vi "TC.vi"() -> ()   [LabVIEW 2019]
uses:
  Lib/Lib.llb/CS mode.ctl
  Lib/Lib.llb/R.ctl
  Lib/Lib.llb/T.ctl
  Lib/Lib.llb/Calibrations.ctl
  Lib/Lib.llb/CS.lvclass
  Lib/Lib.llb/PID Settings.ctl
  Lib/Lib.llb/AVS_exc_n_ranges.ctl
  Lib/Lib.llb/AVS_excitation.ctl
  Lib/Lib.llb/AVS47_range.ctl
  Lib/Lib.llb/Ch descriptions.ctl
  Lib/Lib.llb/Cursor Controls.ctl
  Lib/Lib.llb/DataArray.ctl
  Lib/Lib.llb/Unit.ctl
  Lib/Lib.llb/Control 6.ctl
  Lib/Lib.llb/Control 4.ctl
  Lib/Lib.llb/Control 8.ctl
  Lib/Lib.llb/VI FPO Ref.ctl
  Lib/support/Class ID ENUM.ctl
  <userlib>/_OpenG.lib/lvdata/lvdata.llb/Type Descriptor Enumeration__ogtk.ctl
  <userlib>/_OpenG.lib/lvdata/lvdata.llb/Refnum Subtype Enum__ogtk.ctl
  <userlib>/_OpenG.lib/lvdata/lvdata.llb/Waveform Subtype Enum__ogtk.ctl
  Lib/Lib.llb/LV Data cluster.ctl
  <userlib>/LevyLab/Instrument Framework/Instrument/Typedefs/PublicEvents--Instrument.MessageFromProcess.ctl
  <userlib>/LevyLab/RemoteControl/RemoteControl/Typedefs/Message--Cluster.ctl
  shared/Inst.TC/Inst.TC.lvclass
  C:/Program Files (x86)/National Instruments/LabVIEW 2019/vi.lib/JKI/JKI SMO/SMO/SMO.lvclass
  C:/Program Files (x86)/National Instruments/LabVIEW 2019/user.lib/LevyLab/Instrument Framework/Instrument/Instrument.lvclass
  Lib/Lib.llb/Action.ctl
  <userlib>/LevyLab/Instrument Framework/Instrument Types/Cryostat/Typedefs/setHeater--cluster.ctl
  shared/Inst.TC/Typedefs/Inst.TC.Commands--Enum.ctl
  Lib/Lib.llb/TCS.lvclass
  C:/Users/ansom/Documents/Girthub/Leiden-FP-and-TC/src/TC/1. Sources/Lib/Lib.llb/CS.lvclass
  Lib/Lib.llb/QCS.lvclass
  Lib/Lib.llb/CS Emulation.lvclass
  Lib/Lib.llb/PCS.lvclass
  Lib/Lib.llb/Byte Params.ctl
  8b3f8898-ff02-46d6-8412-899a53daf4d1.vi
  <vilib>/JDP Science/JSONtext/JSON text to Variant.vi
  <userlib>/LevyLab/Instrument Framework/Instrument/API/Instrument.sendMessageToProcess (string).vi
  <vilib>/JDP Science/JSONtext/LVClass Serializer/JSONtext LVClass Serializer.lvclass
  Lib/Lib.llb/MView.lvlib
  <userlib>/LevyLab/Instrument Framework/Instrument Types/Cryostat/Instrument.Cryostat.lvclass
  <vilib>/JKI/JKI SMO/SMO/SMO.lvclass
  <userlib>/LevyLab/Instrument Framework/Instrument/Instrument.lvclass
  C:/Program Files (x86)/National Instruments/LabVIEW 2019/user.lib/LevyLab/Instrument Framework/Instrument Types/Cryostat/Instrument.Cryostat.lvclass
  <userlib>/LevyLab/RemoteControl/RemoteControl/RemoteControl.lvclass
panel:
  out "R Array":dbl[](array[numeric])
  out "_SetControl":T1
  out "ControlNames":string[](array[string])
  out "VIRef":T2 {"Array DataType" format="%.0x"; "WaveForm Type" format="%.0x"; "RefNum Type" format="%.0x"; "DataType" format="%.0x"}
  out "VI called?":bool=TRUE
  out "Error code":u8
  out "_zBridgeSetNr":u8 caption="zBridge set nr."
  out "_zBridgeDll":path=path "C:/Users/Sasha/Dropbox/Labview/LC Software/ImpSoft-V5.2.2-multithreaded/ImpBridgeLabview/ImpBridgeDll.dll"
  in  "_String":string="^ Click the Run button to start the program "
  in  "Top Toolbar":enum32{"Page 1", "Page 2"}(tab)
  in  "Load config":bool
  in  "Start":bool
  in  "Load Data":bool
  in  "Pause":bool
  in  "Stop":bool
  in  "Copy to Clipboard":bool
  in  "Save config":bool
  in  "Clear all plots":bool
  in  "ColorBox":enum32{"Page 1", "Page 2"}(tab)
  in  "Colors":picture
  out "Color":u32(colorbox)
  in  "Graph-open popup":bool
  out "_CalibFilesPath":path=path "C:/avs-47/aaaa"
  out "_LogFilesPath":path
  out "_AVS_VISA":refnum<visa-resource-name>="COM3"
  in  "Minimize UI 2":bool
  out "VI Version":string="TC" caption="V"
  in  "Minimize UI 1":bool
  in  "Main Panel":enum32{"AVS"}(tab)
  in  "Graph Controls Bar":enum32{"Page 1"}(tab)
  in  "Mode Buttons":T7
  in  "Erase all":bool
  in  "Plot-Save All":bool
  in  "Plot-save-screen":bool
  in  "Channels Panel":T8(tab)=enum."All"
  out "T0":dbl=nan caption="T" format="%#.2p"
  out "R0":dbl caption="R" format="%.3p"
  out "R-Plot 0":cluster{dbl[], dbl[]}(graph) caption="R-Plot"
  out "T1":dbl=nan caption="T" format="%#.2p"
  out "R1":dbl caption="R" format="%.3p"
  out "R-Plot 1":cluster{dbl[], dbl[]}(graph) caption="R-Plot"
  out "T2":dbl=nan caption="T" format="%#.2p"
  out "R2":dbl caption="R" format="%.3p"
  out "R-Plot 2":cluster{dbl[], dbl[]}(graph) caption="R-Plot"
  out "T3":dbl=nan caption="T" format="%#.2p"
  out "R3":dbl caption="R" format="%.3p"
  out "R-Plot 3":cluster{dbl[], dbl[]}(graph) caption="R-Plot"
  out "T4":dbl=nan caption="T" format="%#.2p"
  out "R4":dbl caption="R" format="%.3p"
  out "R-Plot 4":cluster{dbl[], dbl[]}(graph) caption="R-Plot"
  out "T5":dbl=nan caption="T" format="%#.2p"
  out "R5":dbl caption="R" format="%.3p"
  out "R-Plot 5":cluster{dbl[], dbl[]}(graph) caption="R-Plot"
  out "T6":dbl=nan caption="T" format="%#.2p"
  out "R6":dbl caption="R" format="%.3p"
  out "R-Plot 6":cluster{dbl[], dbl[]}(graph) caption="R-Plot"
  out "T7":dbl=nan caption="T" format="%#.2p"
  out "R7":dbl caption="R" format="%.3p"
  out "R-Plot 7":cluster{dbl[], dbl[]}(graph) caption="R-Plot"
  out "T8":dbl=nan caption="T" format="%#.2p"
  out "R8":dbl caption="R" format="%.3p"
  out "R-Plot 8":cluster{dbl[], dbl[]}(graph) caption="R-Plot"
  out "T9":dbl=nan caption="T" format="%#.2p"
  out "R9":dbl caption="R" format="%.3p"
  out "R-Plot 9":cluster{dbl[], dbl[]}(graph) caption="R-Plot"
  out "T Cluster":T9 {"T9" format="%.2p"; "T8" format="%.2p"; "T7" format="%.2p"; "T6" format="%.2p"; "T5" format="%.2p"; "T4" format="%.2p"; "T3" format="%.2p"; "T2" format="%.2p"; "T1" format="%.2p"; "T0" format="%.2p"}
  in  "Sensor Names":T10={"AVS Name 0"="C_still", "AVS Name 1"="3K", "AVS Name 2"="Still", "AVS Name 3"="50mK", "AVS Name 4"="MC", "AVS Name 5"="MC", "AVS Name 6"="MC", "AVS Name 7"="", "AVS Name 8"="", "AVS Name 9"=""}
  in  "Edit Calibrations":T11
  in  "Sensor Calibrations":T12 {"Sensor 10" items=["PT100", "PT1000", "RuO2 2k", "Emulation R", "PT 1000", "RuO2-10K-NEW", "RuO2-10K", "RuO2-1k5", "TT-1338", "TT-1340", "TT-1342", "TT-1346", "TT-1349", "TT-1392", "CMN-187", "testCMN", "No Calibration"]; "Sensor 9" items=["PT100", "PT1000", "RuO2 2k", "Emulation R", "PT 1000", "RuO2-10K-NEW", "RuO2-10K", "RuO2-1k5", "TT-1338", "TT-1340", "TT-1342", "TT-1346", "TT-1349", "TT-1392", "CMN-187", "testCMN", "No Calibration"]; "Sensor 8" items=["PT100", "PT1000", "RuO2 2k", "Emulation R", "PT 1000", "RuO2-10K-NEW", "RuO2-10K", "RuO2-1k5", "TT-1338", "TT-1340", "TT-1342", "TT-1346", "TT-1349", "TT-1392", "CMN-187", "testCMN", "No Calibration"]; "Sensor 7" items=["PT100", "PT1000", "RuO2 2k", "Emulation R", "PT 1000", "RuO2-10K-NEW", "RuO2-10K", "RuO2-1k5", "TT-1338", "TT-1340", "TT-1342", "TT-1346", "TT-1349", "TT-1392", "CMN-187", "testCMN", "No Calibration"]; "Sensor 6" items=["PT100", "PT1000", "RuO2 2k", "Emulation R", "PT 1000", "RuO2-10K-NEW", "RuO2-10K", "RuO2-1k5", "TT-1338", "TT-1340", "TT-1342", "TT-1346", "TT-1349", "TT-1392", "CMN-187", "testCMN", "No Calibration"]; "Sensor 5" items=["PT100", "PT1000", "RuO2 2k", "Emulation R", "PT 1000", "RuO2-10K-NEW", "RuO2-10K", "RuO2-1k5", "TT-1338", "TT-1340", "TT-1342", "TT-1346", "TT-1349", "TT-1392", "CMN-187", "testCMN", "No Calibration"]; "Sensor 4" items=["PT100", "PT1000", "RuO2 2k", "Emulation R", "PT 1000", "RuO2-10K-NEW", "RuO2-10K", "RuO2-1k5", "TT-1338", "TT-1340", "TT-1342", "TT-1346", "TT-1349", "TT-1392", "CMN-187", "testCMN", "No Calibration"]; "Sensor 3" items=["PT100", "PT1000", "RuO2 2k", "Emulation R", "PT 1000", "RuO2-10K-NEW", "RuO2-10K", "RuO2-1k5", "TT-1338", "TT-1340", "TT-1342", "TT-1346", "TT-1349", "TT-1392", "CMN-187", "testCMN", "No Calibration"]; "Sensor 2" items=["PT100", "PT1000", "RuO2 2k", "Emulation R", "PT 1000", "RuO2-10K-NEW", "RuO2-10K", "RuO2-1k5", "TT-1338", "TT-1340", "TT-1342", "TT-1346", "TT-1349", "TT-1392", "CMN-187", "testCMN", "No Calibration"]; "Sensor 1" items=["PT100", "PT1000", "RuO2 2k", "Emulation R", "PT 1000", "RuO2-10K-NEW", "RuO2-10K", "RuO2-1k5", "TT-1338", "TT-1340", "TT-1342", "TT-1346", "TT-1349", "TT-1392", "CMN-187", "testCMN", "No Calibration"]}
  out "Units":T13
  out "R Cluster":T14={"R0"=0.0, "R1"=0.0, "R2"=-0.0, "R3"=0.0, "R4"=0.0, "R5"=0.0, "R6"=0.0, "R7"=0.0, "R8"=0.0, "R9"=0.0} {"R9" format="%.3p"; "R8" format="%.3p"; "R7" format="%.3p"; "R6" format="%.3p"; "R5" format="%.3p"; "R4" format="%.3p"; "R3" format="%.3p"; "R2" format="%.3p"; "R1" format="%.3p"; "R0" format="%.3p"}
  in  "AVS Scan Parameters":enum32{"Page 1", "Page 2"}(tab)
  in  "AVS Exc&Ranges":T15={"Excitation 0"=4, "Excitation 1"=4, "Excitation 2"=3, "Excitation 3"=3, "Excitation 4"=3, "Excitation 5"=3, "Excitation 6"=3, "Excitation 7"=3, "Range 0"=5, "Range 1"=5, "Range 2"=5, "Range 3"=5, "Range 4"=5, "Range 5"=5, "Range 6"=5, "Range 7"=5} {"Range 7" items=["n.a."=-1, "open"=0, "2 Ohm"=1, "20 Ohm"=2, "200 Ohm"=3, "2k Ohm"=4, "20k Ohm"=5, "200k Ohm"=6, "2M Ohm"=7]; "Range 6" items=["n.a."=-1, "open"=0, "2 Ohm"=1, "20 Ohm"=2, "200 Ohm"=3, "2k Ohm"=4, "20k Ohm"=5, "200k Ohm"=6, "2M Ohm"=7]; "Range 5" items=["n.a."=-1, "open"=0, "2 Ohm"=1, "20 Ohm"=2, "200 Ohm"=3, "2k Ohm"=4, "20k Ohm"=5, "200k Ohm"=6, "2M Ohm"=7]; "Range 4" items=["n.a."=-1, "open"=0, "2 Ohm"=1, "20 Ohm"=2, "200 Ohm"=3, "2k Ohm"=4, "20k Ohm"=5, "200k Ohm"=6, "2M Ohm"=7]; "Range 3" items=["n.a."=-1, "open"=0, "2 Ohm"=1, "20 Ohm"=2, "200 Ohm"=3, "2k Ohm"=4, "20k Ohm"=5, "200k Ohm"=6, "2M Ohm"=7]; "Range 2" items=["n.a."=-1, "open"=0, "2 Ohm"=1, "20 Ohm"=2, "200 Ohm"=3, "2k Ohm"=4, "20k Ohm"=5, "200k Ohm"=6, "2M Ohm"=7]; "Range 1" items=["n.a."=-1, "open"=0, "2 Ohm"=1, "20 Ohm"=2, "200 Ohm"=3, "2k Ohm"=4, "20k Ohm"=5, "200k Ohm"=6, "2M Ohm"=7]; "Range 0" items=["n.a."=-1, "open"=0, "2 Ohm"=1, "20 Ohm"=2, "200 Ohm"=3, "2k Ohm"=4, "20k Ohm"=5, "200k Ohm"=6, "2M Ohm"=7]; "Excitation 7" items=["none", "3 µV", "10 µV", "30 µV", "100 µV", "300 µV", "1 mV", "3 mV"]; "Excitation 6" items=["none", "3 µV", "10 µV", "30 µV", "100 µV", "300 µV", "1 mV", "3 mV"]; "Excitation 5" items=["none", "3 µV", "10 µV", "30 µV", "100 µV", "300 µV", "1 mV", "3 mV"]; "Excitation 4" items=["none", "3 µV", "10 µV", "30 µV", "100 µV", "300 µV", "1 mV", "3 mV"]; "Excitation 3" items=["none", "3 µV", "10 µV", "30 µV", "100 µV", "300 µV", "1 mV", "3 mV"]; "Excitation 2" items=["none", "3 µV", "10 µV", "30 µV", "100 µV", "300 µV", "1 mV", "3 mV"]; "Excitation 1" items=["none", "3 µV", "10 µV", "30 µV", "100 µV", "300 µV", "1 mV", "3 mV"]; "Excitation 0" items=["none", "3 µV", "10 µV", "30 µV", "100 µV", "300 µV", "1 mV", "3 mV"]}
  out "zBridge.Scan Phase":T18
  out "zBridge params":T19
  out "uPlots":T20
  out "zBridge.Active Channels":T21={"active Channel 0"=TRUE, "active Channel 1"=TRUE, "active Channel 2"=TRUE, "active Channel 3"=FALSE, "active Channel 4"=FALSE, "active Channel 5"=FALSE, "active Channel 6"=FALSE, "active Channel 7"=FALSE, "active Channel 8"=FALSE, "active Channel 9"=FALSE}
  out "Waveform Chart":T22(graph)
  in  "_CS_Address":u32
  in  "Edit calibration":bool
  in  "Convert R-T":bool
  out "T7":dbl caption="T=" format="%#.2p"
  in  "QuickR":dbl caption="R=" format="%_6g"
  in  "_QuickConvertCal":u16(ring) items=["PT100", "PT1000", "RuO2 2k", "Emulation R", "PT 1000", "RuO2-10K-NEW", "RuO2-10K", "RuO2-1k5", "TT-1338", "TT-1340", "TT-1342", "TT-1346", "TT-1349", "TT-1392", "CMN-187", "testCMN", "No Calibration"]
  out "_CSMode1List[i]":T23[](array[typedef]) caption="I_list[i]" min=-1.0
  out "CS.Automode Current":T23[](array[typedef]) min=-1.0
  in  "Lower Panel":enum32{"Page 1", "Page 2"}(tab)
  in  "Data History/RT Settings":enum32{"History", "Settings"}(tab)=enum."Settings"
  out "AVS names small":T10={"AVS Name 0"="3K", "AVS Name 1"="Still", "AVS Name 2"="50 mK", "AVS Name 3"="MC", "AVS Name 4"="MC", "AVS Name 5"="", "AVS Name 6"="", "AVS Name 7"="", "AVS Name 8"="", "AVS Name 9"=""}
  out "zBridge.Active channel":T24
  out "Small T Cluster":T25 caption="T" {"T0" format="%#.2p"; "T1" format="%#.2p"; "T2" format="%#.2p"; "T3" format="%#.2p"; "T4" format="%#.2p"; "T5" format="%#.2p"; "T6" format="%#.2p"; "T7" format="%#.2p"; "T8" format="%#.2p"; "T9" format="%#.2p"}
  out "Small R Cluster":T26 caption="R" {"R0" format="%#_5p"; "R1" format="%#_5p"; "R2" format="%#_5p"; "R3" format="%#_5p"; "R4" format="%#_5p"; "R5" format="%#_5p"; "R6" format="%#_5p"; "R7" format="%#_5p"; "R8" format="%#_5p"; "R9" format="%#_5p"}
  out "Time":dbl format="%<%X\n%x>T"
  in  "Runtime Settings":T27={"Read AVS channels from"=0, "Last Channel"=7, "Delay Between Scans"=0, "Stabilisation Delay"=5.0, "Averages"=2, "Data Memory"=25000, "Filter Graphs"=FALSE, "Y_min"=0.0, "Y_max"=2000000.0, "Plot type"=enum."T vs Time", "Allow neg R"=TRUE, "Miniplot Time"=30.0} {"Miniplot Time" min=0.0; "Delay Between Scans" format="%.0f s"; "Averages" min=1 max=1000; "Stabilisation Delay" min=0.5; "Last Channel" min=0 max=7 step=1; "Read AVS channels from" min=0 max=7 step=1; "Y_max" format="%#_6f"; "Y_min" min=0.0 format="%#_6f"; "Data Memory" min=3 max=50000}
  out "CS.Current Value":dbl[](array[numeric])
  in  "Data Array":T28=[{"R"=[], "T"=[], "Time"=[]}, {"R"=[0.0, 2.0], "T"=[], "Time"=[]}]
  out "T Array":dbl[](array[numeric])
  in  "_ScanData":dbl[](array[numeric])
  out "_I3SetPnt":dbl
  out "_CurrentsChanged":bool
  in  "_AVSRanges":T29={"Excitationl 0"=5, "Excitation 1"=5, "Excitation 2"=5, "Excitation 3"=5, "Excitation 4"=5, "Excitation 5"=5, "Excitation 6"=5, "Excitation 7"=5} caption="Ranges" {"Excitation 7" items=["n.a."=-1, "open"=0, "2 Ohm"=1, "20 Ohm"=2, "200 Ohm"=3, "2k Ohm"=4, "20k Ohm"=5, "200k Ohm"=6, "2M Ohm"=7]; "Excitation 6" items=["n.a."=-1, "open"=0, "2 Ohm"=1, "20 Ohm"=2, "200 Ohm"=3, "2k Ohm"=4, "20k Ohm"=5, "200k Ohm"=6, "2M Ohm"=7]; "Excitation 5" items=["n.a."=-1, "open"=0, "2 Ohm"=1, "20 Ohm"=2, "200 Ohm"=3, "2k Ohm"=4, "20k Ohm"=5, "200k Ohm"=6, "2M Ohm"=7]; "Excitation 4" items=["n.a."=-1, "open"=0, "2 Ohm"=1, "20 Ohm"=2, "200 Ohm"=3, "2k Ohm"=4, "20k Ohm"=5, "200k Ohm"=6, "2M Ohm"=7]; "Excitation 3" items=["n.a."=-1, "open"=0, "2 Ohm"=1, "20 Ohm"=2, "200 Ohm"=3, "2k Ohm"=4, "20k Ohm"=5, "200k Ohm"=6, "2M Ohm"=7]; "Excitation 2" items=["n.a."=-1, "open"=0, "2 Ohm"=1, "20 Ohm"=2, "200 Ohm"=3, "2k Ohm"=4, "20k Ohm"=5, "200k Ohm"=6, "2M Ohm"=7]; "Excitation 1" items=["n.a."=-1, "open"=0, "2 Ohm"=1, "20 Ohm"=2, "200 Ohm"=3, "2k Ohm"=4, "20k Ohm"=5, "200k Ohm"=6, "2M Ohm"=7]; "Excitationl 0" items=["n.a."=-1, "open"=0, "2 Ohm"=1, "20 Ohm"=2, "200 Ohm"=3, "2k Ohm"=4, "20k Ohm"=5, "200k Ohm"=6, "2M Ohm"=7]}
  out "_CSClassRef":refnum<class "CS.lvclass">
  in  "CS Indicators Panel":enum32{"Page 1", "Page 2"}(tab)
  out "CS.Automode 0":bool
  out "CS.Automode 1":bool
  out "QCS. I0 Mapping":T30(ring) caption="Output to"
  in  "uA 0":u32
  in  "CS Cannel Names":T31={"CS Name 0"="N.C.", "CS Name 1"="3K", "CS Name 2"="Still", "CS Name 3"="MC"}
  out "I0":T32={"uA"="000", "ON"=FALSE, "Gated"=FALSE, "current flows"=FALSE, "Error"=FALSE} caption="Ch0 -"
  in  "uA 3":u32
  in  "uA 2":u32
  in  "uA 1":u32
  out "CS.Automode 3":bool
  out "CS.Automode 2":bool
  out "I3":T32={"uA"="000", "ON"=FALSE, "Gated"=FALSE, "current flows"=FALSE, "Error"=FALSE} caption="Chn 3"
  out "I2":T32={"uA"="000", "ON"=FALSE, "Gated"=FALSE, "current flows"=FALSE, "Error"=FALSE} caption="Chn 2"
  out "I1":T32={"uA"="000", "ON"=FALSE, "Gated"=FALSE, "current flows"=FALSE, "Error"=FALSE} caption="Chn 1"
  out "_ExtVIReference":refnum<vi>
  out "Small I":cluster{"I1":dbl, "I2":dbl, "I3":dbl, "I4":dbl} caption="I" {"I1" format="%#.2f"; "I2" format="%#.2p"; "I3" format="%#.2p"; "I4" format="%#.2p"}
  out "CS.Actual Current":dbl[](array[numeric])
  in  "Save Data 2":bool
  in  "Show PID graph?":bool
  in  "Set Color":bool
  out "_ZBridgeUnit":string caption="Unit"
  out "_zBridgeParText":string caption="zBridge params/Error"
  out "_CurCalibrations":T33
  out "_LMBDown":bool
  in  "Side Panel":T34(tab)
  in  "Reload Calibrations":bool
  in  "zBridge settings":bool
  out "CS.ID":string caption="ID"
  out "CS status":errorcluster
  out "General Error":errorcluster caption="General status"
  in  "Bridge settings":T35={"Bridge Type"=enum."AVS47A (GPIB interface)", "AVS RS232 Port"="COM5", "AVS GPIB Address"="GPIB0::20::INSTR", "Calibrations Folder"=path "C:/LC Data/Calibrations", "Picobus Delay"=1, "Sync to ADC"=enum."TRUE"} {"Picobus Delay" max=1000000 step=1}
  in  "CS Settings":T36={"TCS RS232 Port"="COM1", "TCS_Imax"=5, "CS type"=enum."TCS", "CS.QCS Device Nr"=0}
  in  "Data Logging Settings":T37={"Log Files Folder"=path "C:/LC Data/Data", "Log Files Name"="LogAVS", "Automode Files Name"="calibration", "Filenames Suffix"="_%Y-%m-%d-%H-%M-%S", "Delimeter"="\t", "New File Interval"=7, "New File Interval Units"=enum."Days", "Date Format"="%Y-%m-%d %H:%M:%S", "External VI Path"=path "", "Query Description"=FALSE, "Run Description"="\n"}
  out "Bridge status":errorcluster
  in  "CS.QCS I0 Output":T38(ring) caption="Set Channel 0 output to"
  in  "CS.Mode":T39 caption="CS mode"
  out "_TimeOld":dbl format="%#_16g"
  in  "CS Modes Panel":T40(tab)=enum."Automatic 1"
  in  "CS.I3":T41={"Toggle ON/OFF"=FALSE, "Toggle Gated"=FALSE, "I"=0, "Range"=enum."x1 uA"} caption="Chn 3" {"I" max=100000 step=1}
  in  "CS.I2":T41={"Toggle ON/OFF"=FALSE, "Toggle Gated"=FALSE, "I"=0, "Range"=enum."x1 uA"} caption="Chn 2" {"I" max=100000 step=1}
  in  "CS.I1":T41={"Toggle ON/OFF"=FALSE, "Toggle Gated"=FALSE, "I"=0, "Range"=enum."x1 uA"} caption="Chn 1" {"I" max=100000 step=1}
  in  "CS.I0":T41={"Toggle ON/OFF"=FALSE, "Toggle Gated"=FALSE, "I"=0, "Range"=enum."x1 uA"} caption="Chn 0" {"I" max=100000 step=1}
  in  "CS.Mode1.PID Settings":T42={"FB on 2"=enum."3", "Proportional Gain"=3.0, "Integral Gain"=3.0, "Derivative Gain"=1.0, "Deadband"=0.1, "Feed Fwd Gain [uA/mK]"=0.0, "Integral Gain Bandwidth"=10.0, "Integral Gain Background"=1.0, "Current limit, [uA]"=1.0} {"Integral Gain Background" format="%#.6g"; "Integral Gain Bandwidth" format="%#.6g"; "Feed Fwd Gain [uA/mK]" format="%#.5g"; "Deadband" format="%#.5g"; "Derivative Gain" format="%#.6g"; "Integral Gain" format="%#.6g"; "Proportional Gain" format="%#.6g"; "Current limit, [uA]" format="%#.5g"}
  in  "CS.Mode1.Start":bool
  in  "CS.Mode1.List":T23[][](array[typedef]) min=-1.0
  out "CS.Mode1.PID Column":T43[](array[typedef])
  out "CS.Mode1.Row":T44[](array[typedef])=[TRUE, FALSE, FALSE, FALSE, FALSE, FALSE, FALSE, FALSE, FALSE, FALSE]
  out "CS.Mode1.PID Stabilized?":bool caption="SP reached?"
  out "CS.Mode1.PID Error":dbl=10.0 caption="Error" format="%#_6f"
  out "CS.Mode1.Slope":dbl caption="Slope" format="%#_3g %"
  out "CS.Mode1.Timer":dbl caption="Timer" format="%<%H:%M:%S>t"
  out "CS.Mode1.List:Count":i32=10 caption="/"
  out "CS.Mode1.List:Index":i32=10 caption="Point #"
  in  "CS.Mode1.Next":bool
  in  "CS.Mode1.Reset PID":bool
  in  "CS.Mode1.Auto Advance":bool=TRUE caption="Enable automatic sweeping/list iteration"
  in  "CS.Mode1.Settings":T45={"Bridge Channel"=0, "N averages"=10, "Delay Time"=10.0, "T stability"=0.3, "FB on"=enum."Temperature"} {"Delay Time" min=0.0 format="%#_g min"; "Bridge Channel" min=-1 max=9 step=1}
  in  "CS.Mode1.Call VI?":bool caption="Call Ext. VI"
  out "CS.Mode1.VI State":T46(ring) caption="- state"
  in  "CS.Mode1.Trigger all TC":bool caption="Trigger other running TC instances"
  in  "CS.Mode1.List:Prev":bool
  in  "CS.Mode1.List:Next":bool
  in  "CS.Mode1.List:To First":bool
  in  "CS.Mode1.List:Save":bool
  in  "CS.Mode1.List:Load":bool
  in  "CS.Mode1.Write To Log":bool
  in  "CS.Mode1.PID":cluster{"Enabled":bool}
  in  "CS.Mode1.List:Clear":bool
  in  "CS.Mode2.Settings":T47={"FB on"=enum."Temperature", "Bridge Channel"=0, "Hysteresis"=10} {"Hysteresis" max=100 format="%.0f %%"; "Bridge Channel" min=-1 max=9 step=1}
  in  "CS.Mode2.Start":bool
  in  "CS.Mode2.Add Row":bool
  in  "CS.Mode2.New Row":dbl[](array[numeric])=[0.0, 0.0, 0.0, 0.0, 0.0, 0.0] caption="New range" min=-1.0
  in  "CS.Mode2.List":dbl[][](array[numeric])=[[0.0, 0.0, 0.0, 0.0, 0.0, inf]] min=-1.0
  out "CS.Mode2.Row":T44[](array[typedef])=[TRUE, FALSE, FALSE, FALSE, FALSE, FALSE, FALSE, FALSE, FALSE, FALSE]
  in  "T Sweep":T48={"Start value"=200.0, "End value"=250.0, "Step"=10.0, "Current"=0.0, "I_next"=FALSE, "I_prev"=FALSE, "Interrrupt Sweep"=FALSE, "Start"=FALSE, "Boolean"=TRUE} {"Step" min=0.0; "End value" min=0.0; "Start value" min=0.0}
  # "Quick convert R->T:"
  # "Ohm"
  # "mK"
  # "Ch#"
  # "Miniplot"
  # "Channel parameters"
  # "Impedance"
  # "Unit"
  # "Type of sensor"
  # "T [mK]"
  # "Description"
  # "0"
  # "1"
  # "2"
  # "3"
  # "4"
  # "5"
  # "6"
  # "7"
  # "8"
  # "9"
  # "0"
  # "1"
  # "2"
  # "3"
  # "4"
  # "5"
  # "7"
  # "8"
  # "9"
  # "6"
  # "auto"
  # "auto"
  # "auto"
  # "auto"
  # "gated"
  # "gated"
  # "gated"
  # "gated"
  # "Status"
  # "Current source mode"
  # "Current source manual control"
  # "Current source automatic mode #1"
  # "Currents List"
  # "Settings"
  # "I0"
  # "I1"
  # "I2"
  # "I3"
  # "Status"
  # "On temperature stabilized"
  # "Current source automatic mode #2"
  # "Currents List"
  # "Settings"
  # "T0"
  # "T1"
  # "I0"
  # "I1"
  # "I2"
  # "I3"
  # "T0"
  # "T1"
  # "I0"
  # "I1"
  # "I2"
  # "I3"
  # "Ch3"
types:
  T1 = typedef "MView.lvlib/LV Data cluster.ctl" = cluster{"Name":string, "Scalar":string, "Array":string[][]}
  T2 = typedef "MView.lvlib/VI FPO Ref.ctl" = cluster{"Control Ref ID":refnum<vi>[], "Full Name":string[], "ClassID":T3[], "Short Name":string[], "DataType":T4[], "RefNum Type":T5[], "WaveForm Type":T6[], "Parent":i32[], "Array DataType":T4[], "Owning VI":refnum<vi>[], "Active?":bool[]}
  T3 = typedef "Class ID ENUM.ctl" = enum16{"<Null>", "1", "2", "Generic", "Decoration", "Text", "Control", "ColorBox", "Boolean", "RefNum", "Variant", "Path", "ListBox", "Table", "Array", "Picture", "ActiveXContainer", "Numeric", "Digital", "NamedNumeric", "ColorRamp", "Slide", "GraphOrChart", "WaveformChart", "WaveformGraph", "IntensityChart", "IntensityGraph", "String", "IOName", "ComboBox", "Cluster", "Panel", "Knob", "NumWithScale", "Ring", "Enum", "GObject", "Plot", "Cursor", "NumericText", "Scale", "ColorScale", "GraphScale", "ColorGraphScale", "TypedRefNum", "OldKnobScale", "MCListbox", "MeasureData", "BVTag", "DAQName", "VISAName", "IVIName", "SlideScale", "TabControl", "Page", "TabArrayTabControl", "ConPane", "57", "58", "59", "60", "61", "62", "63", "64", "SubPanel", "TreeControl", "67", "68", "69", "70", "71", "72", "73", "74", "75", "SplitterBar"}
  T4 = typedef "Type Descriptor Enumeration__ogtk.ctl" = enum8{"<Null>", "I8", "I16", "I32", "I64", "U8", "U16", "U32", "U64", "SGL", "DBL", "EXT", "CSG", "CDB", "CXT", "0x0F", "0x10", "0x11", "0x12", "0x13", "0x14", "Enum U8", "Enum U16", "Enum U32", "Enum U64", "SGL PQ", "DBL PQ", "EXT PQ", "CSG PQ", "CDB PQ", "CXT PQ", "0x1F", "0x20", "Boolean", "0x22", "0x23", "0x24", "0x25", "0x26", "0x27", "0x28", "0x29", "0x2A", "0x2B", "0x2C", "0x2D", "0x2E", "0x2F", "String", "0x31", "Path", "Pict", "0x34", "0x35", "0x36", "DAQ", "0x38", "0x39", "0x3A", "0x3B", "0x3C", "0x3D", "0x3E", "0x3F", "Array", "0x41", "0x42", "0x43", "0x44", "0x45", "0x46", "0x47", "0x48", "0x49", "0x4A", "0x4B", "0x4C", "0x4D", "0x4E", "0x4F", "Cluster", "0x51", "0x52", "Variant", "Waveform", "0x55", "0x56", "0x57", "0x58", "0x59", "0x5A", "0x5B", "0x5C", "0x5D", "0x5E", "Fixed Point", "0x60", "0x61", "0x62", "0x63", "0x64", "0x65", "0x66", "0x67", "0x68", "0x69", "0x6A", "0x6B", "0x6C", "0x6D", "0x6E", "0x6F", "Refnum", "0x71", "0x72", "Set Collection", "Map Collection"}
  T5 = typedef "Refnum Subtype Enum__ogtk.ctl" = enum8{"Generic", "Datalog File Refnum", "Byte Stream File Refnum", "Device Refnum", "Occurence Refnum", "TCP Connection Refnum", "VISA Refnum (Obsolete)", "Automation Renum", "VI Server Refnum", "Menu Refnum", "IVI Refnum (Obsolete)", "IMAQ Session", "0x0C", "Datasocket Refnum", "VISA Resource", "IVI Logical Name", "UDP Connection Refnum", "Notifier Refnum", "Queue Refnum", "IrDA Refnum", "Hardware Plugin Refnum", "Hardware Plugin Tag Refnum", "DAQmx Refnum", "Event Registration Refnum", ".NET Refnum", "User Event Refnum", "0x1A", "Event Callback", "0x1C", "0x1D", "LabVIEW Class Instance", "Bluetooth", "Data Value References", "RT FIFO", "TDM Streaming"}
  T6 = typedef "Waveform Subtype Enum__ogtk.ctl" = enum8{"<Not a Waveform Type>", "0x01", "Analog 16-bit signed", "Analog Double-Precision", "0x04", "Analog Single Precision", "Timestamp", "Digital Data", "Digital Waveform", "Dynamic Data", "Analog Extended-Precision", "Analog 8-bit unsigned", "Analog 16-bit unsigned", "Analog 32-bit unsigned", "Analog 8-bit signed", "Analog 32-bit signed", "Analog Complex Single-Precision", "Analog Complex Double-Precision", "Analog Complex Extended Precision", "Analog 64-bit signed", "Analog 64-bit unsigned"}
  T7 = typedef "Cursor Controls.ctl" = enum32{"No Selection", "Cursor mode", "Erase point", "Erase range"}
  T8 = enum32{"0", "1", "2", "3", "4", "5", "6", "7", "8", "9", "All", "PID loop"}
  T9 = typedef "T.ctl" = cluster{"T0":dbl, "T1":dbl, "T2":dbl, "T3":dbl, "T4":dbl, "T5":dbl, "T6":dbl, "T7":dbl, "T8":dbl, "T9":dbl}
  T10 = typedef "Ch descriptions.ctl" = cluster{"AVS Name 0":string, "AVS Name 1":string, "AVS Name 2":string, "AVS Name 3":string, "AVS Name 4":string, "AVS Name 5":string, "AVS Name 6":string, "AVS Name 7":string, "AVS Name 8":string, "AVS Name 9":string}
  T11 = cluster{"Boolean":bool, "Boolean 2":bool, "Boolean 3":bool, "Boolean 4":bool, "Boolean 5":bool, "Boolean 6":bool, "Boolean 7":bool, "Boolean 8":bool, "Boolean 9":bool, "Boolean 10":bool}
  T12 = typedef "Calibrations.ctl" = cluster{"Sensor 1":u16, "Sensor 2":u16, "Sensor 3":u16, "Sensor 4":u16, "Sensor 5":u16, "Sensor 6":u16, "Sensor 7":u16, "Sensor 8":u16, "Sensor 9":u16, "Sensor 10":u16}
  T13 = typedef "Unit.ctl" = cluster{"Value 0":string, "Value 1":string, "Value 2":string, "Value 3":string, "Value 4":string, "Value 5":string, "Value 6":string, "Value 7":string, "Value 8":string, "Value 9":string}
  T14 = typedef "R.ctl" = cluster{"R0":dbl, "R1":dbl, "R2":dbl, "R3":dbl, "R4":dbl, "R5":dbl, "R6":dbl, "R7":dbl, "R8":dbl, "R9":dbl}
  T15 = typedef "AVS_exc_n_ranges.ctl" = cluster{"Excitation 0":T16, "Excitation 1":T16, "Excitation 2":T16, "Excitation 3":T16, "Excitation 4":T16, "Excitation 5":T16, "Excitation 6":T16, "Excitation 7":T16, "Range 0":T17, "Range 1":T17, "Range 2":T17, "Range 3":T17, "Range 4":T17, "Range 5":T17, "Range 6":T17, "Range 7":T17}
  T16 = typedef "AVS_excitation.ctl" = i16
  T17 = typedef "AVS47_range.ctl" = i16
  T18 = cluster{"Value 0":dbl, "Value 1":dbl, "Value 2":dbl, "Value 3":dbl, "Value 4":dbl, "Value 5":dbl, "Value 6":dbl, "Value 7":dbl, "Value 8":dbl, "Value 9":dbl}
  T19 = cluster{"AVS Name 0":string, "AVS Name 1":string, "AVS Name 2":string, "AVS Name 3":string, "AVS Name 4":string, "AVS Name 5":string, "AVS Name 6":string, "AVS Name 7":string, "AVS Name 8":string, "AVS Name 9":string}
  T20 = cluster{"uPlot 0":cluster{dbl[], dbl[]}, "uPlot 1":cluster{dbl[], dbl[]}, "uPlot 2":cluster{dbl[], dbl[]}, "uPlot 3":cluster{dbl[], dbl[]}, "uPlot 4":cluster{dbl[], dbl[]}, "uPlot 5":cluster{dbl[], dbl[]}, "uPlot 6":cluster{dbl[], dbl[]}, "uPlot 7":cluster{dbl[], dbl[]}, "uPlot 8":cluster{dbl[], dbl[]}, "uPlot 9":cluster{dbl[], dbl[]}}
  T21 = cluster{"active Channel 0":bool, "active Channel 1":bool, "active Channel 2":bool, "active Channel 3":bool, "active Channel 4":bool, "active Channel 5":bool, "active Channel 6":bool, "active Channel 7":bool, "active Channel 8":bool, "active Channel 9":bool}
  T22 = cluster{"Ip":dbl, "Ii":dbl, "Id":dbl, "Iff":dbl, "I_tot":dbl}
  T23 = typedef "Control 4.ctl" = dbl
  T24 = cluster{"Boolean 5":bool, "Boolean 5":bool, "Boolean 5":bool, "Boolean 5":bool, "Boolean 5":bool, "Boolean 5":bool, "Boolean 5":bool, "Boolean 5":bool, "Boolean 5":bool, "Boolean 5":bool}
  T25 = cluster{"T0":dbl, "T1":dbl, "T2":dbl, "T3":dbl, "T4":dbl, "T5":dbl, "T6":dbl, "T7":dbl, "T8":dbl, "T9":dbl}
  T26 = cluster{"R0":dbl, "R1":dbl, "R2":dbl, "R3":dbl, "R4":dbl, "R5":dbl, "R6":dbl, "R7":dbl, "R8":dbl, "R9":dbl}
  T27 = cluster{"Read AVS channels from":i8, "Last Channel":i8, "Delay Between Scans":u32, "Stabilisation Delay":dbl, "Averages":u16, "Data Memory":u16, "Filter Graphs":bool, "Y_min":dbl, "Y_max":dbl, "Plot type":enum16{"R vs Time", "T vs Time"}, "Allow neg R":bool, "Miniplot Time":dbl}
  T28 = typedef "DataArray.ctl" = cluster{"R":dbl[], "T":dbl[], "Time":dbl[]}[]
  T29 = cluster{"Excitationl 0":i16, "Excitation 1":i16, "Excitation 2":i16, "Excitation 3":i16, "Excitation 4":i16, "Excitation 5":i16, "Excitation 6":i16, "Excitation 7":i16}
  T30 = enum16{"Chn 0", "Aux 0", "Aux 1", "Aux 2", "Aux 3"}
  T31 = cluster{"CS Name 0":string, "CS Name 1":string, "CS Name 2":string, "CS Name 3":string}
  T32 = cluster{"uA":string, "ON":bool, "Gated":bool, "current flows":bool, "Error":bool}
  T33 = cluster{"[0]":string, "[1]":string, "[2]":string, "[3]":string, "[4]":string, "[5]":string, "[6]":string, "[7]":string, "[8]":string, "[9]":string}
  T34 = enum32{"Devices Settings", "Current source control"}
  T35 = cluster{"Bridge Type":enum16{"AVS47A (GPIB interface)", "AVS47B (RS232 interface)", "AVS48SI (RS232 interface)", "AVS Emulation", "Impedance Bridge", "Disabled"}, "AVS RS232 Port":refnum<visa-resource-name>, "AVS GPIB Address":refnum<visa-resource-name>, "Calibrations Folder":path, "Picobus Delay":u32, "Sync to ADC":enum16{"FALSE", "TRUE"}}
  T36 = cluster{"TCS RS232 Port":refnum<visa-resource-name>, "TCS_Imax":i32, "CS type":enum16{"TCS", "QCS v1", "PCS (n.a.)", "CS Emulation", "Disabled"}, "CS.QCS Device Nr":u16}
  T37 = cluster{"Log Files Folder":path, "Log Files Name":string, "Automode Files Name":string, "Filenames Suffix":string, "Delimeter":string, "New File Interval":u32, "New File Interval Units":enum16{"Minutes", "Hours", "Days"}, "Date Format":string, "External VI Path":path, "Query Description":bool, "Run Description":string}
  T38 = enum16{"Channel 0", "Aux 0", "Aux 1", "Aux 2", "Aux 3"}
  T39 = typedef "CS mode.ctl" = enum16{"Manual", "Mode 1", "Mode2"}
  T40 = enum32{"Manual", "Automatic 1", "Automatic 2", "Automatic 3"}
  T41 = cluster{"Toggle ON/OFF":bool, "Toggle Gated":bool, "I":u32, "Range":enum8{"Auto", "x1 uA", "x10 uA", "x100 uA", "x1 mA"}}
  T42 = typedef "PID Settings.ctl" = cluster{"FB on 2":enum16{"0", "1", "2", "3"}, "Proportional Gain":dbl, "Integral Gain":dbl, "Derivative Gain":dbl, "Deadband":dbl, "Feed Fwd Gain [uA/mK]":dbl, "Integral Gain Bandwidth":dbl, "Integral Gain Background":dbl, "Current limit, [uA]":dbl}
  T43 = typedef "Control 8.ctl" = bool
  T44 = typedef "Control 6.ctl" = bool
  T45 = cluster{"Bridge Channel":i32, "N averages":i32, "Delay Time":dbl, "T stability":dbl, "FB on":enum16{"Resistance", "Temperature"}}
  T46 = enum32{"Bad", "Idle", "Run top level", "Running"}
  T47 = cluster{"FB on":enum16{"Resistance", "Temperature"}, "Bridge Channel":i32, "Hysteresis":u8}
  T48 = cluster{"Start value":dbl, "End value":dbl, "Step":dbl, "Current":dbl, "I_next":bool, "I_prev":bool, "Interrrupt Sweep":bool, "Start":bool, "Boolean":bool}
  T49 = cluster{"UpdateChannelInfo":refnum<user-event>, "UpdateValuesAVS":refnum<user-event>, "UpdateCalibrations":refnum<user-event>, "UpdateLogFilePath":refnum<user-event>, "TempStabilized":refnum<user-event>, "Reset PID loop":refnum<user-event>, "UpdateValuesZBridge":refnum<user-event>, "CS Automode":refnum<user-event>, "CallExtVI":refnum<user-event>, "Data Array":refnum<user-event>}
  T50 = cluster{"Config folder":path, "Config File":path, "Calibrations Folder":path, "zBridge dll":path, "Variables Library":path, "Inst.TC":refnum<class "Inst.TC.lvclass">}
  T51 = enum32{"Page Enabled", "Page Disabled", "Page Disabled & Grayed"}
  T52 = cluster{"error":bool, "code":i32, "source":string}
  T53 = typedef "Action.ctl" = enum16{"Init", "Write", "Read"}
  T54 = typedef "Instrument.Cryostat.lvclass/setHeater--cluster.ctl" = cluster{"current":dbl, "channel":i32}
  T55 = enum8{"Auto", "x1 uA", "x10 uA", "x100 uA", "x1 mA"}
  T56 = enum32{"No Selection", "Cursor mode", "Erase point", "Erase range"}
  T57 = enum16{"AVS47A (GPIB interface)", "AVS47B (RS232 interface)", "AVS48", "AVS Emulation", "Impedance Bridge", "Disabled"}
  T58 = enum16{"TCS", "QCS v1", "PCS (n.a.)", "CS Emulation", "Disabled"}
  T59 = cluster{"Cluster":cluster{"Time":dbl[], "T":dbl[]}, "Cluster":cluster{"Time":dbl[], "T":dbl[]}, "Cluster":cluster{"Time":dbl[], "T":dbl[]}, "Cluster":cluster{"Time":dbl[], "T":dbl[]}, "Cluster":cluster{"Time":dbl[], "T":dbl[]}, "Cluster":cluster{"Time":dbl[], "T":dbl[]}, "Cluster":cluster{"Time":dbl[], "T":dbl[]}, "Cluster":cluster{"Time":dbl[], "T":dbl[]}, "Cluster":cluster{"Time":dbl[], "T":dbl[]}, "Cluster":cluster{"Time":dbl[], "T":dbl[]}}
  T60 = enum32{"invalid app kind", "Development System", "Run Time System", "Student Edition", "Embedded LabVIEW", "Evaluation", "Custom"}
  T61 = enum16{"AVS47A (GPIB interface)", "AVS47B (RS232 interface)", "AVS48SI (RS232 interface)", "AVS Emulation", "Impedance Bridge", "Disabled"}
  T62 = typedef "Inst.TC.lvclass/PublicEvents--Cluster.ctl" = cluster{"MessageFromProcess":refnum<user-event>}
  T63 = typedef "Inst.TC.lvclass/Inst.TC.Commands--Enum.ctl" = enum16{"getTemperature", "getHeater", "setHeater"}
  T64 = cluster{"[0]":dbl, "[1]":dbl, "[2]":dbl, "[3]":dbl, "[4]":dbl, "[5]":dbl, "[6]":dbl, "[7]":dbl, "[8]":dbl, "[9]":dbl}
  T65 = cluster{"Temperature[0]":dbl, "Temperature[1]":dbl, "Temperature[2]":dbl, "Temperature[3]":dbl, "Temperature[4]":dbl, "Temperature[5]":dbl, "Temperature[6]":dbl, "Temperature[7]":dbl, "Temperature[8]":dbl, "Temperature[9]":dbl}
  T66 = cluster{"Current Time (double)":dbl, "R":dbl[], "T":dbl[]}
  T67 = typedef "File Info Record__ogtk.ctl" = cluster{"type":string, "creator":string, "permissions":i32, "data size":i32, "res size":i32, "creation date":u32, "modification date":u32, "bFolder":bool, "bInvisible":bool, "location":cluster{"vertical":i16, "horizontal":i16}, "owner":string, "group":string}
  T68 = cluster{"Units[0]":string, "Units[1]":string, "Units[2]":string, "Units[3]":string, "Units[4]":string, "Units[5]":string, "Units[6]":string, "Units[7]":string, "Units[8]":string, "Units[9]":string}
  T69 = cluster{"zBridge params[0]":string, "zBridge params[1]":string, "zBridge params[2]":string, "zBridge params[3]":string, "zBridge params[4]":string, "zBridge params[5]":string, "zBridge params[6]":string, "zBridge params[7]":string, "zBridge params[8]":string, "zBridge params[9]":string}
  T70 = cluster{"date/time string":string, "Value":dbl[], "Value":dbl[], "Value":dbl[]}
  T71 = typedef "imagedata.ctl" = cluster{"image type":i32, "image depth":i32, "image":u8[], "mask":u8[], "colors":u32[], "Rectangle":cluster{"left":i16, "top":i16, "right":i16, "bottom":i16}}
  T72 = typedef "LVPoint32TypeDef.ctl" = cluster{"Horizontal":i32, "Vertical":i32}
  T73 = cluster{"Shift":bool, "Ctrl":bool, "Alt":bool, "Cmd":bool, "Opt":bool}
  T74 = cluster{"Output Array":dbl[], "array w/ subset deleted":dbl[], "array w/ subset deleted":dbl[]}
  T75 = typedef "LVRectTypeDef.ctl" = cluster{"Left":i16, "Top":i16, "Right":i16, "Bottom":i16}
  T76 = typedef "Exc_n_Ranges.ctl" = cluster{"Excitationl 0":i16, "Excitation 1":i16, "Excitation 2":i16, "Excitation 3":i16, "Excitation 4":i16, "Excitation 5":i16, "Excitation 6":i16, "Excitation 7":i16, "Range 0":i16, "Range 1":i16, "Range 2":i16, "Range 3":i16, "Range 4":i16, "Range 5":i16, "Range 6":i16, "Range 7":i16}
  T77 = enum32{"HKEY_CLASSES_ROOT", "HKEY_CURRENT_USER", "HKEY_LOCAL_MACHINE", "HKEY_USERS", "HKEY_PERFORMANCE_DATA", "HKEY_CURRENT_CONFIG", "HKEY_DYN_DATA"}
  T78 = typedef "Byte Params.ctl" = enum8{"Active", "Channel Type", "Channel No", "Reference No", "RLC select", "Save Data", "L Inverted", "Menu Active"}
  T79 = typedef "LVPositionTypeDef.ctl" = cluster{"Left":i32, "Top":i32}
  T80 = cluster{"Range 0":i16, "Range 1":i16, "Range 2":i16, "Range 3":i16, "Range 4":i16, "Range 7":i16, "Range 5":i16, "Range 6":i16}
  T81 = cluster{"Range 0":i16, "Range 1":i16, "Range 2":i16, "Range 3":i16, "Range 4":i16, "Range 5":i16, "Range 6":i16, "Range 7":i16}
  T82 = cluster{"RANGE 0":u16, "RANGE 1":u16, "RANGE 2":u16, "RANGE 3":u16, "RANGE 4":u16, "RANGE 5":u16, "RANGE 6":u16, "RANGE 7":u16}
  T83 = typedef "LCR Channel parameters.ctl" = cluster{"Set_number":u8, "Set_char":u16, "Ch_number":u8, "Ch_type":u8, "Freq":dbl, "T_int":dbl, "I_exc":dbl, "V_exc":dbl, "SNR":dbl, "Vnoise":dbl, "P_diss":dbl}
  T84 = typedef "CS Data.ctl" = cluster{"Range":u8, "Current":dbl, "Current (string)":string, "On?":bool, "G?":bool, "I?":bool, "Err?":bool}
  T85 = typedef "TCS indicator.ctl" = cluster{"uA":string, " ON":bool, "Gated":bool, "current flows":bool, "Error":bool}
  T86 = cluster{"Toggle ON/OFF":bool, "Toggle Gated":bool}
  T87 = cluster{"Current":u32, "Range":enum16{"Auto", "x1 uA", "x10 uA", "x100 uA", "x1 mA"}}
  T88 = typedef "TCS manual control.ctl" = cluster{"Toggle ON/OFF":bool, "Toggle Gated":bool, "Current":u32, "Range":enum8{"Auto", "x1 uA", "x10 uA", "x100 uA", "x1 mA"}}
  T89 = cluster{"Status[0]":i32, "Status[1]":i32, "Status[2]":i32, "Status[3]":i32, "Status[4]":i32, "Status[5]":i32, "Status[6]":i32, "Status[7]":i32, "Status[8]":i32, "Status[9]":i32}
  T90 = cluster{"Active":bool, "Active":bool, "Active":bool, "Active":bool, "Active":bool, "Active":bool, "Active":bool, "Active":bool, "Active":bool, "Active":bool}
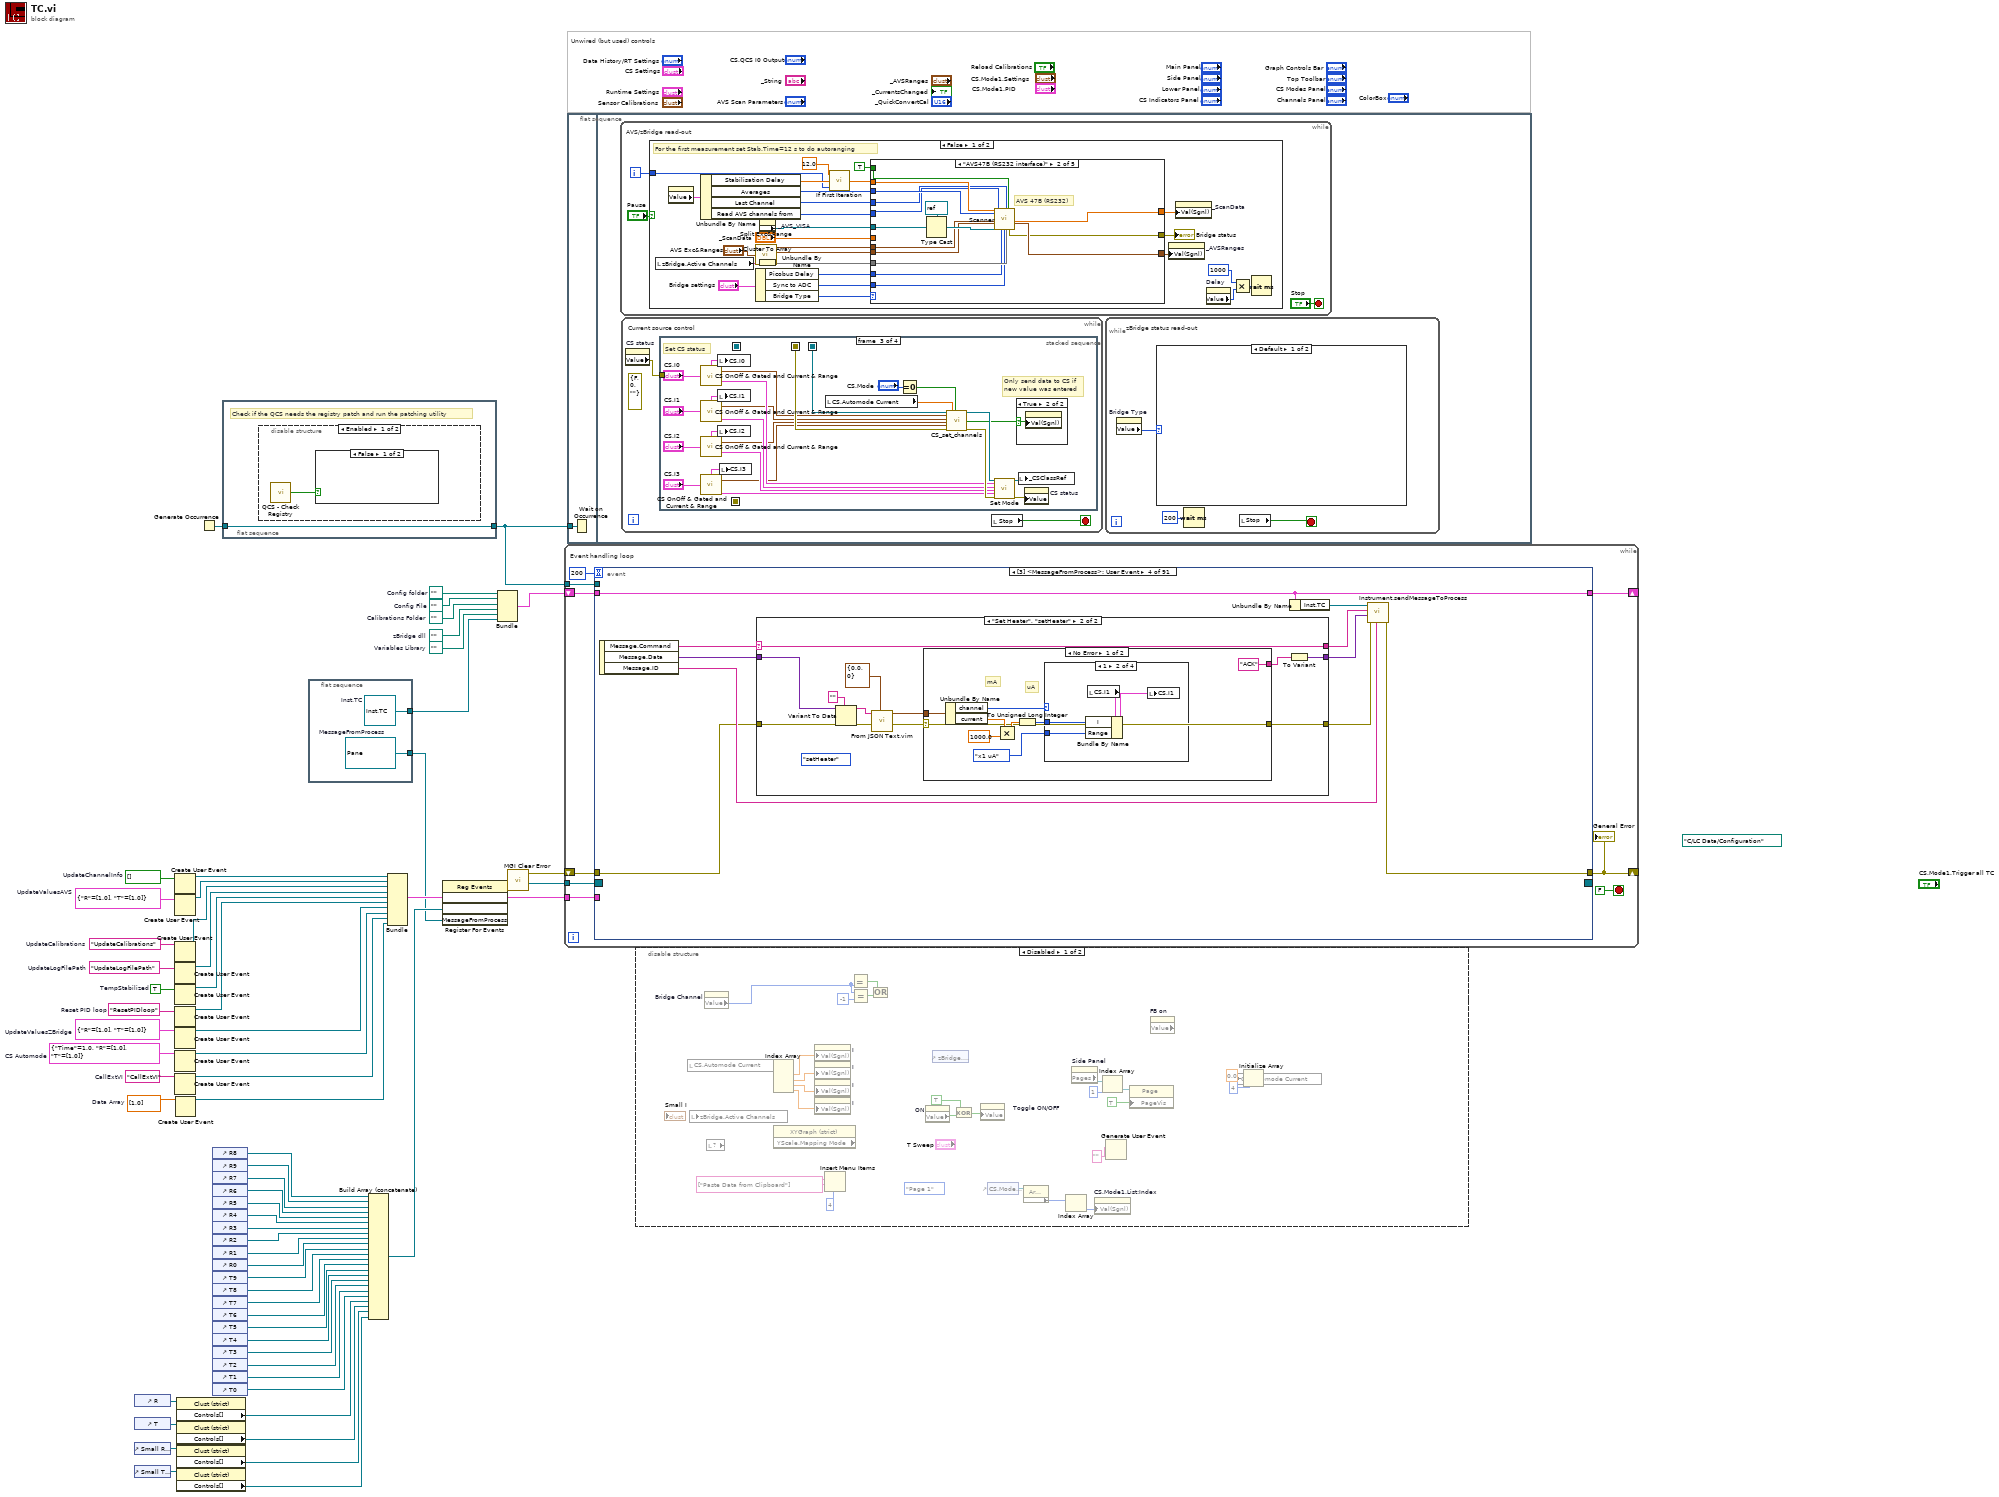
[diagram p0: block diagram]
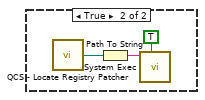
[diagram p2: hidden frame]
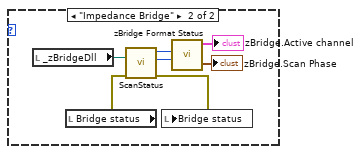
[diagram p4: hidden frame]
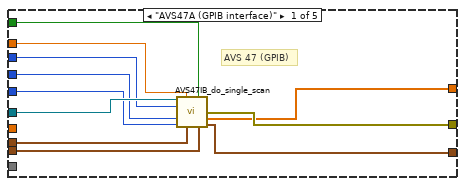
[diagram p5: hidden frame]
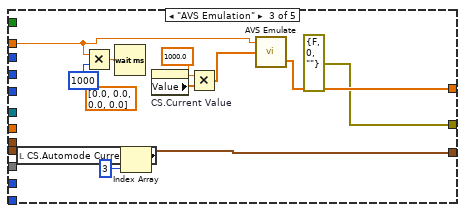
[diagram p6: hidden frame]
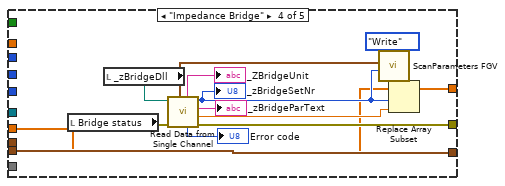
[diagram p7: hidden frame]
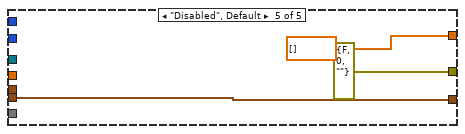
[diagram p8: hidden frame]
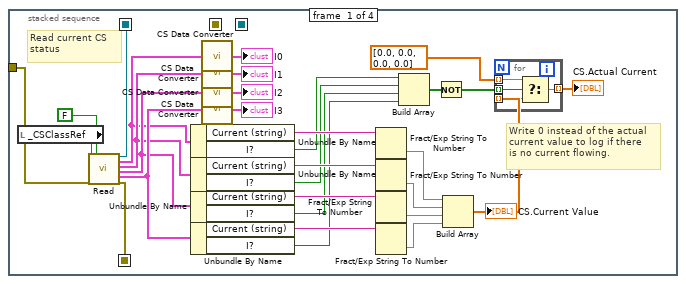
[diagram p10: hidden frame]
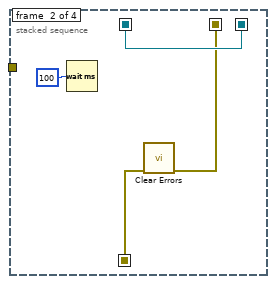
[diagram p11: hidden frame]
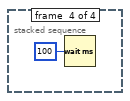
[diagram p13: hidden frame]
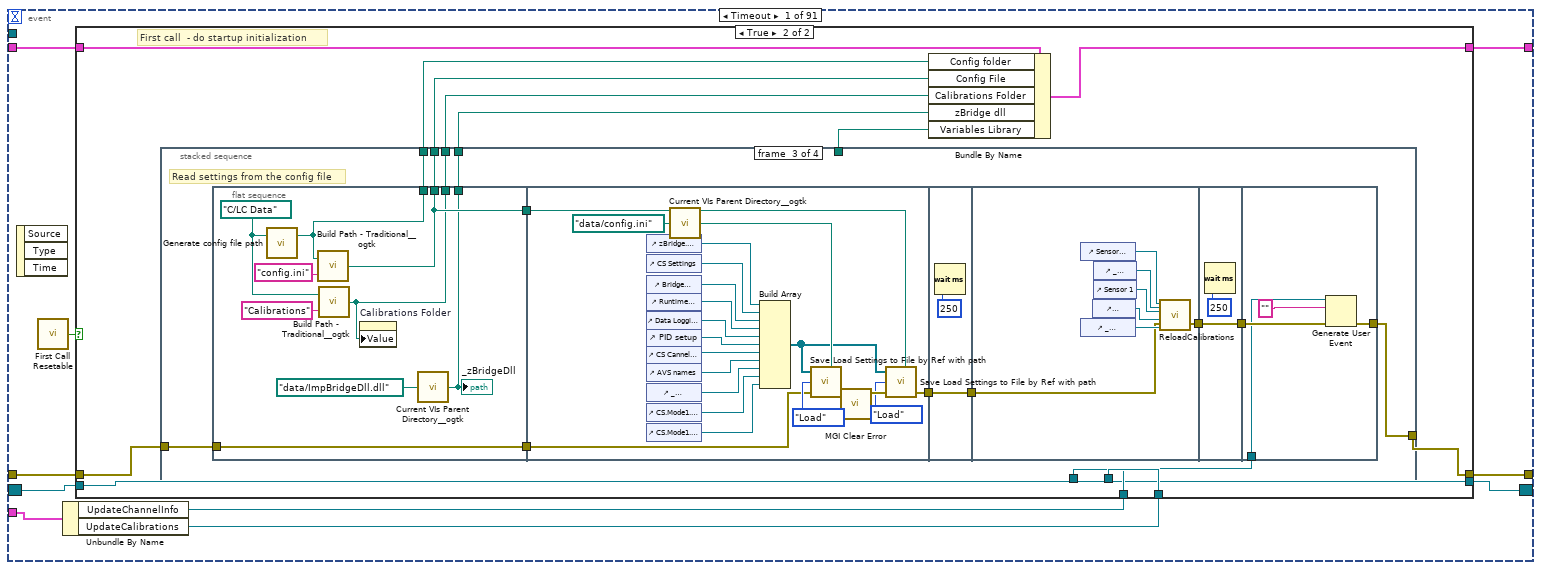
[diagram p15: hidden frame]
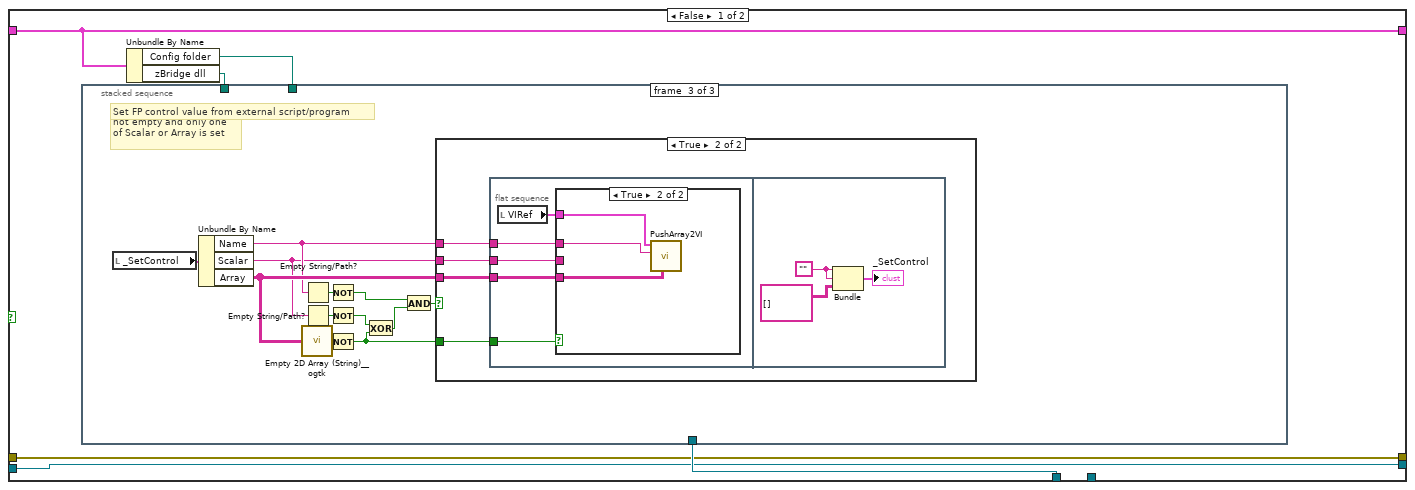
[diagram p16: hidden frame]
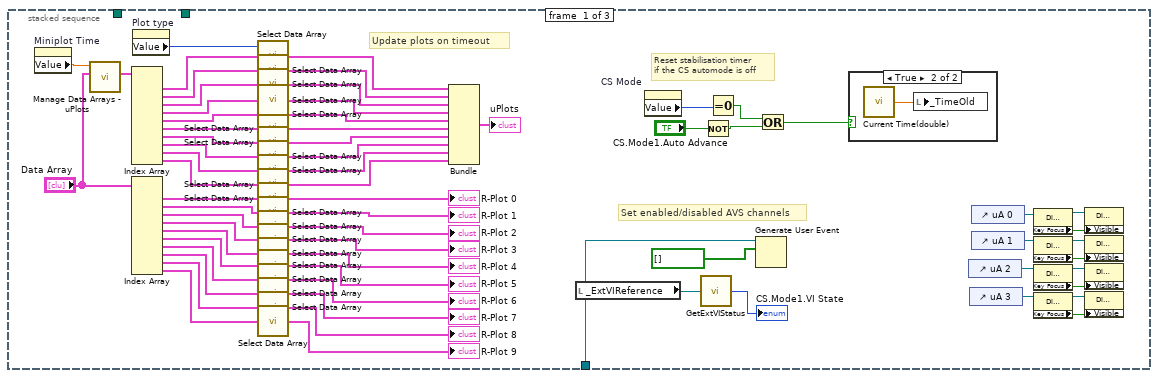
[diagram p17: hidden frame]
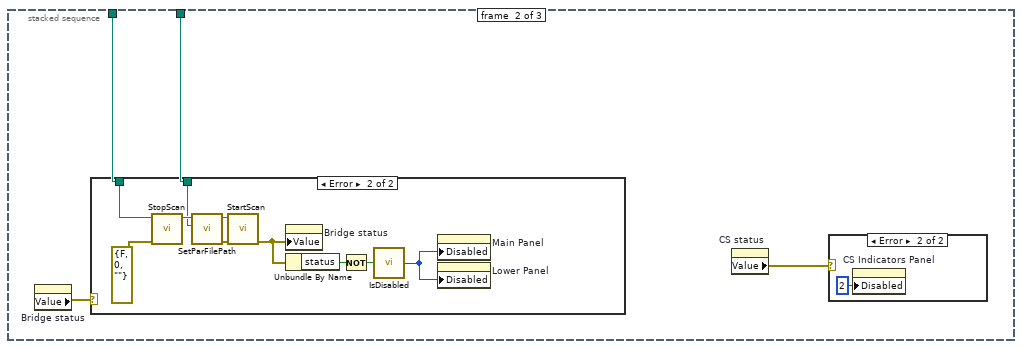
[diagram p19: hidden frame]
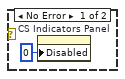
[diagram p20: hidden frame]
diagram:
  w32 = path ""  # Variables Library
  w33 = path ""  # zBridge dll
  w34 = path ""  # Calibrations Folder
  w35 = path ""  # Config File
  w37 = path ""  # Config folder
  (unwired) path "C:/LC Data/Configuration" ("Relative path (.)")
  w40 = dbl[] [1.0]  # Data Array
  w54 = "CallExtVI"  # CallExtVI
  w55 = bool[] []  # UpdateChannelInfo
  w56 = cluster{"Time":dbl, "R":dbl[], "T":dbl[]} {"Time"=1.0, "R"=[1.0], "T"=[1.0]}  # CS Automode
  w57 = cluster{"R":dbl[], "T":dbl[]} {"R"=[1.0], "T"=[1.0]}  # UpdateValuesAVS
  w58 = cluster{"R":dbl[], "T":dbl[]} {"R"=[1.0], "T"=[1.0]}  # UpdateValuesZBridge
  w59 = "ResetPIDloop"  # Reset PID loop
  w60 = TRUE  # TempStabilized
  w61 = "UpdateLogFilePath"  # UpdateLogFilePath
  w62 = "UpdateCalibrations"  # UpdateCalibrations
  # "Unwired (but used) controls"
  n1 = control-ref of="R"() -> (w31:refnum<vi>)
  n2 = control-ref of="T"() -> (w30:refnum<vi>)
  n3 = control-ref of="Small R Cluster"() -> (w6:refnum<vi>)
  n4 = control-ref of="Small T Cluster"() -> (w5:refnum<vi>)
  n5 = Create User Event(user event datatype=w55) -> (user event=w52:refnum<user-event>)  [unwired: 1 in, 1 out]
  n6 = Create User Event(user event datatype=w57) -> (user event=w51:refnum<user-event>)  [unwired: 1 in, 1 out]
  n7 = Create User Event(user event datatype=w62) -> (user event=w50:refnum<user-event>)  [unwired: 1 in, 1 out]
  n8 = Create User Event(user event datatype=w61) -> (user event=w49:refnum<user-event>)  [unwired: 1 in, 1 out]
  n9 = Create User Event ("TempStabilized")(user event datatype=w60) -> (user event=w48:refnum<user-event>)  [unwired: 1 in, 1 out]
  n10 = Create User Event(user event datatype=w59) -> (user event=w47:refnum<user-event>)  [unwired: 1 in, 1 out]
  n11 = Create User Event(user event datatype=w58) -> (user event=w46:refnum<user-event>)  [unwired: 1 in, 1 out]
  n12 = Create User Event(user event datatype=w56) -> (user event=w45:refnum<user-event>)  [unwired: 1 in, 1 out]
  n13 = Create User Event(user event datatype=w54) -> (user event=w44:refnum<user-event>)  [unwired: 1 in, 1 out]
  n14 = Create User Event(user event datatype=w40) -> (user event=w41:refnum<user-event>)  [unwired: 1 in, 1 out]
  n15 = property class="Clust (strict)"(reference=w31) -> ("Controls[]"=w9:refnum<vi>[])  [unwired: 1 in, 2 out]
  n16 = property class="Clust (strict)"(reference=w30) -> ("Controls[]"=w8:refnum<vi>[])  [unwired: 1 in, 2 out]
  n17 = property class="Clust (strict)"(reference=w6) -> ("Controls[]"=w4:refnum<vi>[])  [unwired: 1 in, 2 out]
  n18 = property class="Clust (strict)"(reference=w5) -> ("Controls[]"=w3:refnum<vi>[])  [unwired: 1 in, 2 out]
  n19 = Generate Occurrence() -> (w39:refnum<k4>)
  n20 = control-ref of="R8"() -> (w29:refnum<vi>)
  n21 = control-ref of="R9"() -> (w28:refnum<vi>)
  n22 = control-ref of="R7"() -> (w27:refnum<vi>)
  n23 = control-ref of="R6"() -> (w26:refnum<vi>)
  n24 = control-ref of="R5"() -> (w25:refnum<vi>)
  n25 = control-ref of="R4"() -> (w24:refnum<vi>)
  n26 = control-ref of="R3"() -> (w23:refnum<vi>)
  n27 = control-ref of="R2"() -> (w22:refnum<vi>)
  n28 = control-ref of="R1"() -> (w21:refnum<vi>)
  n29 = control-ref of="R0"() -> (w20:refnum<vi>)
  n30 = control-ref of="T9"() -> (w19:refnum<vi>)
  n31 = control-ref of="T8"() -> (w18:refnum<vi>)
  n32 = control-ref of="T7"() -> (w17:refnum<vi>)
  n33 = control-ref of="T6"() -> (w16:refnum<vi>)
  n34 = control-ref of="T5"() -> (w15:refnum<vi>)
  n35 = control-ref of="T4"() -> (w14:refnum<vi>)
  n36 = control-ref of="T3"() -> (w13:refnum<vi>)
  n37 = control-ref of="T2"() -> (w12:refnum<vi>)
  n38 = control-ref of="T1"() -> (w11:refnum<vi>)
  n39 = control-ref of="T0"() -> (w10:refnum<vi>)
  n40 = flat-sequence {
    tunnel: w39 -> [w63]
    tunnel: [w63] -> w38
    frame #0 {
      # "Check if the QCS needs the registry patch and run the patching utility"
      n41 = disable-structure shown="Enabled" {
        frame Enabled {
          n42 = call "QCS - Check Registry.vi"() -> ("QCS needs reset?"=w64:bool)  [unwired: 5 in]
          n43 = case shown="False" w64 {
            frame False {
            }
            frame True {
              n44 = call "QCS - Locate Registry Patcher.vi"() -> ("dup path"=w66:path)  [unwired: 5 in]
              n45 = Path To String(path=w66) -> (string=w67:string)
              n46 = call <vilib>:"System Exec.vi"("wait until completion? (T)"=TRUE, "command line"=w67) -> ()  [unwired: 6 in, 4 out]
            }
          }
        }
        frame Disabled {
        }
      }
    }
  }
  n47 = flat-sequence {
    tunnel: [w69] -> w2
    tunnel: [w68] -> w1
    frame #0 {
      w68 = refnum<class "Inst.TC.lvclass"> refnum  # Inst.TC
      w69 = refnum<user-event> refnum  # MessageFromProcess
    }
  }
  n48 = Build Array (concatenate)(w29, w28, w27, w26, w25, w24, w23, w22, w21, w20, w19, w18, w17, w16, w15, w14, w13, w12, w11, w10, w9, w8, w4, w3) -> (w7:refnum<vi>[])
  n49 = Bundle("UpdateChannelInfo"=w52, "UpdateValuesAVS"=w51, "UpdateCalibrations"=w50, "UpdateLogFilePath"=w49, "TempStabilized"=w48, "Reset PID loop"=w47, "UpdateValuesZBridge"=w46, "CS Automode"=w45, "CallExtVI"=w44, "Data Array"=w41) -> (w43:T49)  [unwired: 1 in]
  n50 = register-events(w43, w7, w2) -> (reference out=w53:refnum<event-registration>)  [unwired: 2 in, 1 out]
  n51 = Bundle("Config folder"=w37, "Config File"=w35, "Calibrations Folder"=w34, "zBridge dll"=w33, "Variables Library"=w32, "Inst.TC"=w1) -> (w36:T50)  [unwired: 1 in]
  n52 = call <userlib>:"MGI Clear Error.vi"() -> ("Error Out"=w42:errorcluster)  [unwired: 7 in]
  n53 = while {
    tunnel: w53 -> [w77]
    shift-right: [w74] -> _
    shift-left: w42 -> [w75]
    tunnel: w43 -> [w73]
    tunnel: w38 -> [w72]
    shift-right: [w70] -> _
    shift-left: w36 -> [w71]
    stop <- FALSE stop-if-true
    # "Event handling loop"
    n54 = event shown="[3] <MessageFromProcess>: User Event" {
      selector: w77 -> [w80 w346 _ _ _ _ _ _ _ _ _ _ _ _ _ _ _ _ _ _ _ _ _ _ _ _ _ _ _ _ _ _ _ _ _ _ _ _ _ _ _ _ _ _ _ _ _ _ _ _ _ _ _ _ _ _ _ _ _ _ _ _ _ _ _ _ _ _ _ _ _ _ _ _ _ _ _ _ _ _ _ _ _ _ _ _ _ _ _ _ _]
      dyn-events: [w79 w345 _ _ _ _ _ _ _ _ _ _ _ _ _ _ _ _ _ _ _ _ _ _ _ _ _ _ _ _ _ _ _ _ _ _ _ _ _ _ _ _ _ _ _ _ _ _ _ _ _ _ _ _ _ _ _ _ _ _ _ _ _ _ _ _ _ _ _ _ _ _ _ _ _ _ _ _ _ _ _ _ _ _ _ _ _ _ _ _ _] -> _
      timeout: 200 -> [_ _ _ _ _ _ _ _ _ _ _ _ _ _ _ _ _ _ _ _ _ _ _ _ _ _ _ _ _ _ _ _ _ _ _ _ _ _ _ _ _ _ _ _ _ _ _ _ _ _ _ _ _ _ _ _ _ _ _ _ _ _ _ _ _ _ _ _ _ _ _ _ _ _ _ _ _ _ _ _ _ _ _ _ _ _ _ _ _ _ _]
      tunnel: w75 -> [w88 _ _ w525 w596 w645 w733 _ _ w945 _ _ _ w1075 w1084 _ _ _ _ _ _ _ _ _ w1333 _ w1342 _ _ _ _ _ _ _ _ w1447 _ _ _ _ _ _ _ _ _ _ _ _ _ _ _ _ _ _ _ _ _ _ w1873 w1893 _ _ _ _ _ w2038 _ _ _ _ _ _ _ _ _ _ _ _ _ _ _ _ _ _ _ _ _ _ _ _ _]
      tunnel: [w87 _ _ w527 w599 w644 w728 _ _ w943 _ _ _ w1074 w1084 _ _ _ _ _ _ _ _ _ w1333 _ w1342 _ _ _ _ _ _ w1429 _ w1447 _ _ _ _ _ _ _ _ _ _ _ _ _ _ _ _ _ _ _ _ _ _ w1872 w1892 _ _ _ _ _ w2038 _ _ _ _ _ _ _ _ _ _ _ _ _ _ _ _ _ _ _ _ _ _ _ _ _] -> w74
      tunnel: w73 -> [w85 _ _ _ w581 w640 w730 w835 w924 _ _ _ _ _ _ _ _ _ _ _ _ _ _ _ _ _ _ w1373 w1395 _ _ _ _ _ w1437 w1445 _ _ _ _ _ _ _ _ _ _ _ _ _ _ _ _ _ _ _ _ _ _ _ w1887 _ w1968 w1982 _ _ _ _ _ w2044 _ _ w2066 w2083 w2087 _ _ _ _ _ _ _ _ _ _ w2167 _ _ _ _ _ _]
      tunnel: w72 -> [_ w351 _ _ _ _ _ _ _ _ _ _ _ _ _ _ _ _ _ _ _ _ _ _ _ _ _ _ _ _ _ _ _ _ _ _ _ _ _ _ _ _ _ _ _ _ _ _ _ _ _ _ _ _ _ _ _ _ _ _ _ _ _ _ _ _ _ _ _ _ _ _ _ _ _ _ _ _ _ _ _ _ _ _ _ _ _ _ _ _ _]
      tunnel: w71 -> [w81 w342 w493 w530 w577 w638 w727 w831 w922 w942 w980 w1037 w1065 w1072 w1080 w1123 w1140 w1206 w1219 w1259 w1261 w1264 w1277 w1320 w1328 w1336 w1340 w1371 w1393 w1397 w1400 w1408 w1417 w1427 w1435 w1440 w1467 w1471 w1546 w1553 w1563 w1602 w1630 w1664 w1691 w1697 w1705 w1713 w1722 w1731 w1733 w1778 w1786 w1791 w1814 w1831 w1856 w1860 w1864 w1885 w1956 w1966 w1980 w1990 w2015 w2037 w2039 w2040 w2042 w2048 w2052 w2063 w2081 w2085 w2098 w2105 w2106 w2114 w2117 w2121 w2125 w2128 w2154 w2160 w2165 w2169 w2173 w2196 w2207 w2217 w2219]
      tunnel: [w82 w343 w493 w530 w577 w638 w727 w831 w922 w942 w980 w1037 w1065 w1071 w1080 w1123 w1140 w1206 w1219 w1259 w1261 w1264 w1277 w1320 w1328 w1336 w1340 w1371 w1393 w1397 w1400 w1408 w1417 w1427 w1435 w1440 w1467 w1471 w1546 w1553 w1563 w1602 w1630 w1664 w1691 w1697 w1705 w1713 w1722 w1731 w1733 w1778 w1786 w1791 w1814 w1831 w1856 w1860 w1864 w1885 w1956 w1966 w1980 w1990 w2015 w2037 w2039 w2040 w2042 w2048 w2052 w2063 w2081 w2085 w2098 w2105 w2106 w2114 w2117 w2121 w2125 w2128 w2154 w2160 w2165 w2169 w2173 w2196 w2207 w2217 w2219] -> w70
      event Timeout {
        n55 = event-data() -> ()  [unwired: 1 in, 3 out]
        n56 = call "First Call Resetable.vi"() -> ("First Call?"=w86:bool)
        n57 = Unbundle By Name(w85) -> ("UpdateChannelInfo"=w83:refnum<user-event>, "UpdateCalibrations"=w84:refnum<user-event>)
        n58 = case shown="True" w86 {
          tunnel: w88 -> [w93 w219]
          tunnel: [w93 w217] -> w87
          tunnel: w84 -> [_ w218]
          tunnel: w83 -> [w94 w216]
          tunnel: w81 -> [w92 w209]
          tunnel: [w92 w215] -> w82
          tunnel: w80 -> [w89 w208]
          tunnel: [w89 w208] -> w79
          frame False {
            n59 = Unbundle By Name(w92) -> ("Config folder"=w91:path, "zBridge dll"=w90:path)
            n60 = stacked-sequence {
              tunnel: w94 -> [w95 _ _]
              tunnel: w91 -> [_ w163 _]
              tunnel: w90 -> [_ w162 _]
              frame #0 {
                # "Update plots on timeout"
                # "Set enabled/disabled AVS channels"
                # "Reset stabilisation timer\nif the CS automode is off"
                n61 = property on="Miniplot Time" class="DigNum (strict)"() -> ("Value"=w156:dbl)  [unwired: 2 in, 2 out]
                n62 = call "Manage Data Arrays - uPlots.vi"("Data In"="Data Array", "Data Memory"=w156) -> ("Data Out"=w111:T28)  [unwired: 7 in]
                n63 = Index Array(array=w111) -> (element #1=w126:cluster{"R":dbl[], "T":dbl[], "Time":dbl[]}, element #2=w127:cluster{"R":dbl[], "T":dbl[], "Time":dbl[]}, element #3=w128:cluster{"R":dbl[], "T":dbl[], "Time":dbl[]}, element #4=w129:cluster{"R":dbl[], "T":dbl[], "Time":dbl[]}, element #5=w130:cluster{"R":dbl[], "T":dbl[], "Time":dbl[]}, element #6=w131:cluster{"R":dbl[], "T":dbl[], "Time":dbl[]}, element #7=w132:cluster{"R":dbl[], "T":dbl[], "Time":dbl[]}, element #8=w133:cluster{"R":dbl[], "T":dbl[], "Time":dbl[]}, element #9=w134:cluster{"R":dbl[], "T":dbl[], "Time":dbl[]}, element #10=w135:cluster{"R":dbl[], "T":dbl[], "Time":dbl[]})  [unwired: 10 in]
                n64 = Index Array(array="Data Array") -> (element #1=w155:cluster{"R":dbl[], "T":dbl[], "Time":dbl[]}, element #2=w154:cluster{"R":dbl[], "T":dbl[], "Time":dbl[]}, element #3=w153:cluster{"R":dbl[], "T":dbl[], "Time":dbl[]}, element #4=w152:cluster{"R":dbl[], "T":dbl[], "Time":dbl[]}, element #5=w151:cluster{"R":dbl[], "T":dbl[], "Time":dbl[]}, element #6=w150:cluster{"R":dbl[], "T":dbl[], "Time":dbl[]}, element #7=w149:cluster{"R":dbl[], "T":dbl[], "Time":dbl[]}, element #8=w148:cluster{"R":dbl[], "T":dbl[], "Time":dbl[]}, element #9=w147:cluster{"R":dbl[], "T":dbl[], "Time":dbl[]}, element #10=w146:cluster{"R":dbl[], "T":dbl[], "Time":dbl[]})  [unwired: 10 in]
                n65 = property on="Plot type" class="Enum (strict)"() -> ("Value"=w114:enum16{"R vs Time", "T vs Time"})  [unwired: 2 in, 2 out]
                n66 = call "Select Data Array.vi"("Value"=w114, "Cluster 2"=w126) -> ("Cluster"=w136:cluster{"Time":dbl[], "T":dbl[]})  [unwired: 7 in]
                n67 = call "Select Data Array.vi"("Value"=w114, "Cluster 2"=w127) -> ("Cluster"=w137:cluster{"Time":dbl[], "T":dbl[]})  [unwired: 7 in]
                n68 = call "Select Data Array.vi"("Value"=w114, "Cluster 2"=w128) -> ("Cluster"=w138:cluster{"Time":dbl[], "T":dbl[]})  [unwired: 7 in]
                n69 = call "Select Data Array.vi"("Value"=w114, "Cluster 2"=w129) -> ("Cluster"=w139:cluster{"Time":dbl[], "T":dbl[]})  [unwired: 7 in]
                n70 = call "Select Data Array.vi"("Value"=w114, "Cluster 2"=w130) -> ("Cluster"=w145:cluster{"Time":dbl[], "T":dbl[]})  [unwired: 7 in]
                n71 = call "Select Data Array.vi"("Value"=w114, "Cluster 2"=w131) -> ("Cluster"=w140:cluster{"Time":dbl[], "T":dbl[]})  [unwired: 7 in]
                n72 = call "Select Data Array.vi"("Value"=w114, "Cluster 2"=w132) -> ("Cluster"=w141:cluster{"Time":dbl[], "T":dbl[]})  [unwired: 7 in]
                n73 = call "Select Data Array.vi"("Value"=w114, "Cluster 2"=w133) -> ("Cluster"=w142:cluster{"Time":dbl[], "T":dbl[]})  [unwired: 7 in]
                n74 = call "Select Data Array.vi"("Value"=w114, "Cluster 2"=w134) -> ("Cluster"=w143:cluster{"Time":dbl[], "T":dbl[]})  [unwired: 7 in]
                n75 = call "Select Data Array.vi"("Value"=w114, "Cluster 2"=w135) -> ("Cluster"=w144:cluster{"Time":dbl[], "T":dbl[]})  [unwired: 7 in]
                n76 = call "Select Data Array.vi"("Value"=w114, "Cluster 2"=w155) -> ("Cluster"=→"R-Plot 0":cluster{"Time":dbl[], "T":dbl[]})  [unwired: 7 in]
                n77 = call "Select Data Array.vi"("Value"=w114, "Cluster 2"=w154) -> ("Cluster"=→"R-Plot 1":cluster{"Time":dbl[], "T":dbl[]})  [unwired: 7 in]
                n78 = call "Select Data Array.vi"("Value"=w114, "Cluster 2"=w153) -> ("Cluster"=→"R-Plot 2":cluster{"Time":dbl[], "T":dbl[]})  [unwired: 7 in]
                n79 = call "Select Data Array.vi"("Value"=w114, "Cluster 2"=w152) -> ("Cluster"=→"R-Plot 3":cluster{"Time":dbl[], "T":dbl[]})  [unwired: 7 in]
                n80 = call "Select Data Array.vi"("Value"=w114, "Cluster 2"=w151) -> ("Cluster"=→"R-Plot 4":cluster{"Time":dbl[], "T":dbl[]})  [unwired: 7 in]
                n81 = call "Select Data Array.vi"("Value"=w114, "Cluster 2"=w150) -> ("Cluster"=→"R-Plot 5":cluster{"Time":dbl[], "T":dbl[]})  [unwired: 7 in]
                n82 = call "Select Data Array.vi"("Value"=w114, "Cluster 2"=w149) -> ("Cluster"=→"R-Plot 6":cluster{"Time":dbl[], "T":dbl[]})  [unwired: 7 in]
                n83 = call "Select Data Array.vi"("Value"=w114, "Cluster 2"=w148) -> ("Cluster"=→"R-Plot 7":cluster{"Time":dbl[], "T":dbl[]})  [unwired: 7 in]
                n84 = call "Select Data Array.vi"("Value"=w114, "Cluster 2"=w147) -> ("Cluster"=→"R-Plot 8":cluster{"Time":dbl[], "T":dbl[]})  [unwired: 7 in]
                n85 = call "Select Data Array.vi"("Value"=w114, "Cluster 2"=w146) -> ("Cluster"=→"R-Plot 9":cluster{"Time":dbl[], "T":dbl[]})  [unwired: 7 in]
                n86 = Bundle("Cluster"=w136, "Cluster"=w137, "Cluster"=w138, "Cluster"=w139, "Cluster"=w145, "Cluster"=w140, "Cluster"=w141, "Cluster"=w142, "Cluster"=w143, "Cluster"=w144) -> (→"uPlots":T59)  [unwired: 1 in]
                n87 = local read "_ExtVIReference"() -> (w110:refnum<vi>)
                n88 = property on="CS Mode" class="Enum (strict)"() -> ("Value"=w159:T39)  [unwired: 2 in, 2 out]
                n89 = call "GetExtVIStatus.vi"("vi reference in"=w110) -> ("Exec.State"=→"CS.Mode1.VI State":T46)  [unwired: 2 out]
                n90 = Not(x="CS.Mode1.Auto Advance") -> (.not. x?=w158:bool)
                n91 = Equal To 0?(x=w159) -> (x = 0?=w108:bool)
                n92 = Generate User Event(user event=w95, event data cluster=bool[] [] ("event data")) -> ()  [unwired: 2 in, 2 out]
                n93 = Or(x=w108, y=w158) -> (x .or. y?=w157:bool)
                n94 = case shown="True" w157 {
                  frame False {
                  }
                  frame True {
                    n95 = call "Current Time(double).vi"() -> ("Current Time (double)"=w161:dbl)  [unwired: 6 in, 1 out]
                    n96 = local write "_TimeOld"(w161) -> ()
                  }
                }
                n97 = control-ref of="uA 2"() -> (w96:refnum<vi>)
                n98 = control-ref of="uA 3"() -> (w97:refnum<vi>)
                n99 = control-ref of="uA 0"() -> (w107:refnum<vi>)
                n100 = control-ref of="uA 1"() -> (w103:refnum<vi>)
                n101 = property class="DigNum (strict)"(reference=w107) -> (reference out=w106:refnum<vi>, "Key Focus"=w105:bool)  [unwired: 1 in, 1 out]
                n102 = property class="DigNum (strict)"(reference=w103) -> (reference out=w104:refnum<vi>, "Key Focus"=w102:bool)  [unwired: 1 in, 1 out]
                n103 = property class="DigNum (strict)"(reference=w96) -> (reference out=w98:refnum<vi>, "Key Focus"=w99:bool)  [unwired: 1 in, 1 out]
                n104 = property class="DigNum (strict)"(reference=w97) -> (reference out=w100:refnum<vi>, "Key Focus"=w101:bool)  [unwired: 1 in, 1 out]
                n105 = property class="DigNum (strict)"(reference=w106, "Visible"=w105) -> ()  [unwired: 1 in, 2 out]
                n106 = property class="DigNum (strict)"(reference=w104, "Visible"=w102) -> ()  [unwired: 1 in, 2 out]
                n107 = property class="DigNum (strict)"(reference=w98, "Visible"=w99) -> ()  [unwired: 1 in, 2 out]
                n108 = property class="DigNum (strict)"(reference=w100, "Visible"=w101) -> ()  [unwired: 1 in, 2 out]
              }
              frame #1 {
                n109 = property on="Bridge status" class="Clust (strict)"() -> ("Value"=w165:errorcluster)  [unwired: 2 in, 2 out]
                n110 = case shown="Error" w165 {
                  tunnel: w163 -> [_ w169]
                  tunnel: w162 -> [_ w168]
                  frame No Error {
                  }
                  frame Error {
                    n111 = call "StopScan.vi"("error in (no error)"=errorcluster {"status"=FALSE, "code"=0, "source"=""}, "path in"=w168) -> ("path out"=w175:path)  [unwired: 8 in, 1 out]
                    n112 = call "SetParFilePath.vi"("path"=w169, "zDll"=w175) -> ("error out"=w177:errorcluster, "zDll out"=w176:path)  [unwired: 8 in]
                    n113 = call "StartScan.vi"("error in (no error)"=w177, "path in"=w176) -> ("error out"=w173:errorcluster)  [unwired: 8 in, 1 out]
                    n114 = property on="Bridge status" class="Clust (strict)"("Value"=w173) -> ()  [unwired: 2 in, 2 out]
                    n115 = Unbundle By Name(w173) -> ("status"=w171:bool)
                    n116 = Not(x=w171) -> (.not. x?=w172:bool)
                    n117 = call "IsDisabled.vi"("Enabled?"=w172) -> ("Numeric"=w170:i16)
                    n118 = property on="Main Panel" class="TabCtl (strict)"("Disabled"=w170) -> ()  [unwired: 2 in, 2 out]
                    n119 = property on="Lower Panel" class="TabCtl (strict)"("Disabled"=w170) -> ()  [unwired: 2 in, 2 out]
                  }
                }
                n120 = property on="CS status" class="Clust (strict)"() -> ("Value"=w164:errorcluster)  [unwired: 2 in, 2 out]
                n121 = case shown="Error" w164 {
                  frame No Error {
                    n122 = property on="CS Indicators Panel" class="TabCtl (strict)"("Disabled"=u8 0) -> ()  [unwired: 2 in, 2 out]
                  }
                  frame Error {
                    n123 = property on="CS Indicators Panel" class="TabCtl (strict)"("Disabled"=u8 2) -> ()  [unwired: 2 in, 2 out]
                  }
                }
              }
              frame #2 {
                # "Check if the structure is \nnot empty and only one\nof Scalar or Array is set"
                # "Set FP control value from external script/program"
                n124 = local read "_SetControl"() -> (w178:T1)
                n125 = Unbundle By Name(w178) -> ("Name"=w180:string, "Scalar"=w179:string, "Array"=w188:string[][])
                n126 = call <userlib>:"Empty 2D Array (String)__ogtk.vi"("Array"=w188) -> ("Empty Array?"=w185:bool)  [unwired: 8 in]
                n127 = Empty String/Path?(string/path=w180) -> (empty?=w184:bool)
                n128 = Empty String/Path?(string/path=w179) -> (empty?=w183:bool)
                n129 = Not(x=w184) -> (.not. x?=w182:bool)
                n130 = Not(x=w183) -> (.not. x?=w186:bool)
                n131 = Not(x=w185) -> (.not. x?=w189:bool)
                n132 = Exclusive Or(1:w189, 2:w186) -> (0:w187:bool)
                n133 = And(x=w182, y=w187) -> (x .and. y?=w181:bool)
                n134 = case shown="True" w181 {
                  tunnel: w180 -> [_ w193]
                  tunnel: w179 -> [_ w192]
                  tunnel: w188 -> [_ w191]
                  tunnel: w189 -> [_ w190]
                  frame False {
                  }
                  frame True {
                    n135 = flat-sequence {
                      tunnel: w193 -> [w197]
                      tunnel: w192 -> [w196]
                      tunnel: w191 -> [w194]
                      tunnel: w190 -> [w195]
                      frame #0 {
                        n136 = local read "VIRef"() -> (w198:T2)
                        n137 = case shown="True" w195 {
                          tunnel: w198 -> [w201 w204]
                          tunnel: w197 -> [w200 w203]
                          tunnel: w196 -> [w199 _]
                          tunnel: w194 -> [_ w202]
                          frame False {
                            n138 = call "Push2VI.vi"("New Value"=w199, "element"=w200, "VIRef"=w201) -> ()  [unwired: 8 in, 1 out]
                          }
                          frame True {
                            n139 = call "PushArray2VI.vi"("Str"=w202, "element"=w203, "VIRef"=w204) -> ()  [unwired: 8 in, 1 out]
                          }
                        }
                      }
                      frame #1 {
                        w206 = ""
                        n140 = Bundle(w206, w206, "Array"=string[][] []) -> (→"_SetControl":cluster{string, string, "Array":string[][]})  [unwired: 1 in]
                      }
                    }
                  }
                }
              }
            }
          }
          frame True {
            # "First call  - do startup initialization"
            n141 = stacked-sequence {
              tunnel: w219 -> [_ _ w264 _]
              tunnel: [_ _ w258 _] -> w217
              tunnel: w218 -> [_ _ w260 _]
              tunnel: w216 -> [_ _ _ w319]
              tunnel: [_ _ w256 _] -> w214
              tunnel: [_ _ w257 _] -> w213
              tunnel: [_ _ w255 _] -> w212
              tunnel: [_ _ w253 _] -> w211
              tunnel: [w220 _ _ _] -> w210
              frame #0 {
                # "Set control bindings"
                # "\\\\localhost\\DR TempControl\\Currents(In)"
                # "\\\\localhost\\DR TempControl\\Temperatures"
                # "\\\\localhost\\DR TempControl\\Resistances"
                # "\\\\localhost\\DR TempControl\\Currents(Out)"
                n142 = disable-structure shown="RUN_TIME_ENGINE==True" {
                  disable-tunnel: [w233 "\\\\localhost\\DR TempControl\\"] -> w221
                  disable-tunnel: [w230 w243] -> w220
                  frame condition #0 {
                    w240 = u16 0 items=["overwrite", "ask first", "don't overwrite"] ("overwrite")
                    # "Deploy the shared variable library. If there are few copies of the program\nrunning - generate unique name for every copy."
                    n143 = call "Enum Variables.vi"("regular expression"="DR TempControl.*") -> ("Containers"=w238:string[])  [unwired: 15 in, 3 out]
                    n144 = call "Generate New Name.vi"("Existing names"=w238, "Base Name"="DR TempControl") -> ("New Name (path)"=w235:path, "New Name"=w234:string)  [unwired: 16 in]
                    n145 = call <userlib>:"Temporary Directory__ogtk.vi"("Relative path (.)"=w235) -> ("Temporary Directory (+ Relative)"=w239:path)
                    n146 = call <userlib>:"Current VIs Parent Directory__ogtk.vi"("Relative path (.)"=path "DR TempControl.lvlib" ("Library Path")) -> ("Parent Directory (+ Relative)"=w241:path)  [unwired: 4 in]
                    n147 = call <vilib>:"Librarian Copy.vi"("source"=w241, "overwrite"=w240, "destination"=w239) -> ("dup destination"=w230:path)  [unwired: 7 in, 1 out]
                    n148 = invoke class="App" method="Library.Deploy Library"("libPath"=w230) -> ()  [unwired: 4 in, 5 out]
                    n149 = Concatenate Strings("\\\\localhost\\" ("string"), w234, "\\" ("string")) -> (w233:string)
                  }
                  frame condition #1 (active) {
                    # "Default library is deployed automatically in development environment"
                    n150 = call <userlib>:"Current VIs Parent Directory__ogtk.vi"("Relative path (.)"=path "DR TempControl.lvlib" ("Library Path")) -> ("Parent Directory (+ Relative)"=w243:path)  [unwired: 4 in]
                  }
                }
                n151 = Concatenate Strings(w221, "Resistances" ("string")) -> (w227:string)
                n152 = Concatenate Strings(w221, "Temperatures" ("string")) -> (w224:string)
                n153 = Concatenate Strings(w221, "Currents(Out)" ("string")) -> (w223:string)
                n154 = Concatenate Strings(w221, "Currents(In)" ("string")) -> (w222:string)
                n155 = property on="R Array" class="Arr (strict)"("FPB.URL"=w227) -> ()  [unwired: 2 in, 2 out]
                n156 = property on="T Array" class="Arr (strict)"("FPB.URL"=w224) -> ()  [unwired: 2 in, 2 out]
                n157 = property on="CS.Actual Current" class="Arr (strict)"("FPB.URL"=w223) -> ()  [unwired: 2 in, 2 out]
                n158 = property on="CS.Automode Current" class="Arr (strict)"("FPB.URL"=w222) -> ()  [unwired: 2 in, 2 out]
              }
              frame #1 {
                w251 = u8 0 ("Disabled")
                n159 = call <userlib>:"Current VIs Reference__ogtk.vi"() -> ("Current VI's reference"=w249:refnum<vi>)  [unwired: 5 in]
                n160 = property on="Minimize UI 1" class="Bool (strict)"("Val(Sgnl)"=FALSE ("Value (Signaling)")) -> ()  [unwired: 2 in, 2 out]
                n161 = call "GetFrontPanelControls.vi"("Ref to VI"=w249) -> ("VIRef"=w248:T2)  [unwired: 9 in, 1 out]
                "VIRef" <- w248
                n162 = Unbundle By Name(w248) -> ("Full Name"=→"ControlNames":string[])
                n163 = property on="_String" class="Str"("Visible"=FALSE) -> ()  [unwired: 2 in, 2 out]
                n164 = property on="Lower Panel" class="TabCtl (strict)"("Disabled"=w251) -> ()  [unwired: 2 in, 2 out]
                n165 = property on="Main Panel" class="TabCtl (strict)"("Disabled"=w251) -> ()  [unwired: 2 in, 2 out]
                n166 = property on="CS Indicators Panel" class="TabCtl (strict)"("Disabled"=w251) -> ()  [unwired: 2 in, 2 out]
                n167 = property on="Side Panel" class="TabCtl (strict)"("Disabled"=w251) -> ()  [unwired: 2 in, 2 out]
                n168 = property on="Top Toolbar" class="TabCtl (strict)"("Disabled"=w251) -> ()  [unwired: 2 in, 2 out]
              }
              frame #2 {
                # "Read settings from the config file"
                n169 = flat-sequence {
                  tunnel: w264 -> [w265]
                  tunnel: [w265] -> w259
                  tunnel: [w268] -> w257
                  tunnel: [w269] -> w256
                  tunnel: [w270] -> w255
                  tunnel: [w269] -> w254
                  tunnel: [w266] -> w253
                  tunnel: [w285] -> w263
                  tunnel: w259 -> [w284]
                  tunnel: w254 -> [w286]
                  tunnel: w263 -> [w296]
                  tunnel: [w296] -> w262
                  tunnel: [w300] -> w261
                  tunnel: w262 -> [w297]
                  tunnel: w261 -> [w305]
                  tunnel: [w305] -> w252
                  tunnel: [w309] -> w258
                  tunnel: w260 -> [w306]
                  tunnel: w252 -> [w307]
                  frame #0 {
                    w271 = path "C:/LC Data" ("LC Data")
                    n170 = call "Generate config file path.vi"("LC data path"=w271) -> ("Config folder"=w270:path)  [unwired: 18 in]
                    n171 = call <userlib>:"Build Path - Traditional__ogtk.vi"("name or relative path"="config.ini", "base path"=w270) -> ("appended path"=w269:path)
                    n172 = call <userlib>:"Build Path - Traditional__ogtk.vi"("name or relative path"="Calibrations", "base path"=w271) -> ("appended path"=w268:path)
                    n173 = property on="Calibrations Folder" class="Path"("Value"=w268) -> ()  [unwired: 2 in, 2 out]
                    n174 = call <userlib>:"Current VIs Parent Directory__ogtk.vi"("Relative path (.)"=path "data/ImpBridgeDll.dll" ("Library Path")) -> ("Parent Directory (+ Relative)"=w266:path)  [unwired: 4 in]
                    "_zBridgeDll" <- w266
                  }
                  frame #1 {
                    n175 = control-ref of="zBridge.Active Channels"() -> (w283:refnum<vi>)
                    n176 = control-ref of="CS Settings"() -> (w282:refnum<vi>)
                    n177 = control-ref of="Bridge settings"() -> (w281:refnum<vi>)
                    n178 = control-ref of="Runtime Settings"() -> (w280:refnum<vi>)
                    n179 = control-ref of="Data Logging Settings"() -> (w279:refnum<vi>)
                    n180 = control-ref of="PID setup"() -> (w278:refnum<vi>)
                    n181 = control-ref of="CS Cannel Names"() -> (w292:refnum<vi>)
                    n182 = control-ref of="AVS names"() -> (w274:refnum<vi>)
                    n183 = control-ref of="_CurCalibrations"() -> (w275:refnum<vi>)
                    n184 = control-ref of="CS.Mode1.PID"() -> (w276:refnum<vi>)
                    n185 = control-ref of="CS.Mode1.Settings"() -> (w277:refnum<vi>)
                    n186 = call <userlib>:"Current VIs Parent Directory__ogtk.vi"("Relative path (.)"=path "data/config.ini") -> ("Parent Directory (+ Relative)"=w289:path)  [unwired: 4 in]
                    n187 = Build Array(w283, w282, w281, w280, w279, w278, w292, w274, w275, w276, w277) -> (w288:refnum<vi>[])
                    n188 = call "Save Load Settings to File by Ref with path.vi"("Array of Cluster References"=w288, "Action"=enum8{"Load", "Save"}."Load", "error in (no error)"=w284, "Configuration file"=w289) -> ("error out"=w291:errorcluster)  [unwired: 5 in]
                    n189 = call <userlib>:"MGI Clear Error.vi"("Error In"=w291) -> ("Error Out"=w290:errorcluster)  [unwired: 6 in]
                    n190 = call "Save Load Settings to File by Ref with path.vi"("Array of Cluster References"=w288, "Action"=enum8{"Load", "Save"}."Load", "error in (no error)"=w290, "Configuration file"=w286) -> ("error out"=w285:errorcluster)  [unwired: 5 in]
                  }
                  frame #2 {
                    n191 = Wait (ms)(milliseconds to wait=250) -> ()  [unwired: 1 out]
                  }
                  frame #3 {
                    n192 = control-ref of="Sensor Calibrations"() -> (w299:refnum<vi>)
                    n193 = control-ref of="_CurCalibrations"() -> (w298:refnum<vi>)
                    n194 = control-ref of="Calibrations Folder"() -> (w302:refnum<vi>)
                    n195 = control-ref of="_QuickConvertCal"() -> (w301:refnum<vi>)
                    n196 = control-ref of="Sensor 1"() -> (w303:refnum<vi>)
                    n197 = call "ReloadCalibrations.vi"("error in (no error)"=w297, "Quick convert sensors"=w301, "CurCalibrations"=w298, "Calibration files path"=w302, "Channel1 sensors"=w303, "Channels list"=w299) -> ("error out"=w300:errorcluster)  [unwired: 1 out]
                  }
                  frame #4 {
                    n198 = Wait (ms)(milliseconds to wait=250) -> ()  [unwired: 1 out]
                  }
                  frame #5 {
                    n199 = Generate User Event(user event=w306, event data cluster="" ("event data"), error in=w307) -> (error out=w309:errorcluster)  [unwired: 1 in, 1 out]
                  }
                }
              }
              frame #3 {
                w311 = FALSE ("Mode1 ON")
                w328 = u8 0 ("Disabled")
                # "Set enabled/disabled AVS channels"
                # "Reset pid parameters"
                # "Print VI version in the low left corner"
                # "Reset Current lists\nto first element"
                # "Hardware settings"
                # "Reset currents lists"
                # "Set initial controls state"
                n200 = call "Currents-Temp list - check ranges.vi"() -> ("I_list out"=w322:dbl[][])  [unwired: 5 in]
                n201 = property on="Start" class="Bool (strict)"("Visible"=TRUE, "Disabled"=u8 0, "Value"=FALSE ("start")) -> ()  [unwired: 2 in, 2 out]
                n202 = property on="CS.Mode1.List:Index" class="DigNum (strict)"("Val(Sgnl)"=1 ("Value (Signaling)")) -> ()  [unwired: 2 in, 2 out]
                n203 = property on="CS Mode" class="Enum (strict)"("Val(Sgnl)"=CS_mode."Manual" ("CS Mode")) -> ()  [unwired: 2 in, 2 out]
                n204 = local write "CS.Mode2.List"(w322) -> ()
                n205 = property on="CS.Mode1.List:To First" class="Bool (strict)"("Val(Sgnl)"=TRUE ("Value (Signaling)")) -> ()  [unwired: 2 in, 2 out]
                n206 = property on="CS.Mode1.Start" class="Bool (strict)"("Value"=w311) -> ()  [unwired: 2 in, 2 out]
                n207 = property on="CS.Mode2.Start" class="Bool (strict)"("Value"=w311) -> ()  [unwired: 2 in, 2 out]
                n208 = property on="CS.QCS I0 Output" class="Enum (strict)"("Disabled"=u8 2, "Val(Sgnl)"=T38."Channel 0" ("Map Channel 0 to")) -> ()  [unwired: 2 in, 2 out]
                n209 = property on="Bridge Type" class="Enum (strict)"("Disabled"=w328) -> ()  [unwired: 2 in, 2 out]
                n210 = property on="AVS GPIB Address" class="VISAName"("Disabled"=w328) -> ()  [unwired: 2 in, 2 out]
                n211 = property on="TCS RS232 Port" class="VISAName"("Disabled"=w328) -> ()  [unwired: 2 in, 2 out]
                n212 = property on="CS type" class="Enum (strict)"("Disabled"=w328) -> ()  [unwired: 2 in, 2 out]
                n213 = property on="CS.QCS Device Nr" class="DigNum (strict)"("Disabled"=w328) -> ()  [unwired: 2 in, 2 out]
                n214 = property on="Side Panel" class="TabCtl (strict)"("Value"=T34."Devices Settings" ("Tab Control 2")) -> ("Pages"=w316:refnum<vi>[])  [unwired: 2 in, 2 out]
                n215 = Index Array(array=w316, index=1) -> (element=w313:refnum<vi>)
                n216 = property class="App"() -> ("App.Kind"=w325:T60)  [unwired: 2 in, 2 out]
                n217 = property class="Page"(reference=w313, "PageEnb"=T51."Page Disabled & Grayed" ("Page Enabled State")) -> ()  [unwired: 1 in, 2 out]
                n218 = case shown="\"invalid app kind\", Default" w325 {
                  tunnel: [w333 w341] -> w310
                  frame "invalid app kind", Default {
                    n219 = control-ref of="This VI"() -> (w340:refnum<vi>)
                    n220 = property class="VI"(reference=w340) -> ("Hist.Revision"=w339:u32)  [unwired: 1 in, 2 out]
                    n221 = Divide(x=w339, y=1000.0 ("x")) -> (x/y=w335:dbl)
                    n222 = Number To Fractional String(use system decimal point (T)=FALSE, number=w335, precision (6)=i16 2) -> (F-format string=w334:string)  [unwired: 1 in]
                    n223 = Concatenate Strings("" ("string"), w334) -> (w333:string)
                  }
                  frame "Run Time System" {
                    n224 = call <userlib>:"MGI Get Executable Version.vi"() -> ("Version"=w341:string)  [unwired: 7 in]
                  }
                }
                "VI Version" <- w310
                n225 = property on="Channels Panel" class="TabCtl (strict)"("Val(Sgnl)"=T8."All" ("Value (Signaling)")) -> ()  [unwired: 2 in, 2 out]
                n226 = local write "CS.Mode1.PID Error"(0.0 ("T_error")) -> ()
                n227 = Generate User Event(user event=w319, event data cluster=bool[] [] ("event data")) -> ()  [unwired: 2 in, 2 out]
              }
            }
            n228 = Bundle By Name(cluster=w209, "Config folder"=w212, "Config File"=w214, "Calibrations Folder"=w213, "zBridge dll"=w211, "Variables Library"=w210) -> (w215:T50)
          }
        }
      }
      event "Start": Value Change {
        # "\"Start\" button clicked -> start measuring"
        n229 = event-data() -> ()  [unwired: 1 in, 6 out]
        n230 = Unbundle By Name(w342) -> ("Config File"=w348:path, "zBridge dll"=w349:path, "Config folder"=w350:path, "Inst.TC"=w347:refnum<class "Inst.TC.lvclass">)
        n231 = stacked-sequence {
          tunnel: w351 -> [_ _ _ _ _ _ _ w484]
          tunnel: w350 -> [_ _ _ _ w420 _ _ _]
          tunnel: w349 -> [_ _ _ _ w419 _ _ _]
          tunnel: w348 -> [_ w361 _ _ _ _ _ _]
          tunnel: w347 -> [_ _ _ _ _ _ w480 _]
          tunnel: w346 -> [_ _ _ _ _ _ w482 _]
          tunnel: [_ _ _ _ _ _ w481 _] -> w345
          tunnel: [_ _ _ _ _ _ w478 _] -> w344
          frame #0 {
            n232 = property on="Run Description" class="Str"() -> ("Value"=w354:string)  [unwired: 2 in, 2 out]
            n233 = property on="Query Description" class="Bool (strict)"() -> ("Value"=w353:bool)  [unwired: 2 in, 2 out]
            n234 = Not(x=w353) -> (.not. x?=w352:bool)
            n235 = call "Run Reference DLG.vi"("Enable"=w353, "Run Reference"=w354, "Dont' ask again"=w352) -> ("Dont' ask again"=w356:bool, "Run Reference"=w357:string, "OK"=w358:bool)  [unwired: 13 in, 1 out]
            n236 = Not(x=w356) -> (.not. x?=w355:bool)
            n237 = case shown="True" w358 {
              tunnel: w357 -> [_ w360]
              tunnel: w355 -> [_ w359]
              frame False {
              }
              frame True {
                n238 = property on="Run Description" class="Str"("Val(Sgnl)"=w360) -> ()  [unwired: 2 in, 2 out]
                n239 = property on="Query Description" class="Bool (strict)"("Val(Sgnl)"=w359) -> ()  [unwired: 2 in, 2 out]
              }
            }
          }
          frame #1 {
            # "Save new settings to config file"
            n240 = control-ref of="zBridge.Active Channels"() -> (w365:refnum<vi>)
            n241 = control-ref of="CS.Mode1.PID"() -> (w364:refnum<vi>)
            n242 = control-ref of="CS.Mode1.Settings"() -> (w363:refnum<vi>)
            n243 = control-ref of="CS.Mode1.Settings"() -> (w362:refnum<vi>)
            n244 = control-ref of="CS Cannel Names"() -> (w368:refnum<vi>)
            n245 = control-ref of="AVS names"() -> (w367:refnum<vi>)
            n246 = control-ref of="_CurCalibrations"() -> (w366:refnum<vi>)
            n247 = control-ref of="Bridge settings"() -> (w373:refnum<vi>)
            n248 = control-ref of="Runtime Settings"() -> (w374:refnum<vi>)
            n249 = control-ref of="CS Settings"() -> (w372:refnum<vi>)
            n250 = control-ref of="Sensor Calibrations"() -> (w375:refnum<vi>)
            n251 = control-ref of="PID setup"() -> (w376:refnum<vi>)
            n252 = control-ref of="Data Logging Settings"() -> (w371:refnum<vi>)
            n253 = Build Array(w365, w373, w374, w372, w371, w375, w376, w368, w367, w366, w364, w363, w362) -> (w369:refnum<vi>[])
            n254 = call "Save Load Settings to File by Ref with path.vi"("Array of Cluster References"=w369, "Action"=enum8{"Load", "Save"}."Save", "Configuration file"=w361) -> ()  [unwired: 6 in, 1 out]
          }
          frame #2 {
            w392 = u8 2 ("Disabled")
            # "Reset stop button"
            # "Hide Disable Start button"
            # "Load external calibration VI"
            # "Set controls\nInitialize data for run"
            # "Lock hardware settings"
            n255 = property on="Bridge Type" class="Enum (strict)"("Disabled"=w392) -> ()  [unwired: 2 in, 2 out]
            n256 = property on="AVS GPIB Address" class="VISAName"("Disabled"=w392) -> ()  [unwired: 2 in, 2 out]
            n257 = property on="AVS RS232 Port" class="VISAName"("Disabled"=w392) -> ()  [unwired: 2 in, 2 out]
            n258 = property on="TCS RS232 Port" class="VISAName"("Disabled"=w392) -> ()  [unwired: 2 in, 2 out]
            n259 = property on="CS type" class="Enum (strict)"("Disabled"=w392) -> ()  [unwired: 2 in, 2 out]
            n260 = property on="CS.QCS Device Nr" class="DigNum (strict)"("Disabled"=w392) -> ()  [unwired: 2 in, 2 out]
            n261 = property on="CS.QCS I0 Output" class="Enum (strict)"("Disabled"=u8 0) -> ()  [unwired: 2 in, 2 out]
            n262 = call "Current Time(double).vi"() -> ("Current Time (double)"=w381:dbl)  [unwired: 6 in, 1 out]
            n263 = local write "_TimeOld"(w381) -> ()
            n264 = property on="External VI Path" class="Path"() -> ("Value"=w391:path)  [unwired: 2 in, 2 out]
            n265 = vi-ref "OnTempStabilizedRef.vi"() -> (w390:refnum<vi>)
            n266 = local write "VI called?"(FALSE ("VI called?")) -> ()
            n267 = Open VI Reference(type specifier VI Refnum (for type only)=w390, vi path=w391) -> (vi reference=→"_ExtVIReference":refnum<vi>)  [unwired: 4 in, 1 out]
            n268 = property on="Start" class="Bool (strict)"("Visible"=TRUE, "Disabled"=u8 2) -> ()  [unwired: 2 in, 2 out]
            n269 = Initialize Array(cluster{"R":dbl[], "T":dbl[], "Time":dbl[]} {"R"=[], "T"=[], "Time"=[]}, 10 ("dimension size")) -> (w385:cluster{"R":dbl[], "T":dbl[], "Time":dbl[]}[])
            n270 = local write "Data Array"(w385) -> ()
            n271 = disable-structure shown="Enabled" {
              frame Enabled {
                n272 = property on="Stop" class="Bool (strict)"("Value"=FALSE ("MainStopButton")) -> ()  [unwired: 2 in, 2 out]
              }
              frame Disabled {
              }
            }
            n273 = property on="Side Panel" class="TabCtl (strict)"() -> ("Pages"=w380:refnum<vi>[])  [unwired: 2 in, 2 out]
            n274 = Index Array(array=w380, index=1) -> (element=w378:refnum<vi>)
            n275 = property class="Page"(reference=w378, "PageEnb"=T51."Page Enabled" ("Page Enabled State")) -> ()  [unwired: 1 in, 2 out]
          }
          frame #3 {
            # "Initialize CS"
            n276 = local read "_CSClassRef"() -> (w404:refnum<class "CS.lvclass">)
            n277 = call-dynamic "Initialize.vi"("CS in"=w404, "HW Address"="_CS_Address", "error in (no error)"=T52 {"error"=FALSE, "code"=0, "source"=""} ("error in")) -> ("CS out"=w397:refnum<class "CS.lvclass">, "Instrument ID"=→"CS.ID":string, "error out"=w396:errorcluster)  [unwired: 10 in]
            n278 = call-dynamic "Get Currents & Ranges.vi"("CS.lvclass in"=w397, "error in (no error)"=w396) -> ("CS.lvclass out"=w405:refnum<class "CS.lvclass">, "I0"=w406:cluster{"Value":dbl, "Range":dbl}, "I1"=w398:cluster{"Value":dbl, "Range":dbl}, "I2"=w399:cluster{"Value":dbl, "Range":dbl}, "I3"=w400:cluster{"Value":dbl, "Range":dbl}, "error out"=w402:errorcluster)  [unwired: 12 in]
            "CS status" <- w402
            n279 = local write "_CSClassRef"(w405) -> ()
            n280 = Unbundle By Name(w402) -> ("status"=w394:bool)
            n281 = case shown="True" w394 {
              tunnel: w398 -> [w418 _]
              tunnel: w399 -> [w417 _]
              tunnel: w400 -> [w416 _]
              tunnel: w406 -> [w410 _]
              frame False {
                n282 = Unbundle By Name(w410) -> ("Value"=w409:dbl, "Range"=w408:dbl)
                n283 = Unbundle By Name(w418) -> ("Value"=w415:dbl, "Range"=w414:dbl)
                n284 = Unbundle By Name(w417) -> ("Value"=w413:dbl, "Range"=w412:dbl)
                n285 = Unbundle By Name(w416) -> ("Value"=w407:dbl, "Range"=w411:dbl)
                n286 = property on="I" class="DigNum (strict)"("Value"=w409) -> ()  [unwired: 2 in, 2 out]
                n287 = property on="I" class="DigNum (strict)"("Value"=w415) -> ()  [unwired: 2 in, 2 out]
                n288 = property on="I" class="DigNum (strict)"("Value"=w413) -> ()  [unwired: 2 in, 2 out]
                n289 = property on="I" class="DigNum (strict)"("Value"=w407) -> ()  [unwired: 2 in, 2 out]
                n290 = property on="Range" class="Enum (strict)"("Value"=w408) -> ()  [unwired: 2 in, 2 out]
                n291 = property on="Range" class="Enum (strict)"("Value"=w414) -> ()  [unwired: 2 in, 2 out]
                n292 = property on="Range" class="Enum (strict)"("Value"=w412) -> ()  [unwired: 2 in, 2 out]
                n293 = property on="Range" class="Enum (strict)"("Value"=w411) -> ()  [unwired: 2 in, 2 out]
              }
              frame True {
              }
            }
          }
          frame #4 {
            # "Initialize AVS/zBridge"
            n294 = property on="Bridge Type" class="Enum (strict)"() -> ("Value"=w425:T61)  [unwired: 2 in, 2 out]
            n295 = case shown="\"Disabled\", Default" w425 {
              tunnel: [w431 w440 w456 refnum<visa-resource-name> refnum ("dup VISA session") refnum<visa-resource-name> refnum ("dup VISA session")] -> w424
              tunnel: [w430 w443 _ w464 errorcluster {"status"=FALSE, "code"=0, "source"=""} ("error out")] -> w423
              tunnel: [_ _ w455 _ _] -> _
              tunnel: w420 -> [_ _ _ w461 _]
              tunnel: w419 -> [_ _ _ w460 _]
              frame "AVS47A (GPIB interface)" {
                # "Set default Parameters,\n enable Autoranging"
                n296 = property on="AVS GPIB Address" class="VISAName"() -> ("Value"=w426:refnum<visa-resource-name>)  [unwired: 2 in, 2 out]
                n297 = call "AVS47IB Initialize.vi"("Instr. Descriptor (GPIB::)"=w426) -> ("VISA session"=w439:refnum<visa-resource-name>, "error out"=w427:errorcluster)  [unwired: 13 in]
                n298 = call "AVS47IB Stop.vi"("VISA session"=w439, "error in (no error)"=w427) -> ("dup VISA session"=w437:refnum<visa-resource-name>, "error out"=w429:errorcluster)  [unwired: 12 in]
                n299 = call "AVS47IB Go Remote.vi"("VISA session"=w437, "error in (no error)"=w429) -> ("dup VISA session"=w438:refnum<visa-resource-name>, "error out"=w428:errorcluster)  [unwired: 12 in]
                n300 = call "AVS47IB Configure 47IB.vi"("VISA session"=w438, "Printer Enabled (-1:no change)"=i8 0, "Buffer Enabled (-1:no change)"=i8 0, "Message Headers Included  (-1:no change)"=i8 0, "Autoranging Enabled (-1:no change)"=i8 1, "Stabilisation Delay (-1:no change)"=i8 15, "error in (no error)"=w428) -> ("dup VISA session"=w431:refnum<visa-resource-name>, "error out"=w430:errorcluster)  [unwired: 7 in]
              }
              frame "AVS47B (RS232 interface)" {
                n301 = property on="Bridge settings" class="Clust (strict)"() -> ("Value"=w447:T35)  [unwired: 2 in, 2 out]
                n302 = Unbundle By Name(w447) -> ("AVS RS232 Port"=w446:refnum<visa-resource-name>)
                n303 = call "InitPort_b.vi"("VISA resource"=w446) -> ("error out"=w442:errorcluster, "dup VISA resource"=w445:refnum<visa-resource-name>)  [unwired: 5 in]
                n304 = Type Cast(type=refnum<visa-resource-name> refnum ("dup VISA session"), x=w445) -> (*(type *) &x=w441:refnum<visa-resource-name>)
                n305 = case shown="No Error" w442 {
                  selector: w442 -> [w448 w451]
                  tunnel: w441 -> [w449 w453]
                  tunnel: [w448 w452] -> w443
                  tunnel: [w449 refnum<visa-resource-name> refnum ("dup VISA session")] -> w440
                  frame No Error {
                  }
                  frame Error {
                    n306 = VISA Close(VISA resource name=w453, error in (no error)=w451) -> (error out=w452:errorcluster)
                  }
                }
              }
              frame "AVS48SI (RS232 interface)" {
                n307 = property on="Bridge settings" class="Clust (strict)"() -> ("Value"=w459:T35)  [unwired: 2 in, 2 out]
                n308 = Unbundle By Name(w459) -> ("AVS RS232 Port"=w457:refnum<visa-resource-name>)
                n309 = call "Configure Hardware.vi"("VISA RESOURCE NAME"=w457) -> ("THREAD OUT"=w454:string)  [unwired: 14 in]
                n310 = call "Configure Sensor Wiring of CHs.vi"("THREAD IN"=w454) -> ("THREAD OUT"=w455:string)  [unwired: 10 in]
                n311 = Type Cast(type=refnum<visa-resource-name> refnum ("dup VISA session"), x=w457) -> (*(type *) &x=w456:refnum<visa-resource-name>)
              }
              frame "Impedance Bridge" {
                n312 = call "SetParFilePath.vi"("path"=w461, "zDll"=w460) -> ("error out"=w463:errorcluster, "zDll out"=w462:path)  [unwired: 8 in]
                n313 = call "StartScan.vi"("error in (no error)"=w463, "path in"=w462) -> ("error out"=w464:errorcluster)  [unwired: 8 in, 1 out]
              }
              frame "Disabled", Default {
              }
            }
            "_AVS_VISA" <- w424
            n314 = property on="Bridge status" class="Clust (strict)"("Value"=w423) -> ()  [unwired: 2 in, 2 out]
            n315 = property on="_ScanData" class="Arr (strict)"("Value"=dbl[] [0.0, 0.0, 0.0, 0.0, 0.0, 0.0, 0.0, 0.0, 0.0, 0.0] ("R_array")) -> ()  [unwired: 2 in, 2 out]
            n316 = call "ScanParameters FGV.vi"("Action"=Action."Init") -> ()  [unwired: 10 in, 1 out]
          }
          frame #5 {
            # "Generate paths for log files"
            n317 = Unbundle By Name("Data Logging Settings") -> ("Run Description"=w471:string, "Filenames Suffix"=w472:string, "Log Files Folder"=w469:path, "Log Files Name"=w475:string, "Automode Files Name"=w474:string)
            n318 = call <userlib>:"Create Dir if Non-Existant__ogtk.vi"("Directory Path"=w469) -> ("dup Directory Path"=w468:path)  [unwired: 8 in, 2 out]
            n319 = call <userlib>:"MGI Make String Filesafe.vi"("String In"=w471) -> ("Filesafe String Out"=w470:string)
            n320 = call "GeneratePaths.vi"("Filename Suffix"=w472, "Run description"=w470, "AVS_Path"=w468, "AVS_FName"=w475, "CAL_Path"=w468, "CAL_FName"=w474) -> ("Generated Log path"=w473:path, "Generated Calib path"=→"_CalibFilesPath":path)  [unwired: 8 in]
            n321 = property on="_LogFilesPath" class="Path"("Val(Sgnl)"=w473) -> ()  [unwired: 2 in, 2 out]
          }
          frame #6 {
            # "replace MessageFromProcess refnum"
            # "get MessageFromProcess refnum"
            n322 = property on="Bridge Type" class="Enum (strict)" props=["Value"]() -> ()  [unwired: 2 in, 3 out]
            n323 = call "Inst.TC.Create.vi"("Inst.TC in"=w480) -> ("Inst.TC Public Events"=w479:T62, "Inst.TC out"=w478:refnum<class "Inst.TC.lvclass">)  [unwired: 8 in, 1 out]
            n324 = Unbundle By Name(w479) -> ("MessageFromProcess"=w483:refnum<user-event>)
            n325 = register-events(reference=w482, w483) -> (reference out=w481:refnum<event-registration>)  [unwired: 3 in, 1 out]
          }
          frame #7 {
            # "Start measurements"
            n326 = Set Occurrence(w484) -> ()
          }
        }
        n327 = Bundle By Name(cluster=w342, "Inst.TC"=w344) -> (w343:T50)
      }
      event "Stop": Value Change; Application Instance Close {
        # "\"Stop\" button pressed -> Stop measuring."
        n328 = event-data() -> ()  [unwired: 1 in, 1 out]
        n329 = flat-sequence {
          tunnel: w490 -> [w494]
          tunnel: w486 -> [_]
          tunnel: w492 -> [w509]
          tunnel: w491 -> [w523]
          frame #0 {
            # "Save settings to config file"
            n330 = control-ref of="zBridge.Active Channels"() -> (w497:refnum<vi>)
            n331 = control-ref of="Bridge settings"() -> (w504:refnum<vi>)
            n332 = control-ref of="Runtime Settings"() -> (w503:refnum<vi>)
            n333 = control-ref of="CS Settings"() -> (w505:refnum<vi>)
            n334 = control-ref of="Data Logging Settings"() -> (w506:refnum<vi>)
            n335 = control-ref of="Sensor Calibrations"() -> (w502:refnum<vi>)
            n336 = control-ref of="PID Settings"() -> (w501:refnum<vi>)
            n337 = control-ref of="CS Cannel Names"() -> (w500:refnum<vi>)
            n338 = control-ref of="Channel names"() -> (w499:refnum<vi>)
            n339 = control-ref of="Curent Calibrations"() -> (w498:refnum<vi>)
            n340 = control-ref of="CS.Mode1.PID"() -> (w496:refnum<vi>)
            n341 = control-ref of="CS.Mode1.Settings"() -> (w495:refnum<vi>)
            n342 = Build Array(w497, w504, w503, w505, w506, w502, w501, w500, w499, w498, w496, w495) -> (w508:refnum<vi>[])
            n343 = call "Save Load Settings to File by Ref with path.vi"("Array of Cluster References"=w508, "Action"=enum8{"Load", "Save"}."Save", "Configuration file"=w494) -> ()  [unwired: 6 in, 1 out]
          }
          frame #1 {
            # "Free serial ports"
            n344 = control-ref of="_AVS_VISA"() -> (w510:refnum<vi>)
            n345 = control-ref of="TCS RS232 Port"() -> (w515:refnum<vi>)
            n346 = call "StopScan.vi"("path in"=w509) -> ()  [unwired: 9 in, 2 out]
            n347 = property class="VISAName"(reference=w510) -> (error out=w512:errorcluster, "Value"=w511:refnum<visa-resource-name>)  [unwired: 1 in, 1 out]
            n348 = property class="VISAName"(reference=w515) -> (error out=w513:errorcluster, "Value"=w514:refnum<visa-resource-name>)  [unwired: 1 in, 1 out]
            n349 = VISA Close(VISA resource name=w511, error in (no error)=w512) -> ()  [unwired: 1 out]
            n350 = VISA Close(VISA resource name=w514, error in (no error)=w513) -> ()  [unwired: 1 out]
          }
          frame #2 {
            w517 = u8 0 ("Disabled")
            # "Reset controls state"
            n351 = property on="Bridge Type" class="Enum (strict)"("Disabled"=w517) -> ()  [unwired: 2 in, 2 out]
            n352 = property on="AVS GPIB Address" class="VISAName"("Disabled"=w517) -> ()  [unwired: 2 in, 2 out]
            n353 = property on="AVS RS232 Port" class="VISAName"("Disabled"=w517) -> ()  [unwired: 2 in, 2 out]
            n354 = property on="TCS RS232 Port" class="VISAName"("Disabled"=w517) -> ()  [unwired: 2 in, 2 out]
            n355 = property on="CS type" class="Enum (strict)"("Disabled"=w517) -> ()  [unwired: 2 in, 2 out]
            n356 = property on="CS.QCS Device Nr" class="DigNum (strict)"("Disabled"=w517) -> ()  [unwired: 2 in, 2 out]
            n357 = property on="Start" class="Bool (strict)"("Visible"=TRUE, "Disabled"=u8 0, "Value"=FALSE ("start")) -> ()  [unwired: 2 in, 2 out]
            n358 = property on="Stop" class="Bool (strict)"("Value"=FALSE ("MainStopButton")) -> ()  [unwired: 2 in, 2 out]
          }
          frame #3 {
            w521 = u8 2 ("Disabled")
            # "Disable UI"
            n359 = property on="Top Toolbar" class="TabCtl (strict)"("Disabled"=w521) -> ()  [unwired: 2 in, 2 out]
            n360 = property on="Main Panel" class="TabCtl (strict)"("Disabled"=w521) -> ()  [unwired: 2 in, 2 out]
            n361 = property on="CS Indicators Panel" class="TabCtl (strict)"("Disabled"=w521) -> ()  [unwired: 2 in, 2 out]
            n362 = property on="Side Panel" class="TabCtl (strict)"("Disabled"=w521) -> ()  [unwired: 2 in, 2 out]
            n363 = property on="Lower Panel" class="TabCtl (strict)"("Disabled"=w521) -> ()  [unwired: 2 in, 2 out]
            n364 = property on="_String" class="Str"("Visible"=TRUE) -> ()  [unwired: 2 in, 2 out]
          }
          frame #4 {
            n365 = invoke class="App" method="Library.UndeployLibrary"("libPath"=w523) -> ()  [unwired: 4 in, 5 out]
          }
          frame #5 {
            # "Stop \nexecution"
            n366 = Stop(stop? (T)=TRUE) -> ()
          }
        }
        n367 = Unbundle By Name(w493) -> ("Variables Library"=w491:path, "zBridge dll"=w492:path, "Config File"=w490:path, "Inst.TC"=w488:refnum<class "Inst.TC.lvclass">)
        n368 = call <vilib>:"Stop.vi"("timeout in ms (-1)"=1000, "SMO"=w488) -> ("error out"=w487:errorcluster, "SMO out"=w489:refnum<class "Inst.TC.lvclass">)  [unwired: 8 in]
        n369 = call <vilib>:"Destroy.vi"("error in (no error)"=w487, "SMO"=w489) -> ("error out"=w486:errorcluster)  [unwired: 9 in]
      }
      event User Event {
        n370 = event-data() -> ("Message.Command"=w532:string, "Message.Data"=w534:variant, "Message.ID"=w528:string)  [unwired: 1 in]
        n371 = case shown="\"Set Heater\", \"setHeater\"" w532 {
          selector: w532 -> [w537 w540]
          tunnel: w534 -> [_ w549]
          tunnel: [variant ("Variant") w541] -> w533
          tunnel: [w537 w540] -> w531
          tunnel: w525 -> [w535 w539]
          tunnel: [w535 w538] -> w526
          frame Default {
          }
          frame "Set Heater", "setHeater" {
            (unwired) Inst.TC.Commands--Enum."setHeater" ("Enum")
            n372 = Variant To Data(error in=w539, type="", Variant=w549) -> (data=w547:string, error out=w544:errorcluster)
            n373 = call "From JSON Text.vim"("Data Type and Default Value"=T54 {"current"=0.0, "channel"=0} ("Set Heater"), "error in (no error)"=w544, "JSON"=w547) -> ("error out"=w543:errorcluster, "Data out"=w545:T54)  [unwired: 7 in]
            n374 = case shown="No Error" w543 {
              selector: w543 -> [w550 w575]
              tunnel: w545 -> [w558 _]
              tunnel: ["ACK" "Error"] -> w542
              tunnel: [w550 w575] -> w538
              frame No Error {
                # "mA"
                # "uA"
                n375 = Unbundle By Name(w558) -> ("channel"=w557:i32, "current"=w555:dbl)
                n376 = Multiply(x=w555, y=1000.0) -> (x*y=w554:dbl)
                n377 = To Unsigned Long Integer(number=w554) -> (unsigned 32bit integer=w552:u32)
                n378 = case shown="1" w557 {
                  tunnel: T55."x1 uA" ("Range") -> [w562 w566 w570 w574]
                  tunnel: w552 -> [w561 w565 w569 w573]
                  frame 0, Default {
                    n379 = local read "CS.I0"() -> (w560:T41)
                    n380 = Bundle By Name(cluster=w560, "I"=w561, "Range"=w562) -> (w559:T41)
                    n381 = local write "CS.I0"(w559) -> ()
                  }
                  frame 1 {
                    n382 = local read "CS.I1"() -> (w564:T41)
                    n383 = Bundle By Name(cluster=w564, "I"=w565, "Range"=w566) -> (w563:T41)
                    n384 = local write "CS.I1"(w563) -> ()
                  }
                  frame 2 {
                    n385 = local read "CS.I2"() -> (w568:T41)
                    n386 = Bundle By Name(cluster=w568, "I"=w569, "Range"=w570) -> (w567:T41)
                    n387 = local write "CS.I2"(w567) -> ()
                  }
                  frame 3 {
                    n388 = local read "CS.I3"() -> (w572:T41)
                    n389 = Bundle By Name(cluster=w572, "I"=w573, "Range"=w574) -> (w571:T41)
                    n390 = local write "CS.I3"(w571) -> ()
                  }
                }
              }
              frame Error {
              }
            }
            n391 = To Variant(anything=w542) -> (Variant=w541:variant)
          }
        }
        n392 = Unbundle By Name(w530) -> ("Inst.TC"=w529:refnum<class "Inst.TC.lvclass">)
        n393 = call-poly <userlib>:"Instrument.sendMessageToProcess.vi"("ID"=w528, "error in (no error)"=w526, "Data"=w533, "Command"=w531, "Instrument"=w529) -> ("error out"=w527:errorcluster)  [unwired: 5 in, 1 out]
      }
      event "_ScanData": Value Change {
        # "Convert 8 elements AVS\narray to 10 elements"
        # "Received new data from AVS/zBridge. Do general tasks - update indicators, calculate temperature and pass the data further to AVS/zBridge specific processing"
        n394 = event-data() -> ("NewVal"=w593:dbl[])  [unwired: 1 in]
        n395 = Unbundle By Name(w581) -> ("UpdateValuesAVS"=w579:refnum<user-event>, "UpdateValuesZBridge"=w580:refnum<user-event>)
        n396 = Unbundle By Name(w577) -> ("Calibrations Folder"=w578:path)
        n397 = for {
          tunnel: w593 -> [w622] mode=indexing
          tunnel: [w620] -> w589 mode=indexing
          n398 = Less?(x=w622, y=1e+25) -> (x < y?=w623:bool)
          n399 = Select(t=w622, s=w623, f=inf) -> (s? t:f=w620:dbl)
        }
        n400 = Index Array(array=w589) -> (element #1=→"R0":dbl, element #2=→"R1":dbl, element #3=→"R2":dbl, element #4=→"R3":dbl, element #5=→"R4":dbl, element #6=→"R5":dbl, element #7=→"R6":dbl, element #8=→"R7":dbl, element #9=→"R8":dbl, element #10=→"R9":dbl)  [unwired: 10 in]
        n401 = Array To Cluster(array=w589) -> (cluster=w583:T64)
        "R Cluster" <- w583
        n402 = Cluster To Array(cluster=w583) -> (array=w582:dbl[])
        n403 = Absolute Value(x=w582) -> (abs(x)=w590:dbl[])
        n404 = property on="Allow neg R" class="Bool (strict)"() -> ("Value"=w588:bool)  [unwired: 2 in, 2 out]
        n405 = Select(t=w582, s=w588, f=w590) -> (s? t:f=w587:dbl[])
        "R Array" <- w587
        n406 = local read "_CurCalibrations"() -> (w595:T33)
        n407 = Cluster To Array(cluster=w595) -> (array=w594:string[])
        n408 = call "Resistance to Temp no Ext.vi"("error in"=w596, "Path"=w578, "CurCalibrations"=w594, "Resistance"=w587) -> ("Temperature"=w585:dbl[])  [unwired: 1 in, 3 out]
        "T Array" <- w585
        n409 = Array To Cluster(array=w585) -> (cluster=w601:T65)
        "T Cluster" <- w601
        n410 = Unbundle(w601) -> ("Temperature[0]"=→"T0":dbl, "Temperature[1]"=→"T1":dbl, "Temperature[2]"=→"T2":dbl, "Temperature[3]"=→"T3":dbl, "Temperature[4]"=→"T4":dbl, "Temperature[5]"=→"T5":dbl, "Temperature[6]"=→"T6":dbl, "Temperature[7]"=→"T7":dbl, "Temperature[8]"=→"T8":dbl, "Temperature[9]"=→"T9":dbl)
        n411 = property on="Mode Buttons" class="RadioBtnsControl (strict)"() -> ("Value"=w600:T7)  [unwired: 2 in, 2 out]
        n412 = Array To Cluster(array=w587) -> (cluster=w586:T64)
        n413 = Array To Cluster(array=w585) -> (cluster=w584:T65)
        n414 = case shown="\"No Selection\", Default" w600 {
          tunnel: w584 -> [w635 _]
          tunnel: w586 -> [w636 _]
          frame "No Selection", Default {
            n415 = call "Current Time(double).vi"() -> ("Current Time (double)"=→"Time":dbl)  [unwired: 6 in, 1 out]
            "Small R Cluster" <- w636
            "Small T Cluster" <- w635
          }
          frame "Cursor mode" {
          }
        }
        n416 = Bundle(w587, "Temperature"=w585) -> (w598:cluster{dbl[], "Temperature":dbl[]})  [unwired: 1 in]
        n417 = property on="Bridge Type" class="Enum (strict)"() -> ("Value"=w597:T61)  [unwired: 2 in, 2 out]
        n418 = case shown="\"Impedance Bridge\"" w597 {
          tunnel: [w628 w629 w632] -> w599
          tunnel: w596 -> [w627 w629 w633]
          tunnel: w598 -> [w626 _ w631]
          tunnel: w580 -> [_ _ w630]
          tunnel: w579 -> [w625 _ _]
          frame "AVS47B (RS232 interface)", Default {
            n419 = Generate User Event(user event=w625, event data cluster=w626, error in=w627) -> (error out=w628:errorcluster)  [unwired: 1 in, 1 out]
          }
          frame "Disabled" {
          }
          frame "Impedance Bridge" {
            n420 = Generate User Event(user event=w630, event data cluster=w631, error in=w633) -> (error out=w632:errorcluster)  [unwired: 1 in, 1 out]
          }
        }
      }
      event User Event {
        # "Process data from the AVS bridge"
        n421 = event-data() -> ("R"=w642:dbl[], "T"=w641:dbl[])  [unwired: 1 in]
        n422 = property on="CS.Actual Current" class="Arr (strict)"() -> ("Value"=w643:dbl[])  [unwired: 2 in, 2 out]
        n423 = Unbundle By Name(w640) -> ("CS Automode"=w639:refnum<user-event>)
        n424 = Unbundle By Name(w638) -> ("Inst.TC"=w637:refnum<class "Inst.TC.lvclass">)
        n425 = stacked-sequence {
          tunnel: w645 -> [_ w663 w674]
          tunnel: [_ _ w690] -> w644
          tunnel: w643 -> [_ w669 w695]
          tunnel: w642 -> [w653 w667 w689]
          tunnel: w641 -> [w652 w668 w688]
          tunnel: w639 -> [w650 _ _]
          tunnel: w637 -> [_ w664 _]
          frame #0 {
            # "Filter data and add it to the data array. \nDo PID"
            n426 = property on="Runtime Settings" class="Clust (strict)"() -> ("Value"=w656:T27)  [unwired: 2 in, 2 out]
            n427 = Unbundle By Name(w656) -> ("Y_max"=w659:dbl, "Y_min"=w658:dbl, "Filter Graphs"=w657:bool)
            n428 = local read "Data Array"() -> (w654:T28)
            n429 = property on="Data Memory" class="DigNum (strict)"() -> ("Value"=w661:u16)  [unwired: 2 in, 2 out]
            n430 = call "Current Time(double).vi"() -> ("Current Time (double)"=w651:dbl)  [unwired: 6 in, 1 out]
            n431 = call "Manage Data Arrays - AVS.vi"("Y_max"=w659, "Y_min"=w658, "Filter Graph Results"=w657, "Append New Data"=TRUE, "Data In"=w654, "Curr R"=w653, "Curr T"=w652, "Curr Time"=w651, "Data Memory"=w661) -> ("Data Out"=w655:T28)  [unwired: 10 in]
            n432 = Bundle("Current Time (double)"=w651, "R"=w653, "T"=w652) -> (w662:T66)  [unwired: 1 in]
            n433 = local write "Data Array"(w655) -> ()
            n434 = Generate User Event(user event=w650, event data cluster=w662) -> ()  [unwired: 2 in, 2 out]
            n435 = Initialize Array("Ohm" ("AVS Name 0"), 10 ("dimension size")) -> (w649:string[])
            n436 = Array To Cluster(array=w649) -> (cluster=w646:T33)
            n437 = local write "Units"(w646) -> ()
          }
          frame #1 {
            n438 = property on="Sensor Calibrations" class="Clust (strict)"() -> ("Controls[]"=w666:refnum<vi>[])  [unwired: 2 in, 2 out]
            n439 = local read "Sensor Names"() -> (w665:T10)
            n440 = call "TC to PGSQL.vi"("Calibration"=w666, "I"=w669, "AVS names"=w665, "error in (no error)"=w663, "T"=w668, "R"=w667, "Inst.TC"=w664) -> ()  [unwired: 2 in, 3 out]
          }
          frame #2 {
            # "Save data to log file"
            n441 = local read "_LogFilesPath"() -> (w686:path)
            n442 = local read "_CalibFilesPath"() -> (w687:path)
            n443 = call <vilib>:"Check if File or Folder Exists.vi"("path"=w686) -> ("file or folder exists?"=w678:bool, "dup path"=w679:path)  [unwired: 8 in, 1 out]
            n444 = case shown="False" w678 {
              tunnel: w679 -> [w719 w725]
              tunnel: [w719 w725] -> w680
              tunnel: [w717 _] -> w671
              frame False {
                n445 = local read "_CurCalibrations"() -> (w716:T33)
                n446 = property on="Run Description" class="Str"() -> ("Value"=w718:string)  [unwired: 2 in, 2 out]
                n447 = Cluster To Array(cluster="Sensor Names") -> (array=w723:string[])
                n448 = Cluster To Array(cluster=w716) -> (array=w715:string[])
                n449 = Cluster To Array(cluster="CS Cannel Names") -> (array=w724:string[])
                n450 = call "Format log file header Z.vi"("Calibrations"=w715, "AVS names"=w723, "CS Names"=w724, "Run description"=w718) -> ("String"=w720:string)  [unwired: 1 in]
                n451 = Write to Text File(file (use dialog)=w719, text=w720) -> (error out=w717:errorcluster)  [unwired: 2 in, 2 out]
              }
              frame True {
              }
            }
            n452 = property on="Data Logging Settings" class="Clust (strict)"() -> ("Value"=w702:T37)  [unwired: 2 in, 2 out]
            n453 = Unbundle By Name(w702) -> ("Delimeter"=w703:string, "Date Format"=w701:string)
            n454 = call "Current Time(double).vi"() -> ("Current Time"=w672:timestamp, "Current Time (double)"=w673:dbl)  [unwired: 6 in]
            n455 = call <userlib>:"File Info__ogtk.vi"("error in (no error)"=w671, "file"=w680) -> ("error out"=w670:errorcluster, "file info"=w676:T67, "file out"=w685:path)  [unwired: 4 in]
            n456 = Unbundle By Name(w676) -> ("creation date"=w677:u32)
            n457 = Number To Exponential String(number=w673, precision (6)=i16 10) -> (E-format string=w693:string)  [unwired: 2 in]
            n458 = Format Date/Time String(time format string (%c)=w701, seconds (now)=w672) -> (date/time string=w698:string)  [unwired: 1 in]
            n459 = Number To Fractional String(number=w689) -> (F-format string=w700:string[])  [unwired: 3 in]
            n460 = Number To Fractional String(number=w688) -> (F-format string=w699:string[])  [unwired: 3 in]
            n461 = Number To Fractional String(number=w695) -> (F-format string=w697:string[])  [unwired: 3 in]
            n462 = property on="New File Interval" class="DigNum (strict)"() -> ("Value"=w681:u32)  [unwired: 2 in, 2 out]
            n463 = property on="New File Interval Units" class="Enum (strict)"() -> ("Value"=w682:enum16{"Minutes", "Hours", "Days"})  [unwired: 2 in, 2 out]
            n464 = To Time Stamp(1:w677) -> (0:w683:timestamp)
            n465 = Build Array (concatenate)(w698, w693, w700, w699, w697) -> (w696:string[])
            n466 = call "Time Elapsed time.vi"("Time Units"=w682, "Delay Time"=w681, "Time Old In"=w683) -> ("T>dT?"=w684:bool)  [unwired: 2 out]
            n467 = case shown="False" w684 {
              tunnel: [w705 w708] -> w675
              tunnel: [w704 w709] -> _
              tunnel: w685 -> [w705 _]
              tunnel: w687 -> [w704 _]
              frame False {
              }
              frame True {
                n468 = local read "Data Logging Settings"() -> (w710:T37)
                n469 = Unbundle By Name(w710) -> ("Run Description"=w706:string, "Log Files Folder"=w714:path, "Log Files Name"=w712:string, "Automode Files Name"=w713:string, "Filenames Suffix"=w711:string)
                n470 = call <userlib>:"MGI Make String Filesafe.vi"("String In"=w706) -> ("Filesafe String Out"=w707:string)
                n471 = call "GeneratePaths.vi"("Filename Suffix"=w711, "Run description"=w707, "AVS_Path"=w714, "AVS_FName"=w712, "CAL_Path"=w714, "CAL_FName"=w713) -> ("Generated Log path"=w708:path, "Generated Calib path"=w709:path)  [unwired: 8 in]
                n472 = local write "_CalibFilesPath"(w709) -> ()
                n473 = property on="_LogFilesPath" class="Path"("Val(Sgnl)"=w708) -> ()  [unwired: 2 in, 2 out]
              }
            }
            n474 = call "Write To Spreadsheet File (string) w Error.vi"("delimiter (\\t)"=w703, "append to file? (new file:F)"=TRUE, "error in"=w670, "1D data"=w696, "file path (dialog if empty)"=w675) -> ("error out"=w691:errorcluster)  [unwired: 5 in, 1 out]
            n475 = Merge Errors(w691, w674) -> (w690:errorcluster)
          }
        }
      }
      event User Event {
        # "Process data from the zBridge bridge"
        n476 = event-data() -> ("R"=w736:dbl[], "T"=w735:dbl[])  [unwired: 1 in]
        n477 = property on="CS.Actual Current" class="Arr (strict)"() -> ("Value"=w734:dbl[])  [unwired: 2 in, 2 out]
        n478 = local read "_zBridgeParText"() -> (w731:string)
        n479 = local read "_zBridgeSetNr"() -> (w737:u8)
        n480 = local read "_ZBridgeUnit"() -> (w732:string)
        n481 = Unbundle By Name(w730) -> ("CS Automode"=w729:refnum<user-event>)
        n482 = Unbundle By Name(w727) -> ("Inst.TC"=w726:refnum<class "Inst.TC.lvclass">)
        n483 = stacked-sequence {
          tunnel: w731 -> [w758 _ _]
          tunnel: w737 -> [w743 w766 _]
          tunnel: w736 -> [w741 w792 w828]
          tunnel: w735 -> [w740 w791 w827]
          tunnel: w734 -> [_ w790 _]
          tunnel: w733 -> [_ w789 _]
          tunnel: [_ w788 _] -> w728
          tunnel: w732 -> [w745 _ _]
          tunnel: w729 -> [w742 _ _]
          tunnel: w726 -> [_ _ w826]
          frame #0 {
            # "Only do PID after measuring\non selected channel( or any \nchannel if -1 is selected)"
            n484 = local read "zBridge params"() -> (w744:T19)
            n485 = local read "Units"() -> (w746:T13)
            n486 = Cluster To Array(cluster=w746) -> (array=w749:string[])
            n487 = Cluster To Array(cluster=w744) -> (array=w759:string[])
            n488 = Replace Array Subset(array=w749, new element=w745, index=w743) -> (w748:string[])
            n489 = Replace Array Subset(array=w759, new element=w758, index=w743) -> (w760:string[])
            n490 = Array To Cluster(array=w748) -> (cluster=→"Units":T68)
            n491 = Array To Cluster(array=w760) -> (cluster=→"zBridge params":T69)
            n492 = property on="Runtime Settings" class="Clust (strict)"() -> ("Value"=w752:T27)  [unwired: 2 in, 2 out]
            n493 = Unbundle By Name(w752) -> ("Y_max"=w755:dbl, "Y_min"=w754:dbl, "Filter Graphs"=w753:bool)
            n494 = local read "Data Array"() -> (w750:T28)
            n495 = property on="Data Memory" class="DigNum (strict)"() -> ("Value"=w757:u16)  [unwired: 2 in, 2 out]
            n496 = call "Current Time(double).vi"() -> ("Current Time (double)"=w738:dbl)  [unwired: 6 in, 1 out]
            n497 = call "Manage Data Arrays - zBridge.vi"("Y_max"=w755, "Y_min"=w754, "Filter Graph Results"=w753, "Append New Data"=TRUE, "Data In"=w750, "Curr R"=w741, "Curr T"=w740, "Curr Time"=w738, "Channel"=w743, "Data Memory"=w757) -> ("Data Out"=w751:T28)  [unwired: 9 in]
            n498 = local write "Data Array"(w751) -> ()
            n499 = Bundle("Current Time (double)"=w738, "R"=w741, "T"=w740) -> (w739:T66)  [unwired: 1 in]
            n500 = Generate User Event(user event=w742, event data cluster=w739) -> ()  [unwired: 2 in, 2 out]
          }
          frame #1 {
            n501 = local read "_LogFilesPath"() -> (w769:path)
            n502 = local read "Data Logging Settings"() -> (w787:T37)
            n503 = call <userlib>:"Strip Path Extension - Path__ogtk.vi"("path"=w769) -> ("root"=w770:string, "extension"=w773:string)
            n504 = Format Into String(format string="_%d", initial string=w770, w766) -> (resulting string=w771:string)  [unwired: 1 in, 1 out]
            n505 = Concatenate Strings(w771, "." ("string"), w773) -> (w768:string)
            n506 = Unbundle By Name(w787) -> ("Delimeter"=w803:string, "Date Format"=w802:string)
            n507 = String To Path(string=w768) -> (path=w767:path)
            n508 = call <vilib>:"Check if File or Folder Exists.vi"("path"=w767) -> ("file or folder exists?"=w778:bool, "dup path"=w779:path)  [unwired: 8 in, 1 out]
            n509 = case shown="False" w778 {
              tunnel: w779 -> [w823 w825]
              tunnel: [w823 w825] -> w780
              tunnel: [w817 _] -> w763
              frame False {
                n510 = local read "CS Cannel Names"() -> (w821:T31)
                n511 = local read "_CurCalibrations"() -> (w816:T33)
                n512 = local read "Sensor Names"() -> (w822:T10)
                n513 = Cluster To Array(cluster=w816) -> (array=w815:string[])
                n514 = property on="Run Description" class="Str"() -> ("Value"=w818:string)  [unwired: 2 in, 2 out]
                n515 = Cluster To Array(cluster=w822) -> (array=w819:string[])
                n516 = Cluster To Array(cluster=w821) -> (array=w820:string[])
                n517 = call "Format log file header Z.vi"("Calibrations"=w815, "AVS names"=w819, "CS Names"=w820, "Run description"=w818) -> ("String"=w824:string)  [unwired: 1 in]
                n518 = Write to Text File(file (use dialog)=w823, text=w824) -> (error out=w817:errorcluster)  [unwired: 2 in, 2 out]
              }
              frame True {
              }
            }
            n519 = call "Current Time(double).vi"() -> ("Current Time"=w764:timestamp, "Current Time (double)"=w765:dbl)  [unwired: 6 in]
            n520 = Number To Exponential String(number=w765, precision (6)=i16 10) -> (E-format string=w795:string)  [unwired: 2 in]
            n521 = Format Date/Time String(time format string (%c)=w802, seconds (now)=w764) -> (date/time string=w799:string)  [unwired: 1 in]
            n522 = Number To Exponential String(number=w792) -> (E-format string=w801:string[])  [unwired: 3 in]
            n523 = Number To Engineering String(4:w791) -> (0:w800:string[])  [unwired: 3 in]
            n524 = Number To Fractional String(number=w790) -> (F-format string=w798:string[])  [unwired: 3 in]
            n525 = call <userlib>:"File Info__ogtk.vi"("error in (no error)"=w763, "file"=w780) -> ("error out"=w762:errorcluster, "file info"=w776:T67, "file out"=w785:path)  [unwired: 4 in]
            n526 = Unbundle By Name(w776) -> ("creation date"=w777:u32)
            n527 = Build Array (concatenate)(w799, w795, w801, w800, w798) -> (w797:string[])
            n528 = local read "_CalibFilesPath"() -> (w786:path)
            n529 = property on="New File Interval" class="DigNum (strict)"() -> ("Value"=w781:u32)  [unwired: 2 in, 2 out]
            n530 = property on="New File Interval Units" class="Enum (strict)"() -> ("Value"=w782:enum16{"Minutes", "Hours", "Days"})  [unwired: 2 in, 2 out]
            n531 = To Time Stamp(1:w777) -> (0:w783:timestamp)
            n532 = call "Time Elapsed time.vi"("Time Units"=w782, "Delay Time"=w781, "Time Old In"=w783) -> ("T>dT?"=w784:bool)  [unwired: 2 out]
            n533 = case shown="True" w784 {
              tunnel: [w805 w808] -> w775
              tunnel: [w804 w810] -> _
              tunnel: w785 -> [w805 _]
              tunnel: w786 -> [w804 _]
              frame False {
              }
              frame True {
                n534 = local read "Data Logging Settings"() -> (w811:T37)
                n535 = Unbundle By Name(w811) -> ("Run Description"=w807:string, "Filenames Suffix"=w809:string, "Log Files Folder"=w814:path, "Log Files Name"=w812:string, "Automode Files Name"=w813:string)
                n536 = call <userlib>:"MGI Make String Filesafe.vi"("String In"=w807) -> ("Filesafe String Out"=w806:string)
                n537 = call "GeneratePaths.vi"("Filename Suffix"=w809, "Run description"=w806, "AVS_Path"=w814, "AVS_FName"=w812, "CAL_Path"=w814, "CAL_FName"=w813) -> ("Generated Log path"=w808:path, "Generated Calib path"=w810:path)  [unwired: 8 in]
                n538 = local write "_CalibFilesPath"(w810) -> ()
                n539 = property on="_LogFilesPath" class="Path"("Val(Sgnl)"=w808) -> ()  [unwired: 2 in, 2 out]
              }
            }
            n540 = call "Write To Spreadsheet File (string) w Error.vi"("delimiter (\\t)"=w803, "append to file? (new file:F)"=TRUE, "error in"=w762, "1D data"=w797, "file path (dialog if empty)"=w775) -> ("error out"=w793:errorcluster)  [unwired: 5 in, 1 out]
            n541 = Merge Errors(w793, w789) -> (w788:errorcluster)
          }
          frame #2 {
            n542 = property on="Sensor Calibrations" class="Clust (strict)"() -> ("Controls[]"=w830:refnum<vi>[])  [unwired: 2 in, 2 out]
            n543 = local read "Sensor Names"() -> (w829:T10)
            n544 = call "TC to PGSQL.vi"("Calibration"=w830, "AVS names"=w829, "T"=w827, "R"=w828, "Inst.TC"=w826) -> ()  [unwired: 4 in, 3 out]
          }
        }
      }
      event User Event {
        # "Current source automatic mode"
        n545 = event-data() -> ("R"=w837:dbl[], "T"=w838:dbl[], "Time"=w832:dbl)  [unwired: 1 in, 4 out]
        n546 = local read "CS.Mode"() -> (w836:T39)
        n547 = Unbundle By Name(w835) -> ("CallExtVI"=w834:refnum<user-event>, "TempStabilized"=w833:refnum<user-event>)
        n548 = case shown="\"Mode2\"" w836 {
          tunnel: w838 -> [_ w842 w917]
          tunnel: w837 -> [_ w843 w918]
          tunnel: w834 -> [_ w845 _]
          tunnel: w833 -> [_ w844 _]
          tunnel: w832 -> [_ w841 _]
          frame "Manual", Default {
          }
          frame "Mode 1" {
            n549 = call <userlib>:"MGI Change Detector (T).vi"("Value"="CS.Mode1.Start") -> ("Changed?"=w839:bool)
            n550 = case shown="True" "CS.Mode1.Start" {
              tunnel: w845 -> [_ w858]
              tunnel: w844 -> [_ w857]
              tunnel: w843 -> [_ w856]
              tunnel: w842 -> [_ w855]
              tunnel: w841 -> [_ w852]
              tunnel: w839 -> [_ w846]
              frame False {
              }
              frame True {
                # "Check if PID error (SP-PV)==0"
                # "Check if temperature\nis stabilized"
                # "T sabilized?"
                # "If TCS auto mode enabled and temperature is not changing => fire TempStabilized event to save log and set new CS point. Otherwise do PID (if enabled)."
                # "Check if stabilization delay time \nis elapsed"
                n551 = property on="R/T?" class="Enum (strict)"() -> ("Value"=w854:enum16{"Resistance", "Temperature"})  [unwired: 2 in, 2 out]
                n552 = case shown="\"Temperature\"" w854 {
                  tunnel: [w873 w874] -> w851
                  tunnel: w856 -> [w873 _]
                  tunnel: w855 -> [_ w874]
                  frame "Resistance", Default {
                  }
                  frame "Temperature" {
                  }
                }
                n553 = property on="Bridge Channel" class="DigNum (strict)"() -> ("Value"=w850:i32)  [unwired: 2 in, 2 out]
                n554 = Index Array(array=w851, index=w850) -> (element=w849:dbl)
                n555 = local read "CS.Mode1.PID Error"() -> (w865:dbl)
                n556 = property on="FB on 2" class="Enum (strict)"() -> ("Value"=w847:enum16{"0", "1", "2", "3"})  [unwired: 2 in, 2 out]
                n557 = local read "_CSMode1List[i]"() -> (w859:T23[])
                n558 = local read "_TimeOld"() -> (w871:dbl)
                n559 = property on="Delay Time" class="DigNum (strict)"() -> ("Value"=w861:dbl)  [unwired: 2 in, 2 out]
                n560 = property on="N averages" class="DigNum (strict)"() -> ("Value"=w848:i32)  [unwired: 2 in, 2 out]
                n561 = property on="T stability" class="DigNum (strict)"() -> ("Value"=w860:dbl)  [unwired: 2 in, 2 out]
                n562 = Equal To 0?(x=w865) -> (x = 0?=w863:bool)
                n563 = call "Derivatives Pt by Pt.vi"("initialize"=w846, "accuracy (%)"=w860, "Time"=w852, "Data"=w849, "Points to avg"=w848) -> ("Stable?"=w864:bool, "Stability (%)"=→"CS.Mode1.Slope":dbl, "dt (s)"=w868:dbl)  [unwired: 2 in]
                n564 = Index Array(array=w859, index=w847) -> (element=w872:T23)
                n565 = call "Time Elapsed dbl.vi"("Delay Time"=w861, "Time Old In"=w871) -> ("T>dT?"=w853:bool, "Delta T"=→"CS.Mode1.Timer":dbl, "Time New Out"=w870:dbl)  [unwired: 1 in]
                n566 = Compound Arithmetic op=AND(w853, w863, w864) -> (w866:bool)
                "CS.Mode1.PID Stabilized?" <- w866
                n567 = property on="Enable PID" class="Bool (strict)"() -> ("Value"=w862:bool)  [unwired: 2 in, 2 out]
                n568 = case shown="False" w866 {
                  tunnel: w870 -> [_ w894]
                  tunnel: w868 -> [w890 _]
                  tunnel: w862 -> [w880 _]
                  tunnel: w872 -> [w888 _]
                  tunnel: w859 -> [w885 _]
                  tunnel: w847 -> [w878 _]
                  tunnel: w858 -> [_ w892]
                  tunnel: w857 -> [_ w891]
                  tunnel: w849 -> [w877 _]
                  tunnel: w846 -> [w875 _]
                  frame False {
                    # "Temperature is not stable. If enabled, do PID regulation"
                    n569 = local read "CS.Current Value"() -> (w882:dbl[])
                    n570 = Index Array(array=w882, index=w878) -> (element=w883:dbl)
                    n571 = Multiply(x=1000.0, y=w883) -> (x*y=w881:dbl)
                    n572 = call "PID control incremental.vi"("Process Variable"=w877, "dt"=w890, "Setpoint"=w888, "PID Settings"="CS.Mode1.PID Settings", "I in"=w881, "PID Enabled"=w880, "Reset"=w875) -> ("PID output I"=→"Waveform Chart":T22, "err out"=→"CS.Mode1.PID Error":dbl, "I out"=w887:dbl)  [unwired: 9 in, 1 out]
                    n573 = Replace Array Subset(array=w885, new element=w887, index=w878) -> (→"CS.Automode Current":T23[])
                  }
                  frame True {
                    # "Temperature is stable & automode is on"
                    n574 = case shown="False" "CS.Mode1.Call VI?" {
                      tunnel: w894 -> [w897 _]
                      tunnel: w892 -> [_ w898]
                      tunnel: w891 -> [w895 _]
                      frame False {
                        # "External VI call disabled -> proceed\nwith automode"
                        n575 = local write "_TimeOld"(w897) -> ()
                        n576 = Generate User Event(user event=w895, event data cluster=TRUE ("event data")) -> ()  [unwired: 2 in, 2 out]
                      }
                      frame True {
                        # "Call external VI"
                        n577 = Generate User Event(user event=w898, event data cluster="" ("event data")) -> ()  [unwired: 2 in, 2 out]
                      }
                    }
                  }
                }
              }
            }
          }
          frame "Mode2" {
            n578 = Unbundle By Name("CS.Mode2.Settings") -> ("Hysteresis"=w900:u8, "Bridge Channel"=w901:i32, "FB on"=w902:enum16{"Resistance", "Temperature"})
            n579 = case shown="\"Resistance\", Default" w902 {
              tunnel: [w920 w921] -> w916
              tunnel: w918 -> [w920 _]
              tunnel: w917 -> [_ w921]
              frame "Resistance", Default {
              }
              frame "Temperature" {
              }
            }
            n580 = Index Array(array=w916, index=w901) -> (element=w915:dbl)
            n581 = local read "CS.Mode2.List"() -> (w914:dbl[][])
            n582 = call "Currents-Temp list  - T in range-.vi"("List in"=w914, "T"=w915, "T1 index"=1, "T0 index"=0, "Hysteresis"=w900) -> ("List index"=w908:i32, "I_out"=w907:dbl[])  [unwired: 1 out]
            n583 = case shown="True" "CS.Mode2.Start" {
              tunnel: w907 -> [_ w919]
              frame False {
              }
              frame True {
                n584 = local write "CS.Automode Current"(w919) -> ()
              }
            }
            n585 = Initialize Array(FALSE, 16 ("dimension size")) -> (w911:bool[])
            n586 = Replace Array Subset(array=w911, new element=TRUE ("new element/subarray"), index=w908) -> (→"CS.Mode2.Row":bool[])
          }
        }
      }
      event User Event {
        n587 = event-data() -> ()  [unwired: 1 in, 5 out]
        n588 = Unbundle By Name(w924) -> ("TempStabilized"=w923:refnum<user-event>)
        n589 = local read "_ExtVIReference"() -> (w928:refnum<vi>)
        n590 = call "GetExtVIStatus.vi"("vi reference in"=w928) -> ("vi reference out"=w925:refnum<vi>, "Exec.State"=w927:T46, "Finished?"=w926:bool)
        n591 = case shown="\"Idle\"" w927 {
          tunnel: w926 -> [_ _]
          tunnel: w925 -> [_ w930]
          tunnel: w923 -> [_ w929]
          frame "Bad", Default {
          }
          frame "Idle" {
            n592 = local read "VI called?"() -> (w931:bool)
            n593 = case shown="False" w931 {
              tunnel: w930 -> [w933 _]
              tunnel: w929 -> [_ w940]
              frame False {
                n594 = property on="_ScanData" class="Arr (strict)"() -> ("Value"=w936:dbl[])  [unwired: 2 in, 2 out]
                n595 = property on="T Array" class="Arr (strict)"() -> ("Value"=w937:dbl[])  [unwired: 2 in, 2 out]
                n596 = property on="CS.Current Value" class="Arr (strict)"() -> ("Value"=w938:dbl[])  [unwired: 2 in, 2 out]
                n597 = Format Date/Time String() -> (date/time string=w935:string)  [unwired: 3 in]
                n598 = Bundle("date/time string"=w935, "Value"=w936, "Value"=w937, "Value"=w938) -> (w934:T70)  [unwired: 1 in]
                n599 = call "CallExtVI.vi"("vi reference in"=w933, "Cluster"=w934) -> ()  [unwired: 1 out]
                "VI called?" <- TRUE ("VI called?")
              }
              frame True {
                n600 = call "Current Time(double).vi"() -> ("Current Time (double)"=w939:dbl)  [unwired: 6 in, 1 out]
                n601 = Generate User Event(user event=w940, event data cluster=TRUE ("event data")) -> ()  [unwired: 2 in, 2 out]
                n602 = local write "_TimeOld"(w939) -> ()
              }
            }
          }
        }
      }
      event User Event {
        # "CS automode\nT is stabilized"
        n603 = event-data() -> ("TempStabilized"=w944:bool)  [unwired: 1 in, 4 out]
        n604 = stacked-sequence {
          tunnel: w945 -> [w951 _]
          tunnel: [w952 _] -> w943
          tunnel: w944 -> [_ w973]
          frame #0 {
            # "Step1: Save R,T,I values to calibration file. Make screenshot when creating the calibration file."
            n605 = property on="_CalibFilesPath" class="Path"() -> ("Value"=w947:path)  [unwired: 2 in, 2 out]
            n606 = call <userlib>:"File Exists - Scalar__ogtk.vi"("file path"=w947) -> ("exists"=w948:bool)  [unwired: 6 in, 1 out]
            n607 = case shown="False" w948 {
              tunnel: w947 -> [w963 w972]
              tunnel: [w963 w972] -> w946
              frame False {
                n608 = local read "CS Cannel Names"() -> (w969:T31)
                n609 = local read "_CurCalibrations"() -> (w960:T33)
                n610 = local read "Sensor Names"() -> (w970:T10)
                n611 = property on="Run Description" class="Str"() -> ("Value"=w966:string)  [unwired: 2 in, 2 out]
                n612 = Cluster To Array(cluster=w960) -> (array=w959:string[])
                n613 = Cluster To Array(cluster=w970) -> (array=w967:string[])
                n614 = Cluster To Array(cluster=w969) -> (array=w968:string[])
                n615 = call "Format log file header Z.vi"("Calibrations"=w959, "AVS names"=w967, "CS Names"=w968, "Run description"=w966) -> ("String"=w971:string)  [unwired: 1 in]
                n616 = control-ref of="This VI"() -> (w965:refnum<vi>)
                n617 = Write to Text File(file (use dialog)=w963, text=w971) -> ()  [unwired: 2 in, 3 out]
                n618 = invoke class="VI" method="FP.Get Image"(reference=w965) -> ("image data"=w964:T71)  [unwired: 5 in, 5 out]
                n619 = call <userlib>:"Convert File Extension (Path)__ogtk.vi"("new ending (none)"="png" ("name or relative path"), "file name"=w963) -> ("new filename"=w962:path)  [unwired: 1 out]
                n620 = call <vilib>:"Write PNG File.vi"("image data"=w964, "path to PNG file"=w962) -> ()  [unwired: 8 in, 2 out]
              }
              frame True {
              }
            }
            n621 = local write "VI called?"(FALSE ("VI called?")) -> ()
            n622 = property on="Data Logging Settings" class="Clust (strict)"() -> ("Value"=w955:T37)  [unwired: 2 in, 2 out]
            n623 = Unbundle By Name(w955) -> ("Date Format"=w956:string, "Delimeter"=w953:string)
            n624 = property on="R" class="Clust (strict)"() -> ("Value"=w954:T14)  [unwired: 2 in, 2 out]
            n625 = property on="T" class="Clust (strict)"() -> ("Value"=w958:T9)  [unwired: 2 in, 2 out]
            n626 = property on="CS.Current Value" class="Arr (strict)"() -> ("Value"=w957:dbl[])  [unwired: 2 in, 2 out]
            n627 = call "Write to cal log file.vi"("Value 2"=w957, "Date/Time Format"=w956, "Value 3"=w958, "Value"=w954, "Delimeter"=w953, "Value 4"=w946) -> ("error out"=w950:errorcluster)  [unwired: 1 out]
            n628 = Merge Errors(w950, w951) -> (w952:errorcluster)
          }
          frame #1 {
            # "Step 2: Sweep through the currents list"
            n629 = case shown="True" w973 {
              frame False {
              }
              frame True {
                n630 = local read "CS.Mode1.List:Count"() -> (w975:i32)
                n631 = local read "CS.Mode1.List:Index"() -> (w976:i32)
                n632 = Less?(x=w976, y=w975) -> (x < y?=w974:bool)
                n633 = case shown="False" w974 {
                  frame False {
                    n634 = property on="CS Mode" class="Enum (strict)"("Val(Sgnl)"=CS_mode."Manual" ("CS Mode")) -> ()  [unwired: 2 in, 2 out]
                  }
                  frame True {
                    n635 = property on="CS.Mode1.List:Next" class="Bool (strict)"("Val(Sgnl)"=TRUE) -> ()  [unwired: 2 in, 2 out]
                  }
                }
              }
            }
          }
        }
      }
      event User Event {
        # "Disable controls for disabled channels"
        n636 = event-data() -> ()  [unwired: 1 in, 5 out]
        n637 = Unbundle By Name(w980) -> ("zBridge dll"=w979:path)
        n638 = property on="Bridge Type" class="Enum (strict)"() -> ("Value"=w988:T61)  [unwired: 2 in, 2 out]
        n639 = case shown="\"AVS47B (RS232 interface)\"" w988 {
          tunnel: [w998 w1010 w1018] -> w987
          tunnel: w979 -> [_ w1009 _]
          frame Default {
            n640 = property on="Runtime Settings" class="Clust (strict)"() -> ("Value"=w1002:T27)  [unwired: 2 in, 2 out]
            n641 = Unbundle By Name(w1002) -> ("Read AVS channels from"=w1000:i8, "Last Channel"=w1001:i8)
            n642 = for {
              N: 10 -> [_]
              tunnel: w1001 -> [w1004]
              tunnel: w1000 -> [w1005]
              tunnel: [w1003] -> w998 mode=indexing
              i -> [w1006]
              n643 = Less Or Equal?(x=w1005, y=w1006) -> (x <= y?=w1008:bool)
              n644 = Less Or Equal?(x=w1006, y=w1004) -> (x <= y?=w1007:bool)
              n645 = And(x=w1008, y=w1007) -> (x .and. y?=w1003:bool)
            }
          }
          frame "Impedance Bridge" {
            n646 = for {
              N: 10 -> [_]
              tunnel: [w1013] -> w1011 mode=indexing
              tunnel: w1009 -> [w1014]
              i -> [w1016]
              n647 = call "GetByteParam.vi"("ParNo"=u8 0, "SetNo"=w1016, "zDll"=w1014) -> ("return type"=w1013:u8)  [unwired: 6 in, 2 out]
            }
            n648 = Greater Than 0?(x=w1011) -> (x > 0?=w1010:bool[])
          }
          frame "AVS47B (RS232 interface)" {
            n649 = local read "zBridge.Active Channels"() -> (w1017:T21)
            n650 = Cluster To Array(cluster=w1017) -> (array=w1018:bool[])
          }
        }
        n651 = control-ref of="zBridge.Active Channels"() -> (w994:refnum<vi>)
        n652 = control-ref of="AVS Exc&Ranges"() -> (w990:refnum<vi>)
        n653 = control-ref of="R"() -> (w995:refnum<vi>)
        n654 = control-ref of="Sensor Calibrations"() -> (w996:refnum<vi>)
        n655 = control-ref of="T"() -> (w997:refnum<vi>)
        n656 = control-ref of="uPlots"() -> (w991:refnum<vi>)
        n657 = control-ref of="AVS names"() -> (w989:refnum<vi>)
        n658 = control-ref of="zBridge params"() -> (w986:refnum<vi>)
        n659 = control-ref of="zBridge.Scan Phase"() -> (w985:refnum<vi>)
        n660 = control-ref of="Units"() -> (w984:refnum<vi>)
        n661 = control-ref of="AVS names small"() -> (w983:refnum<vi>)
        n662 = control-ref of="Small R Cluster"() -> (w982:refnum<vi>)
        n663 = control-ref of="Small T Cluster"() -> (w981:refnum<vi>)
        n664 = Build Array(w994, w990, w995, w996, w997, w991, w989, w986, w985, w984, w983, w982, w981) -> (w992:refnum<vi>[])
        n665 = Array Size(array=w992) -> (size(s)=w993:i32)
        n666 = for {
          N: w993 -> [_]
          tunnel: w992 -> [w1022] mode=indexing
          tunnel: w987 -> [w1019]
          n667 = property class="Clust"(reference=w1022) -> ("Controls[]"=w1020:refnum<vi>[])  [unwired: 1 in, 2 out]
          n668 = Array Size(array=w1020) -> (size(s)=w1021:i32)
          n669 = for {
            N: w1021 -> [_]
            tunnel: w1020 -> [w1024] mode=indexing
            tunnel: w1019 -> [w1023] mode=indexing
            n670 = case shown="True" w1023 {
              tunnel: w1024 -> [w1025 w1030]
              frame False {
                n671 = property class="Ctl"(reference=w1025, "Disabled"=u8 2) -> ("ClassName"=w1026:string)  [unwired: 1 in, 2 out]
                n672 = case shown="\"Boolean\"" w1026 {
                  tunnel: w1025 -> [_ w1029 _]
                  frame "False", Default {
                  }
                  frame "Boolean" {
                    n673 = property class="Ctl"(reference=w1029, "Value"=FALSE) -> ()  [unwired: 1 in, 2 out]
                  }
                  frame "Ring" {
                  }
                }
              }
              frame True {
                n674 = property class="Ctl"(reference=w1030, "Disabled"=u8 0) -> ("ClassName"=w1031:string)  [unwired: 1 in, 2 out]
                n675 = case shown="\"False\", Default" w1031 {
                  tunnel: w1030 -> [_ w1034]
                  frame "False", Default {
                  }
                  frame "Boolean" {
                    n676 = property class="Ctl"(reference=w1034, "Value"=TRUE) -> ()  [unwired: 1 in, 2 out]
                  }
                }
              }
            }
          }
        }
      }
      event Mouse Down? {
        n677 = event-data() -> ("CtlRef"=w1036:refnum<vi>, "Mods.Double Click"=w1035:bool)  [unwired: 1 in]
        n678 = disable-structure shown="Enabled" {
          disable-tunnel: w1035 -> [w1039 _]
          disable-tunnel: w1036 -> [w1038 _]
          frame Enabled {
            n679 = case shown="True" w1039 {
              tunnel: w1038 -> [_ w1058]
              frame False {
              }
              frame True {
                w1054 = 128  # call and forget
                n680 = property class="Ctl"(reference=w1058) -> ("Label.Text"=w1057:string)  [unwired: 1 in, 2 out]
                n681 = local read "Sensor Names"() -> (w1045:T10)
                n682 = call <userlib>:"Slice String 1__ogtk.vi"("Subset (i:j)"="-1", "String"=w1057) -> ("Substring (String[i:j])"=w1055:string)  [unwired: 7 in]
                n683 = Decimal String To Number(string=w1055) -> (number=w1040:i32)  [unwired: 2 in, 1 out]
                n684 = Cluster To Array(cluster=w1045) -> (array=w1044:string[])
                n685 = Index Array(array=w1044, index=w1040) -> (element=w1043:string)
                n686 = vi-ref "Text Popup.vi"() -> (w1051:refnum<vi>)
                n687 = property class="VI"(reference=w1051) -> (error out=w1052:errorcluster, "Name"=w1053:string)  [unwired: 1 in, 1 out]
                n688 = Open VI Reference(type specifier VI Refnum (for type only)=refnum<vi> refnum, vi path=w1053, options=w1054, error in (no error)=w1052) -> (vi reference=w1050:refnum<vi>, error out=w1047:errorcluster)  [unwired: 2 in]
                n689 = control-ref of="T Array"() -> (w1041:refnum<vi>)
                n690 = control-ref of="R Array"() -> (w1042:refnum<vi>)
                n691 = call-by-ref "Start Asynchronous Call"(reference=w1050, error in=w1047, "Title"=w1043, "R_array"=w1042, "T_array"=w1041, "Index"=w1040) -> (reference out=w1048:refnum<vi>, error out=w1046:errorcluster)  [unwired: 16 in]
                n692 = Close Reference(reference=w1048, error in (no error)=w1046) -> ()  [unwired: 1 out]
              }
            }
          }
          frame Disabled {
          }
        }
        n693 = event-data() -> ()  [unwired: 2 in, 1 out]
      }
      event "_LogFilesPath": Value Change {
        # "Modify window title to show measurement information"
        n694 = event-data() -> ("NewVal"=w1068:path)  [unwired: 1 in, 5 out]
        n695 = property class="App"() -> ("App.Dir"=w1060:path)  [unwired: 2 in, 2 out]
        n696 = property on="Run Description" class="Str"() -> ("Value"=w1061:string)  [unwired: 2 in, 2 out]
        n697 = property on="Bridge Type" class="Enum (strict)"() -> ("RingText.Text"=w1062:string)  [unwired: 2 in, 2 out]
        n698 = property on="CS type" class="Enum (strict)"() -> ("RingText.Text"=w1063:string)  [unwired: 2 in, 2 out]
        n699 = Path To String(path=w1068) -> (string=w1064:string)
        n700 = Strip Path(path=w1060) -> (name=w1059:string)  [unwired: 1 out]
        n701 = Format Into String(format string="%s - %s - %s - %s   (%s)", w1059, w1061, w1062, w1063, w1064) -> (resulting string=w1066:string)  [unwired: 2 in, 1 out]
        n702 = control-ref of="This VI"() -> (w1069:refnum<vi>)
        n703 = property class="VI"(reference=w1069, "Front Panel.Title"=w1066) -> ()  [unwired: 1 in, 2 out]
      }
      event "Reload Calibrations", "Bridge settings.Calibrations Folder": Value Change {
        # "Refresh the list of calibration files"
        n704 = event-data() -> ()  [unwired: 1 in, 1 out]
        n705 = property on="Calibrations Folder" class="Path"() -> ("Value"=w1070:path)  [unwired: 2 in, 2 out]
        n706 = control-ref of="Sensor Calibrations"() -> (w1079:refnum<vi>)
        n707 = control-ref of="_CurCalibrations"() -> (w1073:refnum<vi>)
        n708 = control-ref of="Calibrations Folder"() -> (w1077:refnum<vi>)
        n709 = control-ref of="_QuickConvertCal"() -> (w1076:refnum<vi>)
        n710 = control-ref of="Sensor 1"() -> (w1078:refnum<vi>)
        n711 = Bundle By Name(cluster=w1072, "Calibrations Folder"=w1070) -> (w1071:T50)
        n712 = call "ReloadCalibrations.vi"("error in (no error)"=w1075, "Quick convert sensors"=w1076, "CurCalibrations"=w1073, "Calibration files path"=w1077, "Channel1 sensors"=w1078, "Channels list"=w1079) -> ("error out"=w1074:errorcluster)  [unwired: 1 out]
      }
      event Value Change {
        w1086 = refnum<vi> refnum  # XYGraph
        # "Show cursor on plot is \"Cursor\" or \"Delete points\" mode is enabled"
        # "!!NOTE:This routine assumes that XY graph is control #0 on tab page!!"
        n713 = event-data() -> ("NewVal"=w1082:T7)  [unwired: 1 in, 5 out]
        n714 = property on="Channels Panel" class="TabCtl (strict)"() -> ("Pages"=w1090:refnum<vi>[], "Value"=w1089:T8)  [unwired: 2 in, 2 out]
        n715 = Index Array(array=w1090, index=w1089) -> (element=w1088:refnum<vi>)
        n716 = property class="Page"(reference=w1088) -> ("ControlsOnPage"=w1083:refnum<vi>[])  [unwired: 1 in, 2 out]
        n717 = Index Array(array=w1083, index=0) -> (element=w1087:refnum<vi>)
        n718 = Type Cast(type=w1086, x=w1087) -> (*(type *) &x=w1081:refnum<vi>)
        n719 = case shown="\"Erase range\"" w1082 {
          tunnel: w1081 -> [w1091 w1100 w1108 w1116]
          frame "No Selection", Default {
            n720 = property class="XYGraph"(reference=w1091, "Active Cursor"=u32 0, "Cursor.Visible"=FALSE) -> (reference out=w1094:refnum<vi>)  [unwired: 1 in, 1 out]
            n721 = property class="XYGraph"(reference=w1094, "Active Cursor"=u32 1, "Cursor.Visible"=FALSE) -> ()  [unwired: 1 in, 2 out]
          }
          frame "Erase range" {
            n722 = property class="XYGraph"(reference=w1100, "Active Cursor"=u32 0, "Cursor.Visible"=TRUE, "Cursor.Cursor Color"=u32 16777062, "Cursor.Cursor Index"=0, "ActPaletteTool"=0 ("Palette:Active Tool")) -> (reference out=w1103:refnum<vi>)  [unwired: 1 in, 1 out]
            n723 = property class="XYGraph"(reference=w1103, "Active Cursor"=u32 1, "Cursor.Visible"=TRUE, "Cursor.Cursor Color"=u32 6618880) -> ()  [unwired: 1 in, 2 out]
          }
          frame "Cursor mode" {
            n724 = property class="XYGraph"(reference=w1108, "Active Cursor"=u32 0, "Cursor.Visible"=TRUE, "Cursor.Cursor Color"=u32 6618880, "ActPaletteTool"=0 ("Palette:Active Tool")) -> (reference out=w1111:refnum<vi>)  [unwired: 1 in, 1 out]
            n725 = property class="XYGraph"(reference=w1111, "Active Cursor"=u32 1, "Cursor.Visible"=FALSE) -> ()  [unwired: 1 in, 2 out]
          }
          frame "Erase point" {
            n726 = property class="XYGraph"(reference=w1116, "Active Cursor"=u32 0, "Cursor.Visible"=TRUE, "Cursor.Cursor Color"=u32 16777062, "ActPaletteTool"=0 ("Palette:Active Tool")) -> (reference out=w1119:refnum<vi>)  [unwired: 1 in, 1 out]
            n727 = property class="XYGraph"(reference=w1119, "Active Cursor"=u32 1, "Cursor.Visible"=FALSE) -> ()  [unwired: 1 in, 2 out]
          }
        }
      }
      event "R-Plot 0", "R-Plot 1", "R-Plot 2", "R-Plot 3", "R-Plot 4", "R-Plot 5", "R-Plot 6", "R-Plot 7", "R-Plot 8", "R-Plot 9": Mouse Down? {
        # "Disabled"
        n728 = event-data() -> ("CtlRef"=w1125:refnum<vi>, "Button"=w1130:u16, "Mods.Double Click"=w1127:bool)  [unwired: 1 in, 5 out]
        n729 = Equal?(x=u16 1, y=w1130) -> (x = y?=w1128:bool)
        n730 = And(x=w1128, y=w1127) -> (x .and. y?=w1126:bool)
        n731 = disable-structure shown="Disabled" {
          disable-tunnel: w1126 -> [w1133 _]
          disable-tunnel: w1125 -> [w1132 _]
          disable-tunnel: "Mode Buttons" -> [w1131 _]
          frame Disabled {
            n732 = case shown="True" w1133 {
              tunnel: w1131 -> [_ w1135]
              tunnel: w1132 -> [_ w1134]
              frame False {
              }
              frame True {
                n733 = case shown="\"Erase range\"" w1135 {
                  tunnel: w1134 -> [_ w1136]
                  frame "No Selection", Default {
                  }
                  frame "Erase range" {
                    n734 = property class="XYGraph (strict)"(reference=w1136, "ActPaletteTool"=0 ("Palette:Active Tool"), "Active Cursor"=u32 0, "Cursor.Visible"=TRUE) -> ()  [unwired: 1 in, 2 out]
                  }
                }
              }
            }
          }
          frame Enabled {
          }
        }
        n735 = event-data() -> ()  [unwired: 5 in, 1 out]
      }
      event "R-Plot 0", "R-Plot 1", "R-Plot 2", "R-Plot 3", "R-Plot 4", "R-Plot 5", "R-Plot 6", "R-Plot 7", "R-Plot 8", "R-Plot 9": Mouse Down {
        # "Process (double) click on plots in special modes (\"Cursor\", \"Erase\")"
        n736 = event-data() -> ("CtlRef"=w1143:refnum<vi>, "Coords"=w1146:T72, "Button"=w1142:u16, "Mods.Double Click"=w1145:bool, "PlatMods"=w1141:T73)  [unwired: 1 in, 3 out]
        n737 = property on="Mode Buttons" class="RadioBtnsControl (strict)"() -> ("Value"=w1144:T7)  [unwired: 2 in, 2 out]
        n738 = case shown="1" w1142 {
          tunnel: w1146 -> [_ _ w1151]
          tunnel: w1145 -> [_ _ w1150]
          tunnel: w1144 -> [_ _ w1149]
          tunnel: w1143 -> [_ _ w1148]
          tunnel: w1141 -> [_ _ _]
          frame 2 {
          }
          frame Default {
          }
          frame 1 {
            n739 = case shown="\"Cursor mode\"" w1149 {
              tunnel: w1148 -> [_ w1154 w1175 w1183]
              tunnel: w1151 -> [_ w1153 w1174 w1185]
              tunnel: w1150 -> [_ w1152 w1176 w1184]
              frame "No Selection", Default {
              }
              frame "Cursor mode" {
                n740 = case shown="True" w1152 {
                  tunnel: w1154 -> [_ w1164]
                  tunnel: w1153 -> [_ w1162]
                  frame False {
                  }
                  frame True {
                    n741 = invoke class="XYGraph (strict)" method="Map Coords To XY"(reference=w1164, "Coords"=w1162) -> (reference out=w1163:refnum<vi>, "XY"=w1161:cluster{"X":dbl, "Y":dbl})  [unwired: 5 in, 5 out]
                    n742 = Unbundle By Name(w1161) -> ("X"=w1159:dbl)
                    n743 = local read "Data Array"() -> (w1160:T28)
                    n744 = property class="XYGraph (strict)"(reference=w1163, "Active Cursor"=u32 0, "Cursor.Cursor Position"=w1161) -> ()  [unwired: 1 in, 2 out]
                    n745 = for {
                      tunnel: w1160 -> [w1173] mode=indexing
                      tunnel: w1159 -> [w1171]
                      tunnel: [w1167] -> w1158 mode=indexing
                      tunnel: [w1166] -> w1157 mode=indexing
                      n746 = Unbundle By Name(w1173) -> ("R"=w1170:dbl[], "T"=w1169:dbl[], "Time"=w1172:dbl[])
                      n747 = Threshold 1D Array(2:w1171, 3:w1172) -> (0:w1168:dbl)  [unwired: 1 in]
                      n748 = Index Array(array=w1170, index=w1168) -> (element=w1167:dbl)
                      n749 = Index Array(array=w1169, index=w1168) -> (element=w1166:dbl)
                    }
                    n750 = Array To Cluster(array=w1157) -> (cluster=w1155:T64)
                    n751 = Array To Cluster(array=w1158) -> (cluster=w1156:T64)
                    n752 = property on="Time" class="DigNum (strict)"("Value"=w1159) -> ()  [unwired: 2 in, 2 out]
                    n753 = property on="Small R Cluster" class="Clust (strict)"("Value"=w1156) -> ()  [unwired: 2 in, 2 out]
                    n754 = property on="Small T Cluster" class="Clust (strict)"("Value"=w1155) -> ()  [unwired: 2 in, 2 out]
                  }
                }
              }
              frame "Erase range" {
                n755 = case shown="False" w1176 {
                  tunnel: w1175 -> [w1180 _]
                  tunnel: w1174 -> [w1179 _]
                  frame False {
                    n756 = invoke class="XYGraph (strict)" method="Map Coords To XY"(reference=w1180, "Coords"=w1179) -> (reference out=w1182:refnum<vi>, "XY"=w1177:cluster{"X":dbl, "Y":dbl})  [unwired: 5 in, 5 out]
                    n757 = property class="XYGraph (strict)"(reference=w1182, "Active Cursor"=u32 0, "Cursor.Cursor Position"=w1177, "Active Cursor"=u32 1, "Cursor.Cursor Position"=w1177) -> ()  [unwired: 1 in, 2 out]
                  }
                  frame True {
                  }
                }
              }
              frame "Erase point" {
                n758 = case shown="True" w1184 {
                  tunnel: w1183 -> [w1190 w1205]
                  tunnel: w1185 -> [w1189 _]
                  frame False {
                    n759 = invoke class="XYGraph (strict)" method="Map Coords To XY"(reference=w1190, "Coords"=w1189) -> (reference out=w1188:refnum<vi>, "XY"=w1187:cluster{"X":dbl, "Y":dbl})  [unwired: 5 in, 5 out]
                    n760 = property class="XYGraph (strict)"(reference=w1188, "Active Cursor"=u32 0, "Cursor.Cursor Position"=w1187) -> ()  [unwired: 1 in, 2 out]
                  }
                  frame True {
                    n761 = property class="XYGraph (strict)"(reference=w1205, "Active Cursor"=u32 0) -> ("Cursor.Cursor X"=w1193:dbl)  [unwired: 1 in, 2 out]
                    n762 = local read "Channels Panel"() -> (w1192:T8)
                    n763 = local read "Data Array"() -> (w1191:T28)
                    n764 = Index Array(array=w1191, index=w1192) -> (element=w1198:cluster{"R":dbl[], "T":dbl[], "Time":dbl[]})
                    n765 = Unbundle By Name(w1198) -> ("R"=w1194:dbl[], "T"=w1195:dbl[], "Time"=w1196:dbl[])
                    n766 = Threshold 1D Array(2:w1193, 3:w1196) -> (0:w1197:dbl)  [unwired: 1 in]
                    n767 = Delete From Array(array=w1194, index=w1197) -> (array with subset deleted=w1201:dbl[])  [unwired: 1 in, 1 out]
                    n768 = Delete From Array(array=w1195, index=w1197) -> (array with subset deleted=w1200:dbl[])  [unwired: 1 in, 1 out]
                    n769 = Delete From Array(array=w1196, index=w1197) -> (array with subset deleted=w1199:dbl[])  [unwired: 1 in, 1 out]
                    n770 = Bundle By Name(cluster=w1198, "R"=w1201, "T"=w1200, "Time"=w1199) -> (w1202:cluster{"R":dbl[], "T":dbl[], "Time":dbl[]})
                    n771 = Replace Array Subset(array=w1191, new element=w1202, index=w1192) -> (w1203:T28)
                    n772 = local write "Data Array"(w1203) -> ()
                  }
                }
              }
            }
            "_LMBDown" <- TRUE ("Mouse down")
          }
        }
      }
      event "R-Plot 0", "R-Plot 1", "R-Plot 2", "R-Plot 3", "R-Plot 4", "R-Plot 5", "R-Plot 6", "R-Plot 7", "R-Plot 8", "R-Plot 9": Mouse Move {
        # "Process mouse movement over plots in special modes (\"Cursor\", \"Erase\")"
        n773 = event-data() -> ("CtlRef"=w1208:refnum<vi>, "Coords"=w1209:T72)  [unwired: 1 in, 3 out]
        n774 = property on="Mode Buttons" class="RadioBtnsControl (strict)"() -> ("Value"=w1212:T7)  [unwired: 2 in, 2 out]
        n775 = local read "_LMBDown"() -> (w1213:bool)
        n776 = Equal?(x=w1212, y=Cursor_Controls."Erase range" ("Mode Buttons")) -> (x = y?=w1210:bool)
        n777 = And(x=w1213, y=w1210) -> (x .and. y?=w1211:bool)
        n778 = case shown="True" w1211 {
          tunnel: w1209 -> [_ w1215]
          tunnel: w1208 -> [_ w1214]
          frame False {
          }
          frame True {
            n779 = invoke class="XYGraph (strict)" method="Map Coords To XY"(reference=w1214, "Coords"=w1215) -> (reference out=w1218:refnum<vi>, "XY"=w1217:cluster{"X":dbl, "Y":dbl})  [unwired: 5 in, 5 out]
            n780 = property class="XYGraph (strict)"(reference=w1218, "Active Cursor"=u32 1, "Cursor.Cursor Position"=w1217) -> ()  [unwired: 1 in, 2 out]
          }
        }
      }
      event "R-Plot 0", "R-Plot 1", "R-Plot 2", "R-Plot 3", "R-Plot 4", "R-Plot 5", "R-Plot 6", "R-Plot 7", "R-Plot 8", "R-Plot 9": Mouse Up {
        n781 = event-data() -> ("CtlRef"=w1222:refnum<vi>, "Button"=w1220:u16)  [unwired: 1 in, 6 out]
        n782 = property on="Mode Buttons" class="RadioBtnsControl (strict)"() -> ("Value"=w1223:T7)  [unwired: 2 in, 2 out]
        n783 = property class="XYGraph (strict)"(reference=w1222) -> ("ActPaletteTool"=w1221:i32)  [unwired: 1 in, 2 out]
        n784 = case shown="1" w1220 {
          tunnel: w1223 -> [_ w1227]
          tunnel: w1222 -> [_ w1226]
          tunnel: w1221 -> [_ w1225]
          frame Default {
          }
          frame 1 {
            n785 = local read "_LMBDown"() -> (w1224:bool)
            n786 = case shown="0" w1225 {
              tunnel: w1227 -> [_ w1232]
              tunnel: w1226 -> [_ w1231]
              tunnel: w1224 -> [_ w1229]
              frame Default {
                n787 = property on="Mode Buttons" class="RadioBtnsControl (strict)"("Val(Sgnl)"=T56."No Selection" ("Value (Signaling)")) -> ()  [unwired: 2 in, 2 out]
              }
              frame 0 {
                n788 = Equal?(x=w1232, y=T56."Erase range") -> (x = y?=w1235:bool)
                n789 = And(x=w1229, y=w1235) -> (x .and. y?=w1234:bool)
                n790 = case shown="True" w1234 {
                  tunnel: w1231 -> [_ w1258]
                  frame False {
                  }
                  frame True {
                    n791 = local read "Channels Panel"() -> (w1257:T8)
                    n792 = property class="XYGraph (strict)"(reference=w1258, "Active Cursor"=u32 0, "Active Cursor"=u32 1) -> ("Cursor.Cursor X"=w1255:dbl, "Cursor.Cursor X"=w1236:dbl)  [unwired: 1 in, 2 out]
                    n793 = local read "Data Array"() -> (w1252:T28)
                    n794 = Max & Min(x=w1255, y=w1236) -> (max(x,y)=w1245:dbl, min(x,y)=w1238:dbl)
                    n795 = Index Array(array=w1252, index=w1257) -> (element=w1248:cluster{"R":dbl[], "T":dbl[], "Time":dbl[]})
                    n796 = Unbundle By Name(w1248) -> ("R"=w1246:dbl[], "T"=w1247:dbl[], "Time"=w1244:dbl[])
                    n797 = Threshold 1D Array(2:w1245, 3:w1244) -> (0:w1242:dbl)  [unwired: 1 in]
                    n798 = Threshold 1D Array(2:w1238, 3:w1244) -> (0:w1243:dbl)  [unwired: 1 in]
                    n799 = Subtract(x=w1242, y=w1243) -> (x-y=w1241:dbl)
                    n800 = Delete From Array(array=w1246, length=w1241, index=w1243) -> (array with subset deleted=w1251:dbl[])  [unwired: 1 out]
                    n801 = Delete From Array(array=w1247, length=w1241, index=w1243) -> (array with subset deleted=w1250:dbl[])  [unwired: 1 out]
                    n802 = Delete From Array(array=w1244, length=w1241, index=w1243) -> (array with subset deleted=w1249:dbl[])  [unwired: 1 out]
                    n803 = Bundle By Name(cluster=w1248, "R"=w1251, "T"=w1250, "Time"=w1249) -> (w1253:cluster{"R":dbl[], "T":dbl[], "Time":dbl[]})
                    n804 = Replace Array Subset(array=w1252, new element=w1253, index=w1257) -> (w1254:T28)
                    n805 = local write "Data Array"(w1254) -> ()
                    n806 = property class="XYGraph (strict)"(reference=w1258, "Active Cursor"=u32 0, "Cursor.Cursor X"=w1238, "Active Cursor"=u32 1, "Cursor.Cursor X"=w1238) -> ()  [unwired: 1 in, 2 out]
                  }
                }
                n807 = local write "_LMBDown"(FALSE ("Mouse down")) -> ()
              }
            }
          }
        }
      }
      event "R-Plot 0", "R-Plot 1", "R-Plot 2", "R-Plot 3", "R-Plot 4", "R-Plot 5", "R-Plot 6", "R-Plot 7", "R-Plot 8", "R-Plot 9": Mouse Leave {
        n808 = event-data() -> ()  [unwired: 1 in, 4 out]
        n809 = local write "_LMBDown"(FALSE ("Mouse down")) -> ()
      }
      event "R-Plot 0", "R-Plot 1", "R-Plot 2", "R-Plot 3", "R-Plot 4", "R-Plot 5", "R-Plot 6", "R-Plot 7", "R-Plot 8", "R-Plot 9": Scale Range Change {
        w1263 = u8 0 ("X Scale.Scale Fit")
        # "Disable plot autoscaling if the user has changed the scale of the plot manualy"
        n810 = event-data() -> ("CtlRef"=w1262:refnum<vi>)  [unwired: 1 in, 7 out]
        n811 = property class="XYGraph (strict)"(reference=w1262, "XScale.ScaleFit"=w1263, "YScale.ScaleFit"=w1263) -> ()  [unwired: 1 in, 2 out]
      }
      event "R-Plot 0", "R-Plot 1", "R-Plot 2", "R-Plot 3", "R-Plot 4", "R-Plot 5", "R-Plot 6", "R-Plot 7", "R-Plot 8", "R-Plot 9": Shortcut Menu Activation? {
        w1272 = string[] ["Log Y"] ("item names")
        w1274 = string[] ["Zoom In to Last Data", "Autoscale XY"] ("item names")
        # "Add extra options to the plots context menu"
        n812 = event-data() -> ("MenuRef"=w1276:refnum<k9>, "CtlRef"=w1268:refnum<vi>)  [unwired: 1 in]
        n813 = Insert Menu Items(4:10, 7:w1274, 8:w1274, 9:w1276) -> (3:w1270:refnum<k9>)  [unwired: 2 in, 2 out]
        n814 = property class="XYGraph (strict)"(reference=w1268) -> ("YScale.Mapping Mode"=w1267:u8)  [unwired: 1 in, 2 out]
        n815 = Insert Menu Items(4:14, 7:w1272, 8:w1272, 9:w1270) -> (3:w1269:refnum<k9>)  [unwired: 2 in, 2 out]
        n816 = Not Equal To 0?(x=w1267) -> (x != 0?=w1266:bool)
        n817 = Set Menu Item Info(6:w1266, 7:"Log Y", 11:w1269) -> ()  [unwired: 4 in, 2 out]
        n818 = local read "_LMBDown"() -> (w1273:bool)
        n819 = event-data("Discard?"=w1273) -> ()  [unwired: 1 in, 1 out]
      }
      event "R-Plot 0", "R-Plot 1", "R-Plot 2", "R-Plot 3", "R-Plot 4", "R-Plot 5", "R-Plot 6", "R-Plot 7", "R-Plot 8", "R-Plot 9": Shortcut Menu Selection (User) {
        # "Zoom in to last \"Miniplot points\". Zoom out a bit to have some space around the points"
        n820 = event-data() -> ("CtlRef"=w1282:refnum<vi>, "ItemTag"=w1280:string)  [unwired: 1 in]
        n821 = Type Cast(type=refnum<vi> refnum ("R-Plot 0"), x=w1282) -> (*(type *) &x=w1281:refnum<vi>)
        n822 = property on="Runtime Settings" class="Clust (strict)"() -> ("Value"=w1278:T27)  [unwired: 2 in, 2 out]
        n823 = case shown="\"Zoom In to Last Data\"" w1280 {
          tunnel: w1281 -> [_ w1284 w1313 w1319]
          tunnel: w1278 -> [_ _ w1285 _]
          frame Default {
          }
          frame "Autoscale XY" {
            w1283 = u8 2 ("X Scale.Scale Fit")
            n824 = property class="XYGraph (strict)"(reference=w1284, "XScale.ScaleFit"=w1283, "YScale.ScaleFit"=w1283) -> ()  [unwired: 1 in, 2 out]
          }
          frame "Zoom In to Last Data" {
            w1309 = u8 0 ("Y Scale.Scale Fit")
            n825 = property class="XYGraph (strict)"(reference=w1313) -> (reference out=w1310:refnum<vi>, "Value"=w1312:cluster{dbl[], dbl[]})  [unwired: 1 in, 1 out]
            n826 = Unbundle By Name(w1285) -> ("Miniplot Time"=w1308:dbl)
            n827 = Unbundle(w1312) -> (w1287:dbl[], w1311:dbl[])
            n828 = Multiply(x=w1308, y=60.0) -> (x*y=w1304:dbl)
            n829 = Reverse 1D Array(array=w1287) -> (reversed array=w1292:dbl[])
            n830 = Reverse 1D Array(array=w1311) -> (reversed array=w1300:dbl[])
            n831 = Index Array(array=w1292) -> (element=w1306:dbl)  [unwired: 1 in]
            n832 = Multiply(x=0.5, y=w1304) -> (x*y=w1305:dbl)
            n833 = Add(x=w1305, y=w1306) -> (x+y=w1303:dbl)
            n834 = Subtract(x=w1306, y=w1304) -> (x-y=w1301:dbl)
            n835 = call "Improved Threshold Detector.71.vi"("Threshold"=w1301, "Array"=w1287) -> ("Positive transition indices"=w1288:i32[])  [unwired: 8 in, 1 out]
            n836 = Index Array(array=w1288) -> (element=w1314:i32)  [unwired: 1 in]
            n837 = Array Size(array=w1287) -> (size(s)=w1290:i32)
            n838 = Index Array(array=w1287, index=w1314) -> (element=w1286:dbl)
            n839 = Subtract(x=w1290, y=w1314) -> (x-y=w1289:i32)
            n840 = Array Subset(array=w1300, length=w1289) -> (w1299:dbl[])  [unwired: 1 in]
            n841 = Array Max & Min(array=w1299) -> (max value=w1296:dbl, min value=w1295:dbl)  [unwired: 2 out]
            n842 = Subtract(x=w1296, y=w1295) -> (x-y=w1298:dbl)
            n843 = Divide(x=w1298, y=2.0) -> (x/y=w1294:dbl)
            n844 = Add(x=w1296, y=w1294) -> (x+y=w1291:dbl)
            n845 = Subtract(x=w1295, y=w1294) -> (x-y=w1293:dbl)
            n846 = property class="XYGraph (strict)"(reference=w1310, "XScale.ScaleFit"=w1309, "YScale.ScaleFit"=w1309, "XScale.Maximum"=w1303, "XScale.Minimum"=w1286, "YScale.Maximum"=w1291, "YScale.Minimum"=w1293) -> ()  [unwired: 1 in, 2 out]
          }
          frame "Log Y" {
            n847 = property class="XYGraph (strict)"(reference=w1319) -> (reference out=w1318:refnum<vi>, "YScale.Mapping Mode"=w1317:u8)  [unwired: 1 in, 1 out]
            n848 = Equal To 0?(x=w1317) -> (x = 0?=w1316:bool)
            n849 = Boolean To (0,1)(Boolean=w1316) -> (0, 1=w1315:i16)
            n850 = property class="XYGraph (strict)"(reference=w1318, "YScale.Mapping Mode"=w1315) -> ()  [unwired: 1 in, 2 out]
          }
        }
      }
      event "uPlots.uPlot 0", "uPlots.uPlot 1", "uPlots.uPlot 2", "uPlots.uPlot 3", "uPlots.uPlot 4", "uPlots.uPlot 5", "uPlots.uPlot 6", "uPlots.uPlot 7", "uPlots.uPlot 8", "uPlots.uPlot 9": Mouse Down {
        # "Switch to big plot on double click on small plot"
        n851 = event-data() -> ("Mods.Double Click"=w1322:bool, "CtlRef"=w1321:refnum<vi>)  [unwired: 1 in]
        n852 = case shown="True" w1322 {
          tunnel: w1321 -> [_ w1325]
          frame False {
          }
          frame True {
            n853 = property class="XYGraph (strict)"(reference=w1325) -> ("Label.Text"=w1326:string)  [unwired: 1 in, 2 out]
            n854 = Reverse String(1:w1326) -> (0:w1327:string)
            n855 = Decimal String To Number(string=w1327, default (0L)=8 ("default (0 I32)")) -> (number=w1324:i32)  [unwired: 1 in, 1 out]
            n856 = property on="Channels Panel" class="TabCtl (strict)"("Val(Sgnl)"=w1324) -> ()  [unwired: 2 in, 2 out]
          }
        }
      }
      event "Erase all": Value Change {
        # "Clear data array.\nReset PID."
        n857 = event-data() -> ()  [unwired: 1 in, 6 out]
        n858 = local read "Channels Panel"() -> (w1331:T8)
        n859 = local read "Data Array"() -> (w1332:T28)
        n860 = Replace Array Subset(array=w1332, new element=cluster{"R":dbl[], "T":dbl[], "Time":dbl[]} {"R"=[], "T"=[], "Time"=[]} ("new element/subarray"), index=w1331) -> (w1330:T28)
        n861 = local write "Data Array"(w1330) -> ()
        n862 = disable-structure shown="Disabled" {
          frame Disabled {
            n863 = Initialize Array(cluster{"R":dbl[], "T":dbl[], "Time":dbl[]} {"R"=[], "T"=[], "Time"=[]}, 10 ("dimension size")) -> ()  [unwired: 1 out]
          }
          frame Enabled {
          }
        }
      }
      event "Clear all plots": Value Change {
        n864 = event-data() -> ()  [unwired: 1 in, 6 out]
        n865 = Initialize Array(cluster{"R":dbl[], "T":dbl[], "Time":dbl[]} {"R"=[], "T"=[], "Time"=[]}, 10 ("dimension size")) -> (w1337:cluster{"R":dbl[], "T":dbl[], "Time":dbl[]}[])
        n866 = local write "Data Array"(w1337) -> ()
      }
      event "Bridge settings.Bridge Type": Value Change {
        # "Select bridge type (AVS/zBridge). Show/hide corresponding controls."
        n867 = event-data() -> ("NewVal"=w1341:T61)  [unwired: 1 in, 5 out]
        n868 = flat-sequence {
          tunnel: w1341 -> [w1350]
          frame #0 {
            w1348 = u8 0 ("Disabled")
            w1349 = u8 0 ("Disabled")
            w1344 = FALSE ("Visible")
            w1343 = u8 2 ("Disabled")
            n869 = property on="Sync to ADC" class="Enum (strict)"("Visible"=w1344, "DisabledEnum"=w1343) -> ()  [unwired: 2 in, 2 out]
            n870 = property on="AVS RS232 Port" class="VISAName"("Visible"=w1344, "Disabled"=w1343) -> ()  [unwired: 2 in, 2 out]
            n871 = property on="zBridge settings" class="Bool"("Visible"=w1344, "Disabled"=w1343) -> ()  [unwired: 2 in, 2 out]
            n872 = property on="Picobus Delay" class="DigNum (strict)"("Visible"=w1344, "DisabledEnum"=w1343) -> ()  [unwired: 2 in, 2 out]
            n873 = property on="AVS GPIB Address" class="VISAName"("Visible"=w1344, "Disabled"=w1343) -> ()  [unwired: 2 in, 2 out]
            n874 = property on="Lower Panel" class="TabCtl (strict)"("Disabled"=w1348) -> ()  [unwired: 2 in, 2 out]
            n875 = property on="Read AVS channels from" class="DigNum (strict)"("Disabled"=w1349) -> ()  [unwired: 2 in, 2 out]
            n876 = property on="Last Channel" class="DigNum (strict)"("Disabled"=w1349) -> ()  [unwired: 2 in, 2 out]
            n877 = property on="Stabilisation Delay" class="DigNum (strict)"("Disabled"=w1349) -> ()  [unwired: 2 in, 2 out]
            n878 = property on="Averages" class="DigNum (strict)"("Disabled"=w1349) -> ()  [unwired: 2 in, 2 out]
            n879 = property on="Delay Between Scans" class="DigNum (strict)"("Disabled"=w1349) -> ()  [unwired: 2 in, 2 out]
            n880 = property on="Main Panel" class="TabCtl (strict)"("Disabled"=w1348) -> ()  [unwired: 2 in, 2 out]
            n881 = call "Channel Data - Build Ranges List.vi"("Values"="-1\r\n0\r\n1\r\n2\r\n3\r\n4\r\n5\r\n6\r\n7", "Strings"="n.a.\r\nopen\r\n2 Ohm\r\n20 Ohm\r\n200 Ohm\r\n2k Ohm\r\n20k Ohm\r\n200k Ohm\r\n2M Ohm") -> ("Strings and Values"=w1347:cluster{"String":string, "Value":i32}[])  [unwired: 4 in]
            n882 = property on="Range 0" class="Ring (strict)"("StringsAndValues[]"=w1347) -> ()  [unwired: 2 in, 2 out]
            n883 = property on="Range 1" class="Ring (strict)"("StringsAndValues[]"=w1347) -> ()  [unwired: 2 in, 2 out]
            n884 = property on="Range 2" class="Ring (strict)"("StringsAndValues[]"=w1347) -> ()  [unwired: 2 in, 2 out]
            n885 = property on="Range 3" class="Ring (strict)"("StringsAndValues[]"=w1347) -> ()  [unwired: 2 in, 2 out]
            n886 = property on="Range 4" class="Ring (strict)"("StringsAndValues[]"=w1347) -> ()  [unwired: 2 in, 2 out]
            n887 = property on="Range 5" class="Ring (strict)"("StringsAndValues[]"=w1347) -> ()  [unwired: 2 in, 2 out]
            n888 = property on="Range 6" class="Ring (strict)"("StringsAndValues[]"=w1347) -> ()  [unwired: 2 in, 2 out]
            n889 = property on="Range 7" class="Ring (strict)"("StringsAndValues[]"=w1347) -> ()  [unwired: 2 in, 2 out]
          }
          frame #1 {
            n890 = case shown="\"AVS47B (RS232 interface)\"" w1350 {
              frame "AVS47A (GPIB interface)" {
                n891 = local write "AVS Scan Parameters"(enum32{"Page 1", "Page 2"}."Page 1" ("Scan Parameters")) -> ()
                n892 = property on="AVS GPIB Address" class="VISAName"("Visible"=TRUE, "Disabled"=u8 0) -> ()  [unwired: 2 in, 2 out]
              }
              frame "AVS47B (RS232 interface)" {
                w1356 = u8 2 ("Disabled")
                w1355 = TRUE ("Visible")
                w1354 = u8 0 ("Disabled")
                n893 = property on="AVS RS232 Port" class="VISAName"("Visible"=w1355, "Disabled"=w1354) -> ()  [unwired: 2 in, 2 out]
                n894 = property on="Sync to ADC" class="Enum (strict)"("Visible"=w1355, "DisabledEnum"=w1354) -> ()  [unwired: 2 in, 2 out]
                n895 = property on="Picobus Delay" class="DigNum (strict)"("Visible"=w1355, "DisabledEnum"=w1354) -> ()  [unwired: 2 in, 2 out]
                n896 = property on="Read AVS channels from" class="DigNum (strict)"("Disabled"=w1356) -> ()  [unwired: 2 in, 2 out]
                n897 = property on="Last Channel" class="DigNum (strict)"("Disabled"=w1356) -> ()  [unwired: 2 in, 2 out]
                n898 = local write "AVS Scan Parameters"(enum32{"Page 1", "Page 2"}."Page 1" ("Scan Parameters")) -> ()
              }
              frame "AVS48SI (RS232 interface)" {
                w1361 = u8 2 ("Disabled")
                n899 = property on="Read AVS channels from" class="DigNum (strict)"("Disabled"=w1361) -> ()  [unwired: 2 in, 2 out]
                n900 = property on="Last Channel" class="DigNum (strict)"("Disabled"=w1361) -> ()  [unwired: 2 in, 2 out]
                n901 = property on="AVS RS232 Port" class="VISAName"("Visible"=TRUE, "Disabled"=u8 0) -> ()  [unwired: 2 in, 2 out]
                n902 = local write "AVS Scan Parameters"(enum32{"Page 1", "Page 2"}."Page 1" ("Scan Parameters")) -> ()
                n903 = call "Channel Data - Build Ranges List.vi"("Values"="-1\r\n0\r\n1\r\n2\r\n3\r\n4\r\n5\r\n6\r\n7", "Strings"="n.a.\r\n3 Ohm\r\n30 Ohm\r\n300 Ohm\r\n3k Ohm\r\n30k Ohm\r\n300k Ohm\r\n3M Ohm\r\n30m Ohm") -> ("Strings and Values"=w1359:cluster{"String":string, "Value":i32}[])  [unwired: 4 in]
                n904 = property on="Range 0" class="Ring (strict)"("StringsAndValues[]"=w1359) -> ()  [unwired: 2 in, 2 out]
                n905 = property on="Range 1" class="Ring (strict)"("StringsAndValues[]"=w1359) -> ()  [unwired: 2 in, 2 out]
                n906 = property on="Range 2" class="Ring (strict)"("StringsAndValues[]"=w1359) -> ()  [unwired: 2 in, 2 out]
                n907 = property on="Range 3" class="Ring (strict)"("StringsAndValues[]"=w1359) -> ()  [unwired: 2 in, 2 out]
                n908 = property on="Range 4" class="Ring (strict)"("StringsAndValues[]"=w1359) -> ()  [unwired: 2 in, 2 out]
                n909 = property on="Range 5" class="Ring (strict)"("StringsAndValues[]"=w1359) -> ()  [unwired: 2 in, 2 out]
                n910 = property on="Range 6" class="Ring (strict)"("StringsAndValues[]"=w1359) -> ()  [unwired: 2 in, 2 out]
                n911 = property on="Range 7" class="Ring (strict)"("StringsAndValues[]"=w1359) -> ()  [unwired: 2 in, 2 out]
              }
              frame "AVS Emulation" {
                n912 = local write "AVS Scan Parameters"(enum32{"Page 1", "Page 2"}."Page 1" ("Scan Parameters")) -> ()
              }
              frame "Impedance Bridge" {
                w1368 = u8 2 ("Disabled")
                n913 = local write "AVS Scan Parameters"(enum32{"Page 1", "Page 2"}."Page 2" ("Scan Parameters")) -> ()
                n914 = property on="zBridge settings" class="Bool"("Visible"=TRUE, "Disabled"=u8 0) -> ()  [unwired: 2 in, 2 out]
                n915 = property on="Read AVS channels from" class="DigNum (strict)"("Disabled"=w1368) -> ()  [unwired: 2 in, 2 out]
                n916 = property on="Last Channel" class="DigNum (strict)"("Disabled"=w1368) -> ()  [unwired: 2 in, 2 out]
                n917 = property on="Stabilisation Delay" class="DigNum (strict)"("Disabled"=w1368) -> ()  [unwired: 2 in, 2 out]
                n918 = property on="Averages" class="DigNum (strict)"("Disabled"=w1368) -> ()  [unwired: 2 in, 2 out]
                n919 = property on="Delay Between Scans" class="DigNum (strict)"("Disabled"=w1368) -> ()  [unwired: 2 in, 2 out]
              }
              frame "Disabled", Default {
                w1370 = u8 2 ("Disabled")
                n920 = property on="Lower Panel" class="TabCtl (strict)"("Disabled"=w1370) -> ()  [unwired: 2 in, 2 out]
                n921 = property on="Main Panel" class="TabCtl (strict)"("Disabled"=w1370) -> ()  [unwired: 2 in, 2 out]
              }
            }
          }
        }
      }
      event "Runtime Settings.Plot type": Value Change {
        # "Iterate through first 10 pages (plots only)"
        # "Switch between RxTime and TxTime plots"
        n922 = event-data() -> ("NewVal"=w1381:enum16{"R vs Time", "T vs Time"})  [unwired: 1 in, 5 out]
        n923 = Unbundle By Name(w1373) -> ("Reset PID loop"=w1372:refnum<user-event>)
        n924 = Equal To 0?(x=w1381) -> (x = 0?=w1380:bool)
        n925 = Select(t=u32 10532351, s=w1380, f=u32 16711680) -> (s? t:f=w1377:u32)
        n926 = property on="uPlots" class="Clust (strict)"() -> ("Controls[]"=w1375:refnum<vi>[])  [unwired: 2 in, 2 out]
        n927 = property on="Channels Panel" class="TabCtl (strict)"() -> ("Pages"=w1382:refnum<vi>[])  [unwired: 2 in, 2 out]
        n928 = for {
          N: 10 -> [_]
          tunnel: w1382 -> [w1392] mode=indexing
          tunnel: w1377 -> [w1385]
          tunnel: w1375 -> [w1383] mode=indexing
          # "!!NOTE:This routine assumes that graph is control #0 on page!!"
          n929 = property class="Page"(reference=w1392) -> ("ControlsOnPage"=w1390:refnum<vi>[])  [unwired: 1 in, 2 out]
          n930 = Type Cast(type=refnum<vi> refnum ("R-Plot 0"), x=w1383) -> (*(type *) &x=w1384:refnum<vi>)
          n931 = Index Array(array=w1390, index=0) -> (element=w1388:refnum<vi>)
          n932 = Type Cast(type=refnum<vi> refnum ("R-Plot 0"), x=w1388) -> (*(type *) &x=w1387:refnum<vi>)
          n933 = property class="XYGraph (strict)"(reference=w1387, "Plot.Plot Color"=w1385, "Plot.Fill/Pt. Color"=w1385) -> ()  [unwired: 1 in, 2 out]
          n934 = property class="XYGraph (strict)"(reference=w1384, "Plot.Plot Color"=w1385, "Plot.Fill/Pt. Color"=w1385) -> ()  [unwired: 1 in, 2 out]
        }
        n935 = Generate User Event(user event=w1372, event data cluster="" ("event data")) -> ()  [unwired: 2 in, 2 out]
      }
      event "Runtime Settings.Read AVS channels from", "Runtime Settings.Last Channel": Value Change {
        # "Change enabled channels for the AVS bridge"
        n936 = event-data() -> ()  [unwired: 1 in, 6 out]
        n937 = Unbundle By Name(w1395) -> ("UpdateChannelInfo"=w1394:refnum<user-event>)
        n938 = Generate User Event(user event=w1394, event data cluster=bool[] [] ("event data")) -> ()  [unwired: 2 in, 2 out]
      }
      event "Runtime Settings.Filter Graphs": Value Change {
        # "Graph filtering controls"
        n939 = event-data() -> ("NewVal"=w1398:bool)  [unwired: 1 in, 5 out]
        n940 = call "IsDisabled.vi"("Enabled?"=w1398) -> ("Numeric"=w1399:i16)
        n941 = property on="Y_min" class="DigNum (strict)"("Disabled"=w1399) -> ()  [unwired: 2 in, 2 out]
        n942 = property on="Y_max" class="DigNum (strict)"("Disabled"=w1399) -> ()  [unwired: 2 in, 2 out]
      }
      event "Channels Panel": Value Change {
        # "Show hide bottom Impedance/Temperature panel depending on the current tab page"
        n943 = event-data() -> ("NewVal"=w1402:T8)  [unwired: 1 in, 5 out]
        n944 = case shown="Default" w1402 {
          tunnel: [TRUE ("Visible") FALSE ("Visible")] -> w1401
          frame Default {
            n945 = property on="Mode Buttons" class="RadioBtnsControl (strict)"() -> ("Value"=w1404:T7)  [unwired: 2 in, 2 out]
            n946 = property on="Data History/RT Settings" class="TabCtl (strict)"("Value"=enum32{"History", "Settings"}."History" ("Data History")) -> ()  [unwired: 2 in, 2 out]
            n947 = property on="Mode Buttons" class="RadioBtnsControl (strict)"("Val(Sgnl)"=w1404) -> ()  [unwired: 2 in, 2 out]
          }
          frame "All", "PID loop" {
            n948 = property on="Data History/RT Settings" class="TabCtl (strict)"("Value"=enum32{"History", "Settings"}."Settings" ("Data History")) -> ()  [unwired: 2 in, 2 out]
          }
        }
        n949 = property on="Graph Controls Bar" class="TabCtl (strict)"("Visible"=w1401) -> ()  [unwired: 2 in, 2 out]
      }
      event Value Change {
        # "Calibration changed - update calibrations list"
        n950 = event-data() -> ()  [unwired: 1 in, 6 out]
        n951 = property on="Sensor Calibrations" class="Clust (strict)"() -> ("Controls[]"=w1411:refnum<vi>[])  [unwired: 2 in, 2 out]
        n952 = Array Size(array=w1411) -> (size(s)=w1412:i32)
        n953 = for {
          N: w1412 -> [_]
          tunnel: w1411 -> [w1416] mode=indexing
          tunnel: [w1413] -> w1410 mode=indexing
          w1415 = refnum<vi> refnum  # Ring
          n954 = Type Cast(type=w1415, x=w1416) -> (*(type *) &x=w1414:refnum<vi>)
          n955 = property class="Ring"(reference=w1414) -> ("RingText.Text"=w1413:string)  [unwired: 1 in, 2 out]
        }
        n956 = Array To Cluster(array=w1410) -> (cluster=→"_CurCalibrations":T33)
      }
      event "Data Logging Settings": Value Change {
        # "Log file settings changed. Generate new log file name"
        n957 = event-data() -> ()  [unwired: 1 in, 3 out]
        n958 = local read "Data Logging Settings"() -> (w1425:T37)
        n959 = Unbundle By Name(w1425) -> ("Run Description"=w1419:string, "Filenames Suffix"=w1420:string, "Log Files Folder"=w1426:path, "Log Files Name"=w1424:string, "Automode Files Name"=w1423:string)
        n960 = call <userlib>:"MGI Make String Filesafe.vi"("String In"=w1419) -> ("Filesafe String Out"=w1418:string)
        n961 = call "GeneratePaths.vi"("Filename Suffix"=w1420, "Run description"=w1418, "AVS_Path"=w1426, "AVS_FName"=w1424, "CAL_Path"=w1426, "CAL_FName"=w1423) -> ("Generated Log path"=w1422:path, "Generated Calib path"=w1421:path)  [unwired: 8 in]
        n962 = local write "_LogFilesPath"(w1422) -> ()
        n963 = local write "_CalibFilesPath"(w1421) -> ()
      }
      event "Convert R-T": Mouse Down; "QuickR": Value Change {
        # "Quick convert R->T"
        n964 = event-data() -> ()  [unwired: 1 in, 4 out]
        n965 = Unbundle By Name(w1427) -> ("Calibrations Folder"=w1428:path)
        n966 = property on="_QuickConvertCal" class="Ring (strict)"() -> ("Strings []"=w1431:string[], "Value"=w1432:u16)  [unwired: 2 in, 2 out]
        n967 = Index Array(array=w1431, index=w1432) -> (element=w1430:string)
        n968 = call "SelectSensor-txt no ext.vi"("Path"=w1428, "Resistance"="QuickR", "Select sensor"=w1430) -> ("error out"=w1429:errorcluster, "Temperature"=→"T7":dbl)
      }
      event "T Sweep.Current": Value Change {
        # "Current/ Setpoint value is changed"
        n969 = event-data() -> ("NewVal"=→"_I3SetPnt":dbl)  [unwired: 1 in, 5 out]
        n970 = Unbundle By Name(w1437) -> ("Reset PID loop"=w1436:refnum<user-event>)
        n971 = Generate User Event(user event=w1436, event data cluster="" ("event data")) -> ()  [unwired: 2 in, 2 out]
      }
      event Value Change {
        w1441 = FALSE ("Value (Signaling)")
        # "Changed Channel1 automatic mode"
        n972 = event-data() -> ("NewVal"=w1443:T39)  [unwired: 1 in, 5 out]
        n973 = Unbundle By Name(w1445) -> ("TempStabilized"=w1444:refnum<user-event>)
        n974 = property on="CS.Mode1.Start" class="Bool (strict)"("Val(Sgnl)"=w1441) -> ()  [unwired: 2 in, 2 out]
        n975 = property on="CS.Mode2.Start" class="Bool (strict)"("Val(Sgnl)"=w1441) -> ()  [unwired: 2 in, 2 out]
        n976 = case shown="\"Mode 1\"" w1443 {
          tunnel: [FALSE ("Automatic mode ON") TRUE ("Automatic mode ON") TRUE ("Automatic mode ON")] -> w1446
          tunnel: w1444 -> [_ w1456 _]
          tunnel: [0 1 2] -> w1442
          frame "Manual" {
            # "Set manual mode currents \nequal to last automode \nvalues."
            n977 = local read "CS.Automode Current"() -> (w1449:T23[])
            n978 = Index Array(array=w1449) -> (element #1=w1453:T23, element #2=w1452:T23, element #3=w1451:T23, element #4=w1450:T23)  [unwired: 4 in]
            n979 = property on="I" class="DigNum (strict)"("Val(Sgnl)"=w1453) -> ()  [unwired: 2 in, 2 out]
            n980 = property on="I" class="DigNum (strict)"("Val(Sgnl)"=w1452) -> ()  [unwired: 2 in, 2 out]
            n981 = property on="I" class="DigNum (strict)"("Val(Sgnl)"=w1451) -> ()  [unwired: 2 in, 2 out]
            n982 = property on="I" class="DigNum (strict)"("Val(Sgnl)"=w1450) -> ()  [unwired: 2 in, 2 out]
          }
          frame "Mode 1" {
            # "Set automatic mode currents equal to last manual values."
            n983 = local read "CS.Current Value"() -> (w1459:dbl[])
            n984 = Multiply(x=1000.0, y=w1459) -> (x*y=w1457:dbl[])
            n985 = local write "CS.Automode Current"(w1457) -> ()
            n986 = Generate User Event(user event=w1456, event data cluster=FALSE ("event data")) -> ()  [unwired: 2 in, 2 out]
          }
          frame "Mode2" {
            # "Set automatic mode currents equal to last manual values."
            n987 = local read "CS.Current Value"() -> (w1464:dbl[])
            n988 = Multiply(x=1000.0, y=w1464) -> (x*y=w1462:dbl[])
            n989 = local write "CS.Automode Current"(w1462) -> ()
          }
        }
        "CS.Automode 1" <- w1446
        "CS.Automode 2" <- w1446
        "CS.Automode 3" <- w1446
        "CS.Automode 0" <- w1446
        n990 = property on="CS Modes Panel" class="TabCtl (strict)"("Value"=w1442) -> ()  [unwired: 2 in, 2 out]
      }
      event "Data Logging Settings.External VI Path": Value Change {
        # "Set path for the external VI to call on TempStabilised event"
        n991 = event-data() -> ("NewVal"=w1469:path)  [unwired: 1 in, 5 out]
        n992 = vi-ref "OnTempStabilizedRef.vi"() -> (w1470:refnum<vi>)
        n993 = Open VI Reference(type specifier VI Refnum (for type only)=w1470, vi path=w1469) -> (vi reference=w1468:refnum<vi>)  [unwired: 4 in, 1 out]
        n994 = local write "_ExtVIReference"(w1468) -> ()
      }
      event "CS Settings.CS type": Value Change {
        # "Set CS type"
        n995 = event-data() -> ("NewVal"=w1472:T58)  [unwired: 1 in, 5 out]
        n996 = flat-sequence {
          tunnel: w1472 -> [w1499]
          frame #0 {
            w1484 = u8 2 ("Disabled")
            w1479 = u8 0 ("Disabled")
            w1494 = TRUE ("Visible")
            n997 = control-ref of="CS Indicators Panel"() -> (w1480:refnum<vi>)
            n998 = control-ref of="I0"() -> (w1491:refnum<vi>)
            n999 = control-ref of="I1"() -> (w1483:refnum<vi>)
            n1000 = control-ref of="CS.I0"() -> (w1490:refnum<vi>)
            n1001 = control-ref of="CS.I1"() -> (w1482:refnum<vi>)
            n1002 = control-ref of="I2"() -> (w1478:refnum<vi>)
            n1003 = control-ref of="I3"() -> (w1477:refnum<vi>)
            n1004 = control-ref of="CS Mode"() -> (w1481:refnum<vi>)
            n1005 = control-ref of="QCS. I0 Mapping"() -> (w1489:refnum<vi>)
            n1006 = property class="TabCtl (strict)"(reference=w1480, "Disabled"=w1479) -> ()  [unwired: 1 in, 2 out]
            n1007 = property class="Clust (strict)"(reference=w1491, "Disabled"=w1479) -> ()  [unwired: 1 in, 2 out]
            n1008 = property class="Clust (strict)"(reference=w1483, "Disabled"=w1479) -> ()  [unwired: 1 in, 2 out]
            n1009 = property class="Clust (strict)"(reference=w1478, "Disabled"=w1479) -> ()  [unwired: 1 in, 2 out]
            n1010 = property class="Clust (strict)"(reference=w1477, "Disabled"=w1479) -> ()  [unwired: 1 in, 2 out]
            n1011 = property class="Clust (strict)"(reference=w1490, "Disabled"=w1479) -> ()  [unwired: 1 in, 2 out]
            n1012 = property class="Clust (strict)"(reference=w1482, "Disabled"=w1479) -> ()  [unwired: 1 in, 2 out]
            n1013 = property class="Enum (strict)"(reference=w1489, "Disabled"=w1479) -> ()  [unwired: 1 in, 2 out]
            n1014 = property class="Enum (strict)"(reference=w1481, "Disabled"=w1479) -> ()  [unwired: 1 in, 2 out]
            n1015 = property on="Side Panel" class="TabCtl (strict)"() -> ("Pages"=w1473:refnum<vi>[])  [unwired: 2 in, 2 out]
            n1016 = control-ref of="TCS RS232 Port"() -> (w1493:refnum<vi>)
            n1017 = Index Array(array=w1473, index=1) -> (element=w1474:refnum<vi>)
            n1018 = control-ref of="Toggle Gated"() -> (w1485:refnum<vi>)
            n1019 = control-ref of="Toggle Gated"() -> (w1486:refnum<vi>)
            n1020 = control-ref of="Toggle Gated"() -> (w1487:refnum<vi>)
            n1021 = control-ref of="Toggle Gated"() -> (w1488:refnum<vi>)
            n1022 = control-ref of="CS.QCS Device Nr"() -> (w1496:refnum<vi>)
            n1023 = control-ref of="CS.QCS I0 Output"() -> (w1495:refnum<vi>)
            n1024 = property class="Page"(reference=w1474, "PageVis"=TRUE ("Page Visible")) -> ()  [unwired: 1 in, 2 out]
            n1025 = property class="Bool (strict)"(reference=w1485, "Disabled"=w1484) -> ()  [unwired: 1 in, 2 out]
            n1026 = property class="Bool (strict)"(reference=w1486, "Disabled"=w1484) -> ()  [unwired: 1 in, 2 out]
            n1027 = property class="Bool (strict)"(reference=w1487, "Disabled"=w1484) -> ()  [unwired: 1 in, 2 out]
            n1028 = property class="Bool (strict)"(reference=w1488, "Disabled"=w1484) -> ()  [unwired: 1 in, 2 out]
            n1029 = property class="DigNum (strict)"(reference=w1496, "Visible"=w1494) -> ()  [unwired: 1 in, 2 out]
            n1030 = property class="Enum (strict)"(reference=w1495, "Visible"=w1494) -> ()  [unwired: 1 in, 2 out]
            n1031 = property class="VISAName"(reference=w1493, "Visible"=FALSE) -> ()  [unwired: 1 in, 2 out]
          }
          frame #1 {
            n1032 = case shown="\"QCS v1\"" w1499 {
              tunnel: [refnum<class "TCS.lvclass"> refnum ("TCS.lvclass") refnum<class "QCS.lvclass"> refnum ("QCS.lvclass") w1519 w1533 refnum<class "PCS.lvclass"> refnum ("PCS.lvclass")] -> w1498
              tunnel: [w1500 w1518 u16 255 ("Value") u16 255 ("Value") w1538] -> w1497
              frame "TCS" {
                w1503 = u8 2 ("Disabled")
                w1516 = u8 0 ("Disabled")
                n1033 = control-ref of="TCS RS232 Port"() -> (w1506:refnum<vi>)
                n1034 = control-ref of="Toggle Gated"() -> (w1515:refnum<vi>)
                n1035 = control-ref of="Toggle Gated"() -> (w1514:refnum<vi>)
                n1036 = control-ref of="Toggle Gated"() -> (w1513:refnum<vi>)
                n1037 = control-ref of="Toggle Gated"() -> (w1512:refnum<vi>)
                n1038 = control-ref of="CS.QCS Device Nr"() -> (w1508:refnum<vi>)
                n1039 = control-ref of="I0"() -> (w1511:refnum<vi>)
                n1040 = control-ref of="CS.I0"() -> (w1504:refnum<vi>)
                n1041 = control-ref of="QCS. I0 Mapping"() -> (w1505:refnum<vi>)
                n1042 = property class="Bool (strict)"(reference=w1515, "Disabled"=w1516) -> ()  [unwired: 1 in, 2 out]
                n1043 = property class="Bool (strict)"(reference=w1514, "Disabled"=w1516) -> ()  [unwired: 1 in, 2 out]
                n1044 = property class="Bool (strict)"(reference=w1513, "Disabled"=w1516) -> ()  [unwired: 1 in, 2 out]
                n1045 = property class="Bool (strict)"(reference=w1512, "Disabled"=w1516) -> ()  [unwired: 1 in, 2 out]
                n1046 = property class="Clust (strict)"(reference=w1504, "Disabled"=w1503) -> ()  [unwired: 1 in, 2 out]
                n1047 = property class="Clust (strict)"(reference=w1511, "Disabled"=u8 2) -> ()  [unwired: 1 in, 2 out]
                n1048 = property class="DigNum (strict)"(reference=w1508, "Visible"=FALSE) -> ()  [unwired: 1 in, 2 out]
                n1049 = property class="VISAName"(reference=w1506, "Visible"=TRUE) -> ()  [unwired: 1 in, 2 out]
                n1050 = property class="Enum (strict)"(reference=w1505, "Disabled"=w1503) -> ()  [unwired: 1 in, 2 out]
                n1051 = property on="TCS RS232 Port" class="VISAName"() -> ("Value"=w1501:refnum<visa-resource-name>)  [unwired: 2 in, 2 out]
                n1052 = call "VISA to RS232 Port Nr.vi"("VISA Resource Name"=w1501) -> ("Port Number"=w1500:u8)  [unwired: 1 in]
              }
              frame "QCS v1" {
                n1053 = property on="CS.QCS Device Nr" class="DigNum (strict)"() -> ("Value"=w1518:u16)  [unwired: 2 in, 2 out]
              }
              frame "CS Emulation" {
                w1519 = refnum<class "CS Emulation.lvclass"> refnum  # CS Emulation.lvclass
                n1054 = control-ref of="CS.QCS Device Nr"() -> (w1522:refnum<vi>)
                n1055 = property class="DigNum (strict)"(reference=w1522, "Visible"=FALSE) -> ()  [unwired: 1 in, 2 out]
              }
              frame "Disabled", Default {
                w1523 = u8 2 ("Disabled")
                w1533 = refnum<class "CS Emulation.lvclass"> refnum  # CS Emulation.lvclass
                n1056 = control-ref of="CS Indicators Panel"() -> (w1532:refnum<vi>)
                n1057 = control-ref of="I0"() -> (w1527:refnum<vi>)
                n1058 = control-ref of="I1"() -> (w1526:refnum<vi>)
                n1059 = control-ref of="I2"() -> (w1525:refnum<vi>)
                n1060 = control-ref of="I3"() -> (w1524:refnum<vi>)
                n1061 = control-ref of="CS.QCS Device Nr"() -> (w1536:refnum<vi>)
                n1062 = property class="DigNum (strict)"(reference=w1536, "Visible"=FALSE) -> ()  [unwired: 1 in, 2 out]
                n1063 = property class="Clust (strict)"(reference=w1527, "Disabled"=w1523) -> ()  [unwired: 1 in, 2 out]
                n1064 = property class="Clust (strict)"(reference=w1526, "Disabled"=w1523) -> ()  [unwired: 1 in, 2 out]
                n1065 = property class="Clust (strict)"(reference=w1525, "Disabled"=w1523) -> ()  [unwired: 1 in, 2 out]
                n1066 = property class="Clust (strict)"(reference=w1524, "Disabled"=w1523) -> ()  [unwired: 1 in, 2 out]
                n1067 = property class="TabCtl (strict)"(reference=w1532, "Disabled"=w1523) -> ()  [unwired: 1 in, 2 out]
                n1068 = property on="Side Panel" class="TabCtl (strict)"() -> ("Pages"=w1531:refnum<vi>[])  [unwired: 2 in, 2 out]
                n1069 = Index Array(array=w1531, index=1) -> (element=w1530:refnum<vi>)
                n1070 = property class="Page"(reference=w1530, "PageVis"=FALSE ("Page Visible")) -> ()  [unwired: 1 in, 2 out]
              }
              frame "PCS (n.a.)" {
                w1539 = u8 2 ("Disabled")
                n1071 = control-ref of="I0"() -> (w1545:refnum<vi>)
                n1072 = control-ref of="I1"() -> (w1544:refnum<vi>)
                n1073 = control-ref of="CS.I0"() -> (w1543:refnum<vi>)
                n1074 = control-ref of="CS.I1"() -> (w1542:refnum<vi>)
                n1075 = control-ref of="CS Mode"() -> (w1541:refnum<vi>)
                n1076 = control-ref of="QCS. I0 Mapping"() -> (w1540:refnum<vi>)
                n1077 = property class="Clust (strict)"(reference=w1543, "Disabled"=w1539) -> ()  [unwired: 1 in, 2 out]
                n1078 = property class="Clust (strict)"(reference=w1542, "Disabled"=w1539) -> ()  [unwired: 1 in, 2 out]
                n1079 = property class="Clust (strict)"(reference=w1545, "Disabled"=w1539) -> ()  [unwired: 1 in, 2 out]
                n1080 = property class="Clust (strict)"(reference=w1544, "Disabled"=w1539) -> ()  [unwired: 1 in, 2 out]
                n1081 = property class="Enum (strict)"(reference=w1541, "Disabled"=w1539) -> ()  [unwired: 1 in, 2 out]
                n1082 = property class="Enum (strict)"(reference=w1540, "Disabled"=w1539) -> ()  [unwired: 1 in, 2 out]
                n1083 = property on="CS.QCS Device Nr" class="DigNum (strict)"() -> ("Value"=w1538:u16)  [unwired: 2 in, 2 out]
              }
            }
            "_CSClassRef" <- w1498
            n1084 = property on="_CS_Address" class="DigNum (strict)"("Value"=w1497) -> ()  [unwired: 2 in, 2 out]
          }
        }
      }
      event "CS Settings.CS.QCS Device Nr": Value Change {
        # "Set CS port"
        n1085 = event-data() -> ("NewVal"=w1547:u16)  [unwired: 1 in, 5 out]
        n1086 = property on="CS type" class="Enum (strict)"() -> ("Value"=w1548:T58)  [unwired: 2 in, 2 out]
        n1087 = case shown="\"QCS v1\"" w1548 {
          tunnel: w1547 -> [_ w1551 _]
          frame Default {
          }
          frame "QCS v1" {
            n1088 = Variant To Data(type=u32 255 ("HW Address"), Variant=w1551) -> (data=w1549:u32)  [unwired: 1 in, 1 out]
            n1089 = property on="_CS_Address" class="DigNum (strict)"("Value"=w1549) -> ()  [unwired: 2 in, 2 out]
          }
          frame "CS Emulation" {
            n1090 = property on="_CS_Address" class="DigNum (strict)"("Value"=u32 255 ("HW Address")) -> ()  [unwired: 2 in, 2 out]
          }
        }
      }
      event "CS Settings.TCS RS232 Port": Value Change {
        # "Set TCS port"
        n1091 = event-data() -> ("NewVal"=w1554:refnum<visa-resource-name>)  [unwired: 1 in, 5 out]
        n1092 = property on="CS type" class="Enum (strict)"() -> ("Value"=w1555:T58)  [unwired: 2 in, 2 out]
        n1093 = case shown="Default" w1555 {
          tunnel: w1554 -> [w1558 _]
          frame "TCS" {
            n1094 = Type Cast(type=refnum<visa-resource-name> refnum ("Value"), x=w1558) -> (*(type *) &x=w1557:refnum<visa-resource-name>)
            n1095 = call "VISA to RS232 Port Nr.vi"("VISA Resource Name"=w1557) -> ("Port Number"=w1559:u8)  [unwired: 1 in]
            n1096 = property on="_CS_Address" class="DigNum (strict)"("Value"=w1559) -> ()  [unwired: 2 in, 2 out]
          }
          frame Default {
          }
        }
      }
      event "Load Data": Value Change {
        # "copied from v4.57 2022-05-13"
        # "Load data from log files"
        n1097 = event-data() -> ()  [unwired: 1 in, 6 out]
        n1098 = property on="Log Files Folder" class="Path"() -> ("Value"=w1560:path)  [unwired: 2 in, 2 out]
        n1099 = disable-structure shown="Disabled" {
          frame Disabled {
            n1100 = call "FileDialog4.vi"() -> ()  [unwired: 12 in, 4 out]
          }
          frame Enabled {
          }
        }
        n1101 = call "File Dialog9"("start path"=w1560) -> ("selected paths"=w1562:path[], "cancelled"=w1561:bool)  [unwired: 11 in, 2 out]
        n1102 = case shown="False" w1561 {
          tunnel: w1562 -> [w1577 _]
          frame False {
            n1103 = property on="Bridge Type" class="Enum (strict)"() -> ("Value"=w1567:T61)  [unwired: 2 in, 2 out]
            n1104 = case shown="Default" w1567 {
              tunnel: [2 ("index")] -> w1566
              tunnel: [10 ("length")] -> w1564
              tunnel: [12 ("index")] -> w1565
              frame Default {
              }
            }
            n1105 = for {
              tunnel: w1577 -> [w1601] mode=indexing
              shift-right: [w1599] -> w1574
              shift-left: string[][] [] ("all rows") -> [w1600]
              # "skip header"
              n1106 = call <vilib>:"Read From Spreadsheet File (string).vi"("file path (dialog if empty)"=w1601) -> ("all rows"=w1597:string[][])  [unwired: 6 in, 4 out]
              n1107 = Array Subset(array=w1597, index (row)=5 ("index")) -> (w1596:string[][])  [unwired: 3 in]
              n1108 = Insert Into Array(array=w1600, new element=w1596) -> (w1599:string[][])  [unwired: 2 in]
            }
            n1109 = Index Array(array=w1574, index (col)=1 ("disabled index (col)")) -> (element=w1571:string[])  [unwired: 1 in]
            n1110 = Array Subset(array=w1574, index (col)=w1566, length (col)=w1564) -> (w1573:string[][])  [unwired: 2 in]
            n1111 = Array Subset(array=w1574, index (col)=w1565, length (col)=w1564) -> (w1572:string[][])  [unwired: 2 in]
            n1112 = Transpose 2D Array(2D array=w1573) -> (transposed array=w1569:string[][])
            n1113 = Transpose 2D Array(2D array=w1572) -> (transposed array=w1568:string[][])
            n1114 = for {
              tunnel: w1569 -> [w1593] mode=indexing
              tunnel: w1568 -> [w1592] mode=indexing
              tunnel: w1571 -> [w1594]
              tunnel: [w1591] -> w1570 mode=indexing
              # "Sort data by date and remove duplicate points"
              n1115 = Fract/Exp String To Number(string=w1593) -> (number=w1588:dbl[])  [unwired: 3 in, 1 out]
              n1116 = Fract/Exp String To Number(string=w1594) -> (number=w1590:dbl[])  [unwired: 3 in, 1 out]
              n1117 = Fract/Exp String To Number(string=w1592) -> (number=w1589:dbl[])  [unwired: 3 in, 1 out]
              n1118 = call <userlib>:"Sort 1D Array (DBL)__ogtk.vi"("Array in"=w1590) -> ("Sorted Pointers"=w1595:i32[], "Sorted Array out"=w1583:dbl[])  [unwired: 9 in]
              n1119 = call <userlib>:"Reorder 1D Array2 (DBL)__ogtk.vi"("indices"=w1595, "array"=w1588) -> ("reordered array"=w1587:dbl[])  [unwired: 9 in]
              n1120 = call <userlib>:"Reorder 1D Array2 (DBL)__ogtk.vi"("indices"=w1595, "array"=w1589) -> ("reordered array"=w1585:dbl[])  [unwired: 9 in]
              n1121 = call <userlib>:"Remove Duplicates from 1D Array (DBL)__ogtk.vi"("Input Array"=w1587) -> ("Output Array"=w1586:dbl[], "indices of removed elements"=w1581:i32[])
              n1122 = call <userlib>:"Delete Elements from 1D Array (DBL)__ogtk.vi"("indices"=w1581, "array"=w1585) -> ("array w/ subset deleted"=w1584:dbl[])  [unwired: 8 in, 1 out]
              n1123 = call <userlib>:"Delete Elements from 1D Array (DBL)__ogtk.vi"("indices"=w1581, "array"=w1583) -> ("array w/ subset deleted"=w1582:dbl[])  [unwired: 8 in, 1 out]
              n1124 = Bundle("Output Array"=w1586, "array w/ subset deleted"=w1584, "array w/ subset deleted"=w1582) -> (w1591:T74)  [unwired: 1 in]
            }
            n1125 = local write "Data Array"(w1570) -> ()
          }
          frame True {
          }
        }
      }
      event "Save Data 2": Value Change {
        # "Load data from log files"
        n1126 = event-data() -> ()  [unwired: 1 in, 6 out]
        n1127 = property on="Log Files Folder" class="Path"() -> ("Value"=w1607:path)  [unwired: 2 in, 2 out]
        n1128 = call "File Dialog"("start path"=w1607, "pattern (all files)"="*.dat", "pattern label"="Log files") -> ("selected path"=w1605:path, "cancelled"=w1606:bool)  [unwired: 9 in, 2 out]
        n1129 = case shown="False" w1606 {
          tunnel: w1605 -> [w1612 _]
          frame False {
            (unwired) 30 ("dimension size")
            n1130 = local read "Data Array"() -> (w1613:T28)
            n1131 = for {
              tunnel: w1613 -> [w1626] mode=indexing
              tunnel: [w1617] -> w1611 mode=indexing
              shift-right: [w1615] -> w1609
              shift-left: string[][] [] -> [w1616]
              n1132 = Unbundle By Name(w1626) -> ("Time"=w1623:dbl[], "R"=w1622:dbl[], "T"=w1618:dbl[])
              n1133 = property on="Data Logging Settings" class="Clust (strict)"() -> ("Value"=w1625:T37)  [unwired: 2 in, 2 out]
              n1134 = Unbundle By Name(w1625) -> ("Date Format"=w1624:string)
              n1135 = Array Size(array=w1618) -> (size(s)=w1617:i32)
              n1136 = for {
                tunnel: w1624 -> [w1629]
                tunnel: [w1628] -> w1621 mode=indexing
                tunnel: w1623 -> [w1627] mode=indexing
                n1137 = Format Date/Time String(time format string (%c)=w1629, seconds (now)=w1627) -> (date/time string=w1628:string)  [unwired: 1 in]
              }
              n1138 = Number To Fractional String(number=w1622) -> (F-format string=w1620:string[])  [unwired: 3 in]
              n1139 = Number To Fractional String(number=w1618) -> (F-format string=w1619:string[])  [unwired: 3 in]
              n1140 = Build Array(w1621, w1620, w1619) -> (w1614:string[][])
              n1141 = Build Array (concatenate)(w1616, w1614) -> (w1615:string[][])
            }
            n1142 = Array Max & Min(array=w1611) -> ()  [unwired: 4 out]
            n1143 = call "Write To Spreadsheet File (string) w Error.vi"("transpose? (no:F)"=TRUE, "2D data"=w1609, "file path (dialog if empty)"=w1612) -> ()  [unwired: 7 in, 2 out]
          }
          frame True {
          }
        }
      }
      event "Plot-save-screen": Value Change {
        n1144 = event-data() -> ()  [unwired: 1 in, 6 out]
        n1145 = property on="Log Files Folder" class="Path"() -> ("Value"=w1635:path)  [unwired: 2 in, 2 out]
        n1146 = call "File Dialog7"("start path"=w1635, "pattern (all files)"="*.dat", "pattern label"="Log files") -> ("selected path"=w1633:path, "cancelled"=w1634:bool)  [unwired: 9 in, 2 out]
        n1147 = case shown="False" w1634 {
          tunnel: w1633 -> [w1660 _]
          frame False {
            # "!!NOTE:This routine assumes that XY graph is \ncontrol #0 on tab page!!"
            n1148 = property on="Channels Panel" class="TabCtl (strict)"() -> ("Pages"=w1658:refnum<vi>[], "Value"=w1657:T8)  [unwired: 2 in, 2 out]
            n1149 = Index Array(array=w1658, index=w1657) -> (element=w1656:refnum<vi>)
            n1150 = property class="Page"(reference=w1656) -> ("ControlsOnPage"=w1653:refnum<vi>[])  [unwired: 1 in, 2 out]
            n1151 = Index Array(array=w1653, index=0) -> (element=w1655:refnum<vi>)
            n1152 = control-ref of="R-Plot 0"() -> (w1651:refnum<vi>)
            n1153 = Type Cast(type=w1651, x=w1655) -> (*(type *) &x=w1652:refnum<vi>)
            n1154 = property class="XYGraph (strict)"(reference=w1652) -> ("Value"=w1650:cluster{dbl[], dbl[]}, "XScale.Maximum"=w1649:dbl, "XScale.Minimum"=w1648:dbl)  [unwired: 1 in, 2 out]
            n1155 = Unbundle(w1650) -> (w1647:dbl[], w1646:dbl[])
            n1156 = call <userlib>:"MGI Threshold 1D Array Extended.vi"("Threshold Y"=w1649, "Y Value[]"=w1647) -> ("Extended Fractional Index"=w1637:dbl)  [unwired: 1 in]
            n1157 = call <userlib>:"MGI Threshold 1D Array Extended.vi"("Threshold Y"=w1648, "Y Value[]"=w1647) -> ("Extended Fractional Index"=w1636:dbl)  [unwired: 1 in]
            n1158 = Subtract(x=w1637, y=w1636) -> (x-y=w1659:dbl)
            n1159 = Array Subset(array=w1647, index=w1636, length=w1659) -> (w1641:dbl[])
            n1160 = Array Subset(array=w1646, index=w1636, length=w1659) -> (w1639:dbl[])
            n1161 = property on="Data Logging Settings" class="Clust (strict)"() -> ("Value"=w1643:T37)  [unwired: 2 in, 2 out]
            n1162 = Unbundle By Name(w1643) -> ("Date Format"=w1642:string)
            n1163 = Number To Fractional String(number=w1639) -> (F-format string=w1638:string[])  [unwired: 3 in]
            n1164 = for {
              tunnel: w1642 -> [w1663]
              tunnel: [w1662] -> w1640 mode=indexing
              tunnel: w1641 -> [w1661] mode=indexing
              n1165 = Format Date/Time String(time format string (%c)=w1663, seconds (now)=w1661) -> (date/time string=w1662:string)  [unwired: 1 in]
            }
            n1166 = Build Array(w1640, w1638) -> (w1645:string[][])
            n1167 = call <vilib>:"Write To Spreadsheet File (string).vi"("transpose? (no:F)"=TRUE, "2D data"=w1645, "file path (dialog if empty)"=w1660) -> ()  [unwired: 5 in, 1 out]
          }
          frame True {
          }
        }
      }
      event "Plot-Save All": Value Change {
        n1168 = event-data() -> ()  [unwired: 1 in, 6 out]
        n1169 = property on="Log Files Folder" class="Path"() -> ("Value"=w1669:path)  [unwired: 2 in, 2 out]
        n1170 = call "File Dialog8"("start path"=w1669, "pattern (all files)"="*.dat", "pattern label"="Log files") -> ("selected path"=w1667:path, "cancelled"=w1668:bool)  [unwired: 9 in, 2 out]
        n1171 = case shown="False" w1668 {
          tunnel: w1667 -> [w1687 _]
          frame False {
            # "!!NOTE:This routine assumes that XY graph is \ncontrol #0 on tab page!!"
            n1172 = property on="Channels Panel" class="TabCtl (strict)"() -> ("Pages"=w1686:refnum<vi>[], "Value"=w1685:T8)  [unwired: 2 in, 2 out]
            n1173 = Index Array(array=w1686, index=w1685) -> (element=w1684:refnum<vi>)
            n1174 = property class="Page"(reference=w1684) -> ("ControlsOnPage"=w1681:refnum<vi>[])  [unwired: 1 in, 2 out]
            n1175 = Index Array(array=w1681, index=0) -> (element=w1683:refnum<vi>)
            n1176 = control-ref of="R-Plot 0"() -> (w1679:refnum<vi>)
            n1177 = Type Cast(type=w1679, x=w1683) -> (*(type *) &x=w1680:refnum<vi>)
            n1178 = property class="XYGraph (strict)"(reference=w1680) -> ("Value"=w1678:cluster{dbl[], dbl[]})  [unwired: 1 in, 2 out]
            n1179 = Unbundle(w1678) -> (w1671:dbl[], w1670:dbl[])
            n1180 = property on="Data Logging Settings" class="Clust (strict)"() -> ("Value"=w1675:T37)  [unwired: 2 in, 2 out]
            n1181 = Unbundle By Name(w1675) -> ("Date Format"=w1674:string)
            n1182 = Number To Fractional String(number=w1670) -> (F-format string=w1672:string[])  [unwired: 3 in]
            n1183 = for {
              tunnel: w1674 -> [w1690]
              tunnel: [w1689] -> w1673 mode=indexing
              tunnel: w1671 -> [w1688] mode=indexing
              n1184 = Format Date/Time String(time format string (%c)=w1690, seconds (now)=w1688) -> (date/time string=w1689:string)  [unwired: 1 in]
            }
            n1185 = Build Array(w1673, w1672) -> (w1677:string[][])
            n1186 = call <vilib>:"Write To Spreadsheet File (string).vi"("transpose? (no:F)"=TRUE, "2D data"=w1677, "file path (dialog if empty)"=w1687) -> ()  [unwired: 5 in, 1 out]
          }
          frame True {
          }
        }
      }
      event "_CurrentsChanged": Value Change {
        # "New values for currents were entered by user/automode-> write new data to CS"
        n1187 = event-data() -> ()  [unwired: 1 in, 6 out]
        n1188 = local read "_CSClassRef"() -> (w1696:refnum<class "CS.lvclass">)
        n1189 = property on="CS status" class="Clust (strict)"() -> ("Value"=w1693:errorcluster)  [unwired: 2 in, 2 out]
        n1190 = call-dynamic "Read.vi"("CS in"=w1696, "error in (no error)"=w1693, "Optional"=TRUE ("Unused")) -> ("CS out"=w1695:refnum<class "CS.lvclass">, "error out"=w1692:errorcluster)  [unwired: 11 in, 4 out]
        n1191 = local write "_CSClassRef"(w1695) -> ()
        n1192 = property on="CS status" class="Clust (strict)"("Value"=w1692) -> ()  [unwired: 2 in, 2 out]
      }
      event "CS.QCS I0 Output": Value Change {
        # "Switch QCS channel 0 to aux output"
        n1193 = event-data() -> ("OldVal"=w1704:T38, "NewVal"=w1699:T38)  [unwired: 1 in, 4 out]
        n1194 = To Long Integer(number=w1699) -> (32bit integer=→"QCS. I0 Mapping":i32)
        n1195 = local read "_CSClassRef"() -> (w1702:refnum<class "CS.lvclass">)
        n1196 = property on="CS status" class="Clust (strict)"() -> ("Value"=w1703:errorcluster)  [unwired: 2 in, 2 out]
        n1197 = call-dynamic "Switch Output Channel.vi"("error in (no error)"=w1703, "New Channel"=w1699, "Old Channel"=w1704, "CS in"=w1702) -> ("error out"=w1700:errorcluster, "CS out"=w1701:refnum<class "CS.lvclass">)  [unwired: 6 in]
        n1198 = local write "_CSClassRef"(w1701) -> ()
        n1199 = property on="CS status" class="Clust (strict)"("Value"=w1700) -> ()  [unwired: 2 in, 2 out]
      }
      event "T Sweep.Start": Value Change {
        # "Setup and Start Current/Temperature sweep for CS channel 3"
        n1200 = event-data() -> ("CtlRef"=w1706:refnum<vi>, "NewVal"=w1707:bool)  [unwired: 1 in, 4 out]
        n1201 = case shown="False" w1707 {
          tunnel: w1706 -> [w1708 w1711]
          frame False {
            n1202 = property class="Bool (strict)"(reference=w1708, "Caption.Text"="Start") -> ()  [unwired: 1 in, 2 out]
          }
          frame True {
            n1203 = property on="Start value" class="DigNum (strict)"() -> ("Value"=w1712:dbl)  [unwired: 2 in, 2 out]
            n1204 = property class="Bool (strict)"(reference=w1711, "Caption.Text"="Stop") -> ()  [unwired: 1 in, 2 out]
            n1205 = property on="Current" class="DigNum (strict)"("Val(Sgnl)"=w1712) -> ()  [unwired: 2 in, 2 out]
          }
        }
      }
      event "T Sweep.I_next": Value Change {
        # "Go to next step in Current/Temperature sweep for CS channel 3"
        n1206 = event-data() -> ()  [unwired: 1 in, 6 out]
        n1207 = property on="I_next" class="Bool (strict)"("Value"=FALSE) -> ()  [unwired: 2 in, 2 out]
        n1208 = call "Current Time(double).vi"() -> ("Current Time (double)"=w1714:dbl)  [unwired: 6 in, 1 out]
        n1209 = local write "_TimeOld"(w1714) -> ()
        n1210 = property on="Current" class="DigNum (strict)"() -> ("Value"=w1715:dbl)  [unwired: 2 in, 2 out]
        n1211 = property on="Step" class="DigNum (strict)"() -> ("Value"=w1720:dbl)  [unwired: 2 in, 2 out]
        n1212 = Add(x=w1715, y=w1720) -> (x+y=w1719:dbl)
        n1213 = property on="End value" class="DigNum (strict)"() -> ("Value"=w1718:dbl)  [unwired: 2 in, 2 out]
        n1214 = property on="Start value" class="DigNum (strict)"() -> ("Value"=w1717:dbl)  [unwired: 2 in, 2 out]
        n1215 = In Range and Coerce(upper limit=w1718, x=w1719, lower limit=w1717) -> (coerced(x)=w1716:dbl)  [unwired: 1 out]
        n1216 = property on="Current" class="DigNum (strict)"("Val(Sgnl)"=w1716) -> ()  [unwired: 2 in, 2 out]
      }
      event "T Sweep.I_prev": Value Change {
        # "Go to previous step in Current/Temperature sweep for CS channel 3"
        n1217 = event-data() -> ()  [unwired: 1 in, 6 out]
        n1218 = call "Current Time(double).vi"() -> ("Current Time (double)"=w1723:dbl)  [unwired: 6 in, 1 out]
        n1219 = property on="I_prev" class="Bool (strict)"("Value"=FALSE) -> ()  [unwired: 2 in, 2 out]
        n1220 = local write "_TimeOld"(w1723) -> ()
        n1221 = property on="Current" class="DigNum (strict)"() -> ("Value"=w1725:dbl)  [unwired: 2 in, 2 out]
        n1222 = property on="Step" class="DigNum (strict)"() -> ("Value"=w1730:dbl)  [unwired: 2 in, 2 out]
        n1223 = Subtract(x=w1725, y=w1730) -> (x-y=w1729:dbl)
        n1224 = property on="End value" class="DigNum (strict)"() -> ("Value"=w1728:dbl)  [unwired: 2 in, 2 out]
        n1225 = property on="Start value" class="DigNum (strict)"() -> ("Value"=w1727:dbl)  [unwired: 2 in, 2 out]
        n1226 = In Range and Coerce(upper limit=w1728, x=w1729, lower limit=w1727) -> (coerced(x)=w1726:dbl)  [unwired: 1 out]
        n1227 = property on="Current" class="DigNum (strict)"("Val(Sgnl)"=w1726) -> ()  [unwired: 2 in, 2 out]
      }
      event User Event {
        # "Reset the PID loop"
        n1228 = event-data() -> ()  [unwired: 1 in, 5 out]
        n1229 = local write "CS.Mode1.PID Error"(0.0 ("T_error")) -> ()
      }
      event "Minimize UI 1", "Minimize UI 2": Value Change {
        (unwired) 29 ("Splitter Position")
        (unwired) 534 ("Numeric 2")
        # "Shrink/restore the program window"
        # "726"
        # "222"
        # "1243"
        # "816"
        n1230 = event-data() -> ()  [unwired: 1 in, 6 out]
        n1231 = case shown="False" "Minimize UI 1" {
          tunnel: "Minimize UI 2" -> [_ w1761]
          frame True {
            (unwired) T57."Disabled" ("Value")
            n1232 = property on="CS type" class="Enum (strict)"() -> ("Value"=w1747:T58)  [unwired: 2 in, 2 out]
            n1233 = property on="Bridge Type" class="Enum (strict)"() -> ("Value"=w1742:T61)  [unwired: 2 in, 2 out]
            n1234 = Equal?(x=w1742, y=T57."Disabled" ("Value")) -> (x = y?=w1740:bool)
            n1235 = Equal?(x=w1747, y=T58."Disabled" ("Value")) -> (x = y?=w1746:bool)
            n1236 = property on="Data History/RT Settings" class="TabCtl (strict)"("Value"=enum32{"History", "Settings"}."History" ("Data History")) -> ()  [unwired: 2 in, 2 out]
            n1237 = Exclusive Or(1:w1740, 2:w1746) -> (0:w1739:bool)
            n1238 = property on="Mode Buttons" class="RadioBtnsControl (strict)"("Disabled"=u8 2, "Val(Sgnl)"=T56."No Selection" ("Value (Signaling)")) -> ()  [unwired: 2 in, 2 out]
            n1239 = property class="VI"() -> ("Front Panel.PanelBounds"=w1749:T75)  [unwired: 2 in, 2 out]
            n1240 = Select(t=i16 105 ("y"), s=w1739, f=i16 169 ("y")) -> (s? t:f=w1743:i16)
            n1241 = Unbundle By Name(w1749) -> ("Left"=w1755:i16, "Top"=w1752:i16)
            n1242 = property on="Splitter 3" class="Splitter"("Position"=29 ("Splitter Position")) -> (error out=w1741:errorcluster)  [unwired: 2 in, 1 out]
            n1243 = Add(x=i16 806 ("right"), y=w1755) -> (x+y=w1754:i16)
            n1244 = Add(x=w1752, y=w1743) -> (x+y=w1751:i16)
            n1245 = Bundle By Name(cluster=w1749, "Right"=w1754, "Bottom"=w1751) -> (w1756:T75)
            n1246 = case shown="True" w1740 {
              tunnel: w1741 -> [_ w1759]
              frame False {
              }
              frame True {
                n1247 = property on="Splitter 4" class="Splitter"(error in=w1759, "Position"=32 ("Splitter Position")) -> ()  [unwired: 1 in, 2 out]
              }
            }
            n1248 = property class="VI"("Front Panel.PanelBounds"=w1756) -> ()  [unwired: 2 in, 2 out]
          }
          frame False {
            n1249 = property class="VI"() -> ("Front Panel.PanelBounds"=w1768:T75)  [unwired: 2 in, 2 out]
            n1250 = property on="Channels Panel" class="TabCtl (strict)"() -> ("Value"=w1776:T8)  [unwired: 2 in, 2 out]
            n1251 = Unbundle By Name(w1768) -> ("Left"=w1774:i16, "Top"=w1772:i16)
            n1252 = property on="Channels Panel" class="TabCtl (strict)"("Val(Sgnl)"=w1776) -> ()  [unwired: 2 in, 2 out]
            n1253 = Select(t=i16 806 ("right"), s=w1761, f=i16 1206 ("right")) -> (s? t:f=w1765:i16)
            n1254 = Add(x=w1765, y=w1774) -> (x+y=w1773:i16)
            n1255 = Add(x=w1772, y=i16 702) -> (x+y=w1770:i16)
            n1256 = Bundle By Name(cluster=w1768, "Right"=w1773, "Bottom"=w1770) -> (w1775:T75)
            n1257 = property on="Mode Buttons" class="RadioBtnsControl (strict)"("Disabled"=u8 0) -> ()  [unwired: 2 in, 2 out]
            n1258 = property class="VI"("Front Panel.PanelBounds"=w1775) -> (error out=w1762:errorcluster)  [unwired: 2 in, 1 out]
            n1259 = property on="Splitter 3" class="Splitter"(error in=w1762, "Position"=559 ("Splitter Position")) -> (error out=w1766:errorcluster)  [unwired: 1 in, 1 out]
            n1260 = property on="Splitter 4" class="Splitter"(error in=w1766, "Position"=635 ("Splitter Position")) -> ()  [unwired: 1 in, 2 out]
          }
        }
        n1261 = property on="Splitter 2" class="Splitter"("Position"=805 ("Splitter Position")) -> ()  [unwired: 2 in, 2 out]
      }
      event "Copy to Clipboard": Value Change {
        # "Copy current values to the clipboard"
        n1262 = event-data() -> ()  [unwired: 1 in, 6 out]
        n1263 = property on="_ScanData" class="Arr (strict)"() -> ("Value"=w1782:dbl[])  [unwired: 2 in, 2 out]
        n1264 = property on="T Array" class="Arr (strict)"() -> ("Value"=w1781:dbl[])  [unwired: 2 in, 2 out]
        n1265 = Build Array(w1782, w1781) -> (w1780:dbl[][])
        n1266 = Transpose 2D Array(2D array=w1780) -> (transposed array=w1779:dbl[][])
        n1267 = Array To Spreadsheet String(delimiter (Tab)="\t", array=w1779, 3:"%.4g" ("format string")) -> (spreadsheet string=w1785:string)
        n1268 = invoke class="App" method="Clipboard.Write"("Param 0"=w1785) -> ()  [unwired: 3 in, 4 out]
      }
      event "Show PID graph?": Value Change {
        # "Display plots with the PID parameters vs time for debugging"
        n1269 = event-data() -> ("NewVal"=w1787:bool)  [unwired: 1 in, 5 out]
        n1270 = property on="Channels Panel" class="TabCtl (strict)"() -> ("Pages"=w1790:refnum<vi>[])  [unwired: 2 in, 2 out]
        n1271 = Reverse 1D Array(array=w1790) -> (reversed array=w1789:refnum<vi>[])
        n1272 = Index Array(array=w1789) -> (element=w1788:refnum<vi>)  [unwired: 1 in]
        n1273 = property class="Page"(reference=w1788, "PageVis"=w1787) -> ()  [unwired: 1 in, 2 out]
      }
      event "I0.uA", "I1.uA", "I2.uA", "I3.uA": Mouse Up {
        # "Show curent edit filed on double clicking the current indicator. Set the field to the actual current value."
        n1274 = event-data() -> ("Mods.Double Click"=w1793:bool, "CtlRef"=w1792:refnum<vi>)  [unwired: 1 in, 5 out]
        n1275 = case shown="True" w1793 {
          tunnel: w1792 -> [_ w1804]
          frame False {
          }
          frame True {
            w1800 = TRUE ("Visible")
            n1276 = property class="Str"(reference=w1804) -> ("Owner"=w1803:refnum<vi>)  [unwired: 1 in, 2 out]
            n1277 = control-ref of="uA 0"() -> (w1810:refnum<vi>)
            n1278 = control-ref of="uA 1"() -> (w1813:refnum<vi>)
            n1279 = control-ref of="uA 2"() -> (w1812:refnum<vi>)
            n1280 = control-ref of="uA 3"() -> (w1811:refnum<vi>)
            n1281 = control-ref of="I0"() -> (w1801:refnum<vi>)
            n1282 = control-ref of="I1"() -> (w1807:refnum<vi>)
            n1283 = control-ref of="I2"() -> (w1806:refnum<vi>)
            n1284 = control-ref of="I3"() -> (w1799:refnum<vi>)
            n1285 = property on="CS.Current Value" class="Arr (strict)"() -> ("Value"=w1798:dbl[])  [unwired: 2 in, 2 out]
            n1286 = Type Cast(type=w1799, x=w1803) -> (*(type *) &x=w1802:refnum<vi>)
            n1287 = Build Array(w1810, w1813, w1812, w1811) -> (w1809:refnum<vi>[])
            n1288 = Build Array(w1801, w1807, w1806, w1799) -> (w1805:refnum<vi>[])
            n1289 = Search 1D Array(1D array=w1805, element=w1802) -> (index of element=w1797:i32)  [unwired: 1 in]
            n1290 = Index Array(array=w1798, index=w1797) -> (element=w1796:dbl)
            n1291 = Index Array(array=w1809, index=w1797) -> (element=w1808:refnum<vi>)
            n1292 = Multiply(x=1000.0, y=w1796) -> (x*y=w1795:dbl)
            n1293 = property on="Property Node" class="DigNum (strict)"(reference=w1808, "Value"=w1795, "Visible"=w1800, "Key Focus"=w1800) -> ()  [unwired: 1 in, 2 out]
          }
        }
      }
      event "I0.current flows", "I1.current flows", "I2.current flows", "I3.current flows": Mouse Up {
        # "Toggle the current channel by double clickin on the \"On\" led in the current indicator."
        n1294 = event-data() -> ("CtlRef"=w1815:refnum<vi>, "Mods.Double Click"=w1816:bool)  [unwired: 1 in, 5 out]
        n1295 = case shown="True" w1816 {
          tunnel: w1815 -> [_ w1825]
          frame False {
          }
          frame True {
            n1296 = control-ref of="current flows"() -> (w1830:refnum<vi>)
            n1297 = control-ref of="current flows"() -> (w1829:refnum<vi>)
            n1298 = control-ref of="current flows"() -> (w1828:refnum<vi>)
            n1299 = control-ref of="current flows"() -> (w1827:refnum<vi>)
            n1300 = control-ref of="Toggle ON/OFF"() -> (w1824:refnum<vi>)
            n1301 = control-ref of="Toggle ON/OFF"() -> (w1822:refnum<vi>)
            n1302 = control-ref of="Toggle ON/OFF"() -> (w1821:refnum<vi>)
            n1303 = control-ref of="Toggle ON/OFF"() -> (w1823:refnum<vi>)
            n1304 = Build Array(w1830, w1829, w1828, w1827) -> (w1826:refnum<vi>[])
            n1305 = Build Array(w1824, w1822, w1821, w1823) -> (w1820:refnum<vi>[])
            n1306 = Search 1D Array(1D array=w1826, element=w1825) -> (index of element=w1819:i32)  [unwired: 1 in]
            n1307 = Index Array(array=w1820, index=w1819) -> (element=w1818:refnum<vi>)
            n1308 = property class="Bool (strict)"(reference=w1818, "Val(Sgnl)"=TRUE ("Value (Signaling)")) -> ()  [unwired: 1 in, 2 out]
          }
        }
      }
      event "uA 0", "uA 1", "uA 2", "uA 3": Value Change {
        w1833 = refnum<vi> refnum  # Numeric
        w1837 = refnum<vi> refnum  # Enum
        # "User has entered the current by double clicking on the current indicators at the bottom. \nSet range to \"Auto\" and interpret the entered value as [uA]"
        # "!!NOTE:This routine assumes that Current and Range are controls #2 & #3 in current control cluster"
        n1309 = event-data() -> ("CtlRef"=w1845:refnum<vi>, "NewVal"=w1832:u32)  [unwired: 1 in, 4 out]
        n1310 = control-ref of="CS.I0"() -> (w1854:refnum<vi>)
        n1311 = control-ref of="CS.I1"() -> (w1852:refnum<vi>)
        n1312 = control-ref of="CS.I2"() -> (w1853:refnum<vi>)
        n1313 = control-ref of="CS.I3"() -> (w1855:refnum<vi>)
        n1314 = control-ref of="uA 0"() -> (w1847:refnum<vi>)
        n1315 = control-ref of="uA 1"() -> (w1850:refnum<vi>)
        n1316 = control-ref of="uA 2"() -> (w1849:refnum<vi>)
        n1317 = control-ref of="uA 3"() -> (w1848:refnum<vi>)
        n1318 = Build Array(w1854, w1852, w1853, w1855) -> (w1851:refnum<vi>[])
        n1319 = Build Array(w1847, w1850, w1849, w1848) -> (w1846:refnum<vi>[])
        n1320 = Search 1D Array(1D array=w1846, element=w1845) -> (index of element=w1844:i32)  [unwired: 1 in]
        n1321 = Index Array(array=w1851, index=w1844) -> (element=w1843:refnum<vi>)
        n1322 = property class="Clust (strict)"(reference=w1843) -> ("Controls[]"=w1842:refnum<vi>[])  [unwired: 1 in, 2 out]
        n1323 = Index Array(array=w1842, index #1=3 ("index"), index #2=2 ("index")) -> (element #1=w1839:refnum<vi>, element #2=w1835:refnum<vi>)
        n1324 = Type Cast(type=w1833, x=w1835) -> (*(type *) &x=w1834:refnum<vi>)
        n1325 = Type Cast(type=w1837, x=w1839) -> (*(type *) &x=w1838:refnum<vi>)
        n1326 = property on="Property Node" class="Num"(reference=w1834, "Value"=w1832) -> ()  [unwired: 1 in, 2 out]
        n1327 = property on="Property Node" class="Enum"(reference=w1838, "Value"=T55."Auto") -> ()  [unwired: 1 in, 2 out]
      }
      event "_AVSRanges": Value Change {
        # "If user has changed the exitation, update the AVS bridge settings."
        n1328 = event-data() -> ("NewVal"=w1858:T29)  [unwired: 1 in, 5 out]
        n1329 = property on="AVS Exc&Ranges" class="Clust (strict)"() -> ("Value"=w1857:T15)  [unwired: 2 in, 2 out]
        n1330 = call "Combine Excitation&Range.vi"("Ranges"=w1858, "Exc&Ranges In"=w1857) -> ("Exc&Ranges Out"=w1859:T76)
        n1331 = property on="AVS Exc&Ranges" class="Clust (strict)"("Value"=w1859) -> ()  [unwired: 2 in, 2 out]
      }
      event Panel Close? {
        # "Ask for confirmation is user is trying to close the program"
        n1332 = event-data() -> ()  [unwired: 1 in, 4 out]
        n1333 = Two Button Dialog(message="Are you sure you want to quit the program?") -> (T button?=w1862:bool)  [unwired: 2 in]
        n1334 = Not(x=w1862) -> (.not. x?=w1863:bool)
        n1335 = event-data("Discard?"=w1863) -> ()  [unwired: 1 in, 1 out]
      }
      event "Save config": Mouse Up {
        # "Save parameters to the configuration file"
        n1336 = event-data() -> ()  [unwired: 1 in, 8 out]
        n1337 = control-ref of="CS Cannel Names"() -> (w1875:refnum<vi>)
        n1338 = control-ref of="AVS names"() -> (w1874:refnum<vi>)
        n1339 = control-ref of="_CurCalibrations"() -> (w1869:refnum<vi>)
        n1340 = control-ref of="CS.Mode1.PID"() -> (w1867:refnum<vi>)
        n1341 = control-ref of="CS.Mode1.Settings"() -> (w1866:refnum<vi>)
        n1342 = control-ref of="zBridge.Active Channels"() -> (w1868:refnum<vi>)
        n1343 = control-ref of="Bridge settings"() -> (w1880:refnum<vi>)
        n1344 = control-ref of="Runtime Settings"() -> (w1881:refnum<vi>)
        n1345 = control-ref of="CS Settings"() -> (w1879:refnum<vi>)
        n1346 = control-ref of="Sensor Calibrations"() -> (w1882:refnum<vi>)
        n1347 = control-ref of="PID setup"() -> (w1883:refnum<vi>)
        n1348 = control-ref of="Data Logging Settings"() -> (w1878:refnum<vi>)
        n1349 = call "File Dialog3"("start path"=path "C:/LC Data/Configuration" ("Relative path (.)"), "pattern (all files)"="*.ini") -> ("selected path"=w1870:path)  [unwired: 10 in, 3 out]
        n1350 = Build Array(w1868, w1880, w1881, w1879, w1878, w1882, w1883, w1875, w1874, w1869, w1867, w1866) -> (w1876:refnum<vi>[])
        n1351 = call "Save Load Settings to File by Ref with path.vi"("Array of Cluster References"=w1876, "Action"=enum8{"Load", "Save"}."Save", "error in (no error)"=w1873, "Configuration file"=w1870) -> ("error out"=w1872:errorcluster)  [unwired: 5 in]
      }
      event "Load config": Mouse Up {
        # "Load parameters from the configuration file"
        n1352 = event-data() -> ()  [unwired: 1 in, 8 out]
        n1353 = Unbundle By Name(w1887) -> ("UpdateCalibrations"=w1886:refnum<user-event>)
        n1354 = flat-sequence {
          tunnel: [w1912] -> w1897
          tunnel: w1893 -> [w1907]
          tunnel: [w1899] -> w1888
          tunnel: w1884 -> [w1898]
          tunnel: w1897 -> [w1927]
          tunnel: [w1927] -> w1896
          tunnel: [w1925] -> w1889
          tunnel: w1888 -> [w1925]
          tunnel: [w1932] -> w1895
          tunnel: w1896 -> [w1931]
          tunnel: [w1929] -> w1890
          tunnel: w1889 -> [w1929]
          tunnel: w1895 -> [w1938]
          tunnel: [w1938] -> w1894
          tunnel: [w1936] -> w1891
          tunnel: w1890 -> [w1936]
          tunnel: w1894 -> [w1942]
          tunnel: [w1941] -> w1892
          tunnel: w1891 -> [w1940]
          tunnel: w1886 -> [w1939]
          frame #0 {
            n1355 = control-ref of="zBridge.Active Channels"() -> (w1902:refnum<vi>)
            n1356 = control-ref of="Bridge settings"() -> (w1913:refnum<vi>)
            n1357 = control-ref of="Runtime Settings"() -> (w1909:refnum<vi>)
            n1358 = control-ref of="CS Settings"() -> (w1910:refnum<vi>)
            n1359 = control-ref of="Data Logging Settings"() -> (w1911:refnum<vi>)
            n1360 = control-ref of="PID setup"() -> (w1908:refnum<vi>)
            n1361 = control-ref of="CS Cannel Names"() -> (w1906:refnum<vi>)
            n1362 = control-ref of="AVS names"() -> (w1905:refnum<vi>)
            n1363 = control-ref of="_CurCalibrations"() -> (w1903:refnum<vi>)
            n1364 = control-ref of="CS.Mode1.PID"() -> (w1901:refnum<vi>)
            n1365 = control-ref of="CS.Mode1.Settings"() -> (w1900:refnum<vi>)
            n1366 = Build Array(w1902, w1913, w1909, w1910, w1911, w1908, w1906, w1905, w1903, w1901, w1900) -> (w1915:refnum<vi>[])
            n1367 = call "FileDialog2.vi"("start path"=w1898, "pattern (all files)"="*.ini") -> ("selected path"=w1899:path)  [unwired: 10 in, 3 out]
            n1368 = call "Save Load Settings to File by Ref with path.vi"("Array of Cluster References"=w1915, "Action"=enum8{"Load", "Save"}."Load", "error in (no error)"=w1907, "Configuration file"=w1899) -> ("error out"=w1916:errorcluster)  [unwired: 5 in]
            n1369 = disable-structure shown="Disabled" {
              disable-tunnel: w1916 -> [w1919 w1924]
              disable-tunnel: [w1917 w1924] -> w1912
              frame Disabled {
                n1370 = property on="Bridge Type" class="Enum (strict)"(error in=w1919) -> (error out=w1920:errorcluster, "Value"=w1922:T61)  [unwired: 1 in, 1 out]
                n1371 = Equal To 0?(x=w1922) -> (x = 0?=w1923:bool)
                n1372 = property on="AVS GPIB Address" class="VISAName"(error in=w1920, "Visible"=w1923) -> (error out=w1921:errorcluster)  [unwired: 1 in, 1 out]
                n1373 = Not(x=w1923) -> (.not. x?=w1918:bool)
                n1374 = property on="AVS RS232 Port" class="VISAName"(error in=w1921, "Visible"=w1918) -> (error out=w1917:errorcluster)  [unwired: 1 in, 1 out]
              }
              frame Enabled {
              }
            }
          }
          frame #1 {
            n1375 = Wait (ms)(milliseconds to wait=250) -> ()  [unwired: 1 out]
          }
          frame #2 {
            n1376 = control-ref of="Sensor Calibrations"() -> (w1930:refnum<vi>)
            n1377 = control-ref of="_CurCalibrations"() -> (w1928:refnum<vi>)
            n1378 = control-ref of="Calibrations Folder"() -> (w1934:refnum<vi>)
            n1379 = control-ref of="Sensor 1"() -> (w1935:refnum<vi>)
            n1380 = control-ref of="_QuickConvertCal"() -> (w1933:refnum<vi>)
            n1381 = call "ReloadCalibrations.vi"("error in (no error)"=w1931, "Quick convert sensors"=w1933, "CurCalibrations"=w1928, "Calibration files path"=w1934, "Channel1 sensors"=w1935, "Channels list"=w1930) -> ("error out"=w1932:errorcluster)  [unwired: 1 out]
          }
          frame #3 {
            n1382 = Wait (ms)(milliseconds to wait=250) -> ()  [unwired: 1 out]
          }
          frame #4 {
            n1383 = disable-structure shown="Enabled" {
              disable-tunnel: w1942 -> [w1945 w1951]
              disable-tunnel: [w1944 w1953] -> w1941
              disable-tunnel: w1940 -> [w1943 _]
              disable-tunnel: w1939 -> [_ w1950]
              frame Enabled {
                (unwired) T77."HKEY_CURRENT_USER" ("root key (HKEY_LOCAL_MACHINE) 2")
                n1384 = control-ref of="Sensor Calibrations"() -> (w1948:refnum<vi>)
                n1385 = Build Array(w1948) -> (w1947:refnum<vi>[])
                n1386 = call "Save Load Settings to File by Ref with path.vi"("Array of Cluster References"=w1947, "subkey"="SOFTWARE\\Leiden Cryogenics\\TC" ("subkey 2"), "Action"=enum8{"Load", "Save"}."Load", "error in (no error)"=w1945, "Configuration file"=w1943) -> ("error out"=w1944:errorcluster)  [unwired: 4 in]
              }
              frame Disabled {
                n1387 = Generate User Event(user event=w1950, event data cluster="" ("event data"), error in=w1951) -> (error out=w1953:errorcluster)  [unwired: 1 in, 1 out]
              }
            }
          }
        }
        n1388 = Unbundle By Name(w1885) -> ("Config folder"=w1884:path)
      }
      event "zBridge settings": Value Change {
        # "Show parameters menu. (only for zBridge)"
        n1389 = event-data() -> ()  [unwired: 1 in, 6 out]
        n1390 = Unbundle By Name(w1956) -> ("zBridge dll"=w1954:path, "Config folder"=w1955:path)
        n1391 = disable-structure shown="Disabled" {
          disable-tunnel: w1955 -> [w1958 w1963]
          disable-tunnel: w1954 -> [w1957 w1962]
          frame Enabled {
            w1961 = 0 ("Page")
            n1392 = call "SetParFilePath.vi"("path"=w1958, "zDll"=w1957) -> ("error out"=w1959:errorcluster, "zDll out"=w1960:path)  [unwired: 8 in]
            n1393 = call "ParamMenu.vi"("error in (no error)"=w1959, "Subpage"=w1961, "Page"=w1961, "path in"=w1960) -> ()  [unwired: 6 in, 2 out]
          }
          frame Disabled {
            n1394 = call "SetParFilePath.vi"("path"=w1963, "zDll"=w1962) -> ("zDll out"=w1964:path)  [unwired: 8 in, 1 out]
            n1395 = call "zBridgeSettings_1page.vi"("zDll"=w1964) -> ()  [unwired: 10 in, 1 out]
          }
        }
      }
      event "Edit Calibrations": Value Change {
        # "Show calibration files editor. Works with .cal and .cal2 files only"
        n1396 = event-data() -> ("NewVal"=w1976:T11)  [unwired: 1 in, 5 out]
        n1397 = Unbundle By Name(w1968) -> ("UpdateCalibrations"=w1967:refnum<user-event>)
        n1398 = Cluster To Array(cluster=w1976) -> (array=w1975:bool[])
        n1399 = Unbundle By Name(w1966) -> ("Calibrations Folder"=w1965:path)
        n1400 = local read "_CurCalibrations"() -> (w1971:T33)
        n1401 = Search 1D Array(1D array=w1975, element=TRUE) -> (index of element=w1973:i32)  [unwired: 1 in]
        n1402 = Cluster To Array(cluster=w1971) -> (array=w1970:string[])
        n1403 = Index Array(array=w1970, index=w1973) -> (element=w1972:string)
        n1404 = call "Edit Calibration Coefficients.vi"("Calibration Name"=w1972, "Calibration folder"=w1965) -> ("Cancelled?"=w1969:bool)  [unwired: 1 out]
        n1405 = case shown="False" w1969 {
          tunnel: w1967 -> [w1977 _]
          frame False {
            n1406 = Generate User Event(user event=w1977, event data cluster="" ("event data")) -> ()  [unwired: 2 in, 2 out]
          }
          frame True {
          }
        }
      }
      event "Edit calibration": Value Change {
        # "Show calibration files editor for quick convert R->T. Works with .cal and .cal2 files only"
        n1407 = event-data() -> ()  [unwired: 1 in, 6 out]
        n1408 = Unbundle By Name(w1982) -> ("UpdateCalibrations"=w1981:refnum<user-event>)
        n1409 = Unbundle By Name(w1980) -> ("Calibrations Folder"=w1979:path)
        n1410 = property on="_QuickConvertCal" class="Ring (strict)"() -> ("Strings []"=w1985:string[], "Value"=w1986:u16)  [unwired: 2 in, 2 out]
        n1411 = Index Array(array=w1985, index=w1986) -> (element=w1984:string)
        n1412 = call "Edit Calibration Coefficients.vi"("Calibration Name"=w1984, "Calibration folder"=w1979) -> ("Cancelled?"=w1983:bool)  [unwired: 1 out]
        n1413 = case shown="False" w1983 {
          tunnel: w1981 -> [w1987 _]
          frame False {
            n1414 = Generate User Event(user event=w1987, event data cluster="" ("event data")) -> ()  [unwired: 2 in, 2 out]
          }
          frame True {
          }
        }
      }
      event "zBridge params.AVS Name 0", "zBridge params.AVS Name 1", "zBridge params.AVS Name 2", "zBridge params.AVS Name 3", "zBridge params.AVS Name 4", "zBridge params.AVS Name 5", "zBridge params.AVS Name 6", "zBridge params.AVS Name 7", "zBridge params.AVS Name 8", "zBridge params.AVS Name 9": Mouse Down {
        # "Show parameters menu for the channel by double clicking on \"Channel parameters\". (only for zBridge)"
        n1415 = event-data() -> ("CtlRef"=w1993:refnum<vi>, "Mods.Double Click"=w1992:bool, "PlatMods.Alt"=w1991:bool)  [unwired: 1 in, 5 out]
        n1416 = Unbundle By Name(w1990) -> ("zBridge dll"=w1989:path)
        n1417 = case shown="False" w1992 {
          tunnel: w1993 -> [w1997 w2002]
          tunnel: w1991 -> [_ w2001]
          tunnel: w1989 -> [w1994 w2000]
          frame True {
            n1418 = control-ref of="zBridge params"() -> (w1999:refnum<vi>)
            n1419 = property class="Clust (strict)"(reference=w1999) -> ("Controls[]"=w1998:refnum<vi>[])  [unwired: 1 in, 2 out]
            n1420 = Search 1D Array(1D array=w1998, element=w1997) -> (index of element=w1995:i32)  [unwired: 1 in]
            n1421 = call "ParamMenu.vi"("Subpage"=w1995, "Page"=0, "path in"=w1994) -> ()  [unwired: 7 in, 2 out]
          }
          frame False {
            n1422 = case shown="True" w2001 {
              tunnel: w2002 -> [_ w2004]
              tunnel: w2000 -> [_ w2003]
              frame False {
              }
              frame True {
                n1423 = disable-structure shown="Disabled" {
                  disable-tunnel: w2004 -> [w2007 w2011]
                  disable-tunnel: w2003 -> [w2005 _]
                  frame Disabled {
                    # "Show information window.\nTends to crash the acquisition!"
                    n1424 = control-ref of="zBridge params"() -> (w2009:refnum<vi>)
                    n1425 = property class="Clust (strict)"(reference=w2009) -> ("Controls[]"=w2008:refnum<vi>[])  [unwired: 1 in, 2 out]
                    n1426 = Search 1D Array(1D array=w2008, element=w2007) -> (index of element=w2006:i32)  [unwired: 1 in]
                    n1427 = call "Show Info Window.vi"("Data set number"=w2006, "zDll"=w2005) -> ()  [unwired: 8 in, 2 out]
                  }
                  frame Enabled {
                    # "Show information window."
                    n1428 = control-ref of="zBridge params"() -> (w2013:refnum<vi>)
                    n1429 = property class="Clust (strict)"(reference=w2013) -> ("Controls[]"=w2012:refnum<vi>[])  [unwired: 1 in, 2 out]
                    n1430 = Search 1D Array(1D array=w2012, element=w2011) -> (index of element=w2010:i32)  [unwired: 1 in]
                    n1431 = call "Scan Parameters Window.vi"("index"=w2010) -> ()  [unwired: 11 in]
                  }
                }
              }
            }
          }
        }
      }
      event "zBridge.Active Channels.active Channel 0", "zBridge.Active Channels.active Channel 1", "zBridge.Active Channels.active Channel 2", "zBridge.Active Channels.active Channel 3", "zBridge.Active Channels.active Channel 4", "zBridge.Active Channels.active Channel 5", "zBridge.Active Channels.active Channel 6", "zBridge.Active Channels.active Channel 7", "zBridge.Active Channels.active Channel 8", "zBridge.Active Channels.active Channel 9": Mouse Down {
        # "Switch channels On/Off by double clicking on \"Active\" LED. (only for zBridge and AVS47B)"
        n1432 = event-data() -> ("CtlRef"=w2018:refnum<vi>, "Mods.Double Click"=w2016:bool)  [unwired: 1 in, 6 out]
        n1433 = Unbundle By Name(w2015) -> ("zBridge dll"=w2014:path)
        n1434 = property on="Bridge Type" class="Enum (strict)"() -> ("Value"=w2017:T61)  [unwired: 2 in, 2 out]
        n1435 = case shown="True" w2016 {
          tunnel: w2018 -> [_ w2021]
          tunnel: w2017 -> [_ w2025]
          tunnel: w2014 -> [_ w2019]
          frame False {
          }
          frame True {
            n1436 = control-ref of="zBridge.Active Channels"() -> (w2024:refnum<vi>)
            n1437 = property class="Clust (strict)"(reference=w2024) -> ("Controls[]"=w2022:refnum<vi>[])  [unwired: 1 in, 2 out]
            n1438 = property class="Bool (strict)"(reference=w2021) -> ("Value"=w2020:bool)  [unwired: 1 in, 2 out]
            n1439 = Search 1D Array(1D array=w2022, element=w2021) -> (index of element=w2023:i32)  [unwired: 1 in]
            n1440 = case shown="\"Impedance Bridge\"" w2025 {
              tunnel: w2023 -> [_ w2030 w2032]
              tunnel: w2022 -> [_ w2029 _]
              tunnel: w2020 -> [_ w2026 _]
              tunnel: w2019 -> [_ _ w2031]
              frame Default {
              }
              frame "AVS47B (RS232 interface)" {
                n1441 = Index Array(array=w2029, index=w2030) -> (element=w2028:refnum<vi>)
                n1442 = Not(x=w2026) -> (.not. x?=w2027:bool)
                n1443 = property class="Ctl"(reference=w2028, "Value"=w2027) -> ()  [unwired: 1 in, 2 out]
              }
              frame "Impedance Bridge" {
                w2034 = Byte_Params."Active" ("Enum")
                # "Invert Active flag"
                n1444 = call "GetByteParam.vi"("ParNo"=w2034, "SetNo"=w2032, "zDll"=w2031) -> ("return type"=w2036:u8)  [unwired: 6 in, 2 out]
                n1445 = Decrement(x=w2036) -> (x-1=w2035:i8)
                n1446 = Absolute Value(x=w2035) -> (abs(x)=w2033:i8)
                n1447 = call "SetByteParam.vi"("SetNo"=w2032, "ParNo"=w2034, "Data"=w2033, "zDll"=w2031) -> ()  [unwired: 6 in, 2 out]
              }
            }
          }
        }
      }
      event "Small R Cluster.R0", "Small R Cluster.R1", "Small R Cluster.R2", "Small R Cluster.R3", "Small R Cluster.R4", "Small R Cluster.R5", "Small R Cluster.R6", "Small R Cluster.R7", "Small R Cluster.R8", "Small R Cluster.R9", "Small T Cluster.T0", "Small T Cluster.T1", "Small T Cluster.T2", "Small T Cluster.T3", "Small T Cluster.T4", "Small T Cluster.T5", "Small T Cluster.T6", "Small T Cluster.T7", "Small T Cluster.T8", "Small T Cluster.T9": Mouse Down {
        n1448 = event-data() -> ()  [unwired: 1 in, 8 out]
      }
      event Mouse Down {
        n1449 = event-data() -> ()  [unwired: 1 in, 8 out]
      }
      event Value Change {
        # "Update channel names on the small bottom panel when the names are changed."
        n1450 = event-data() -> ("NewVal"=→"AVS names small":T10)  [unwired: 1 in, 5 out]
      }
      event "CS.Mode1.Next": Value Change {
        # "Go to next step in CS auto mode."
        n1451 = event-data() -> ()  [unwired: 1 in, 6 out]
        n1452 = Unbundle By Name(w2044) -> ("TempStabilized"=w2043:refnum<user-event>)
        n1453 = flat-sequence {
          tunnel: w2043 -> [w2046]
          frame #0 {
            n1454 = call "Current Time(double).vi"() -> ("Current Time (double)"=w2045:dbl)  [unwired: 6 in, 1 out]
            n1455 = local write "_TimeOld"(w2045) -> ()
          }
          frame #1 {
            n1456 = Generate User Event(user event=w2046, event data cluster=TRUE ("event data")) -> ()  [unwired: 2 in, 2 out]
          }
        }
      }
      event "CS.Mode1.Auto Advance": Value Change {
        n1457 = event-data() -> ("NewVal"=w2049:bool)  [unwired: 1 in, 5 out]
        n1458 = case shown="True" w2049 {
          frame False {
          }
          frame True {
            # "Set timer to zero (01-01-1904) so the first point is set immediately, w/o wainting for time delay."
            # "If automatic mode is enabled- fire TempStabilized event to record current R,T,I values and start sweeping through TCS channels arrays"
            n1459 = disable-structure shown="Disabled" {
              frame Disabled {
                n1460 = Generate User Event(event data cluster="" ("event data")) -> ()  [unwired: 3 in, 2 out]
                "_TimeOld" <- 0.0 ("Timer")
              }
              frame Enabled {
              }
            }
          }
        }
      }
      event "CS.Mode1.Start", "CS.Mode2.Start": Value Change {
        n1461 = event-data() -> ("NewVal"=w2053:bool)  [unwired: 1 in, 5 out]
        n1462 = case shown="True" w2053 {
          frame False {
          }
          frame True {
            w2054 = TRUE
            # "Switch on the current sources."
            n1463 = property on="ON" class="Bool (strict)"() -> ("Value"=w2058:bool)  [unwired: 2 in, 2 out]
            n1464 = property on="ON" class="Bool (strict)"() -> ("Value"=w2057:bool)  [unwired: 2 in, 2 out]
            n1465 = property on="ON" class="Bool (strict)"() -> ("Value"=w2056:bool)  [unwired: 2 in, 2 out]
            n1466 = property on="ON" class="Bool (strict)"() -> ("Value"=w2055:bool)  [unwired: 2 in, 2 out]
            n1467 = Exclusive Or(1:w2058, 2:w2054) -> (0:w2062:bool)
            n1468 = Exclusive Or(1:w2057, 2:w2054) -> (0:w2060:bool)
            n1469 = Exclusive Or(1:w2056, 2:w2054) -> (0:w2059:bool)
            n1470 = Exclusive Or(1:w2055, 2:w2054) -> (0:w2061:bool)
            n1471 = property on="Toggle ON/OFF" class="Bool (strict)"("Value"=w2062) -> ()  [unwired: 2 in, 2 out]
            n1472 = property on="Toggle ON/OFF" class="Bool (strict)"("Value"=w2060) -> ()  [unwired: 2 in, 2 out]
            n1473 = property on="Toggle ON/OFF" class="Bool (strict)"("Value"=w2059) -> ()  [unwired: 2 in, 2 out]
            n1474 = property on="Toggle ON/OFF" class="Bool (strict)"("Value"=w2061) -> ()  [unwired: 2 in, 2 out]
          }
        }
      }
      event "CS.Mode1.PID.Enabled": Value Change {
        # "Enable/disable the PID loop"
        n1475 = event-data() -> ("NewVal"=w2077:bool)  [unwired: 1 in, 5 out]
        n1476 = Unbundle By Name(w2066) -> ("Reset PID loop"=w2065:refnum<user-event>)
        n1477 = call "IsDisabled.vi"("Enabled?"=w2077) -> ("Numeric"=w2080:i16)
        n1478 = Generate User Event(user event=w2065, event data cluster="" ("event data")) -> ()  [unwired: 2 in, 2 out]
        n1479 = property on="PID setup" class="Clust (strict)"("Disabled"=w2080) -> ()  [unwired: 2 in, 2 out]
        n1480 = property on="FB on" class="Enum (strict)"() -> ("Value"=w2074:enum16{"Resistance", "Temperature"})  [unwired: 2 in, 2 out]
        n1481 = property on="CS.Mode1.PID Channel" class="Enum (strict)"() -> ("Value"=w2064:enum16{"0", "1", "2", "3"})  [unwired: 2 in, 2 out]
        n1482 = property on="Enabled" class="Bool (strict)"() -> ("Value"=w2068:bool)  [unwired: 2 in, 2 out]
        n1483 = Initialize Array(FALSE, 4 ("dimension size")) -> (w2070:bool[])
        n1484 = And(x=TRUE ("new element/subarray"), y=w2068) -> (x .and. y?=w2067:bool)
        n1485 = Index Array(array=string[] ["%#_g uA", "%#_g mK"], index=w2074) -> (element=w2076:string)
        n1486 = Replace Array Subset(array=w2070, new element=w2067, index=w2064) -> (w2073:bool[])
        n1487 = local write "CS.Mode1.PID Column"(w2073) -> ()
        n1488 = Select(t=w2076, s=w2077, f="%#_g uA") -> ()  [unwired: 1 out]
      }
      event "CS.Mode1.Reset PID": Value Change {
        # "Reset the PID loop"
        n1489 = event-data() -> ()  [unwired: 1 in, 6 out]
        n1490 = Unbundle By Name(w2083) -> ("Reset PID loop"=w2082:refnum<user-event>)
        n1491 = Generate User Event(user event=w2082, event data cluster="" ("event data")) -> ()  [unwired: 2 in, 2 out]
      }
      event Value Change {
        n1492 = event-data() -> ("NewVal"=w2089:dbl)  [unwired: 1 in, 5 out]
        n1493 = Unbundle By Name(w2087) -> ("Reset PID loop"=w2086:refnum<user-event>)
        n1494 = Generate User Event(user event=w2086, event data cluster="" ("event data")) -> ()  [unwired: 2 in, 2 out]
        n1495 = property on="Enabled" class="Bool (strict)"() -> ("Value"=w2091:bool)  [unwired: 2 in, 2 out]
        n1496 = Initialize Array(FALSE, 4 ("dimension size")) -> (w2093:bool[])
        n1497 = And(x=TRUE ("new element/subarray"), y=w2091) -> (x .and. y?=w2090:bool)
        n1498 = Replace Array Subset(array=w2093, new element=w2090, index=w2089) -> (→"CS.Mode1.PID Column":bool[])
        n1499 = Index Array(array=string[] ["%#_g uA", "%#_g mK"], index=w2089) -> ()  [unwired: 1 out]
      }
      event "CS.Mode1.List": Value Change {
        n1500 = event-data() -> ("NewVal"=w2102:T23[][])  [unwired: 1 in, 5 out]
        n1501 = local read "CS.Mode1.List:Index"() -> (w2101:i32)
        n1502 = Decrement(x=w2101) -> (x-1=w2100:i32)
        n1503 = Array Size(array=w2102) -> (size(s)=w2104:i32[])
        n1504 = Index Array(array=w2104) -> (element=→"CS.Mode1.List:Count":i32)  [unwired: 1 in]
        n1505 = Index Array(array=w2102, index (row)=w2100) -> (element=→"_CSMode1List[i]":T23[])  [unwired: 1 in]
      }
      event "CS.Mode1.List": Shortcut Menu Activation? {
        n1506 = event-data() -> ()  [unwired: 1 in, 7 out]
        n1507 = event-data() -> ()  [unwired: 2 in, 1 out]
      }
      event "CS.Mode1.List": Shortcut Menu Selection (App) {
        n1508 = event-data() -> ("ItemTag"=w2107:string)  [unwired: 1 in, 7 out]
        n1509 = case shown="\"APP_SC_COPY_DATA\"" w2107 {
          frame Default {
          }
          frame "APP_SC_PASTE_DATA" {
            n1510 = invoke class="App" method="Clipboard.Read"() -> ("Read Clipbrd"=w2110:string)  [unwired: 3 in, 2 out]
            n1511 = Spreadsheet String To Array(format string="%d", spreadsheet string=w2110) -> (array=w2108:dbl[][])  [unwired: 2 in]
            n1512 = local write "CS.Mode1.List"(w2108) -> ()
          }
          frame "APP_SC_COPY_DATA" {
            n1513 = local read "CS.Mode1.List"() -> (w2113:T23[][])
            n1514 = Array To Spreadsheet String(array=w2113, 3:"%d" ("format string")) -> (spreadsheet string=w2111:string)  [unwired: 1 in]
            n1515 = invoke class="App" method="Clipboard.Write"("Param 0"=w2111) -> ()  [unwired: 3 in, 4 out]
          }
        }
      }
      event "CS.Mode1.List:To First": Value Change {
        n1516 = event-data() -> ("OldVal"=w2115:bool)  [unwired: 1 in, 5 out]
        n1517 = local write "CS.Mode1.List:To First"(w2115) -> ()
        n1518 = property on="CS.Mode1.List:Index" class="DigNum (strict)"("Val(Sgnl)"=1 ("Value (Signaling)")) -> ()  [unwired: 2 in, 2 out]
      }
      event "CS.Mode1.List:Next": Value Change {
        n1519 = event-data() -> ("OldVal"=w2118:bool)  [unwired: 1 in, 5 out]
        n1520 = local write "CS.Mode1.List:Next"(w2118) -> ()
        n1521 = local read "CS.Mode1.List:Index"() -> (w2120:i32)
        n1522 = Increment(x=w2120) -> (x+1=w2119:i32)
        n1523 = property on="CS.Mode1.List:Index" class="DigNum (strict)"("Val(Sgnl)"=w2119) -> ()  [unwired: 2 in, 2 out]
      }
      event "CS.Mode1.List:Prev": Value Change {
        n1524 = event-data() -> ("OldVal"=w2122:bool)  [unwired: 1 in, 5 out]
        n1525 = local write "CS.Mode1.List:Prev"(w2122) -> ()
        n1526 = local read "CS.Mode1.List:Index"() -> (w2124:i32)
        n1527 = Decrement(x=w2124) -> (x-1=w2123:i32)
        n1528 = property on="CS.Mode1.List:Index" class="DigNum (strict)"("Val(Sgnl)"=w2123) -> ()  [unwired: 2 in, 2 out]
      }
      event "CS.Mode1.List:Clear": Value Change {
        n1529 = event-data() -> ()  [unwired: 1 in, 6 out]
        n1530 = flat-sequence {
          frame #0 {
            n1531 = local write "CS.Mode1.List"(T23[][] [] ("I_list")) -> ()
          }
          frame #1 {
            n1532 = property on="CS.Mode1.List:To First" class="Bool (strict)"("Val(Sgnl)"=TRUE ("Value (Signaling)")) -> ()  [unwired: 2 in, 2 out]
          }
        }
      }
      event "CS.Mode1.List:Index": Value Change {
        w2149 = 10  # Lines to scroll
        n1533 = event-data() -> ("NewVal"=w2132:i32)  [unwired: 1 in, 5 out]
        n1534 = Array Size(array="CS.Mode1.List") -> (size(s)=w2135:i32[])
        n1535 = Index Array(array=w2135) -> (element=w2133:i32)  [unwired: 1 in]
        n1536 = call "Current Time(double).vi"() -> ("Current Time (double)"=w2129:dbl)  [unwired: 6 in, 1 out]
        n1537 = local write "CS.Mode1.List:Count"(w2133) -> ()
        n1538 = local write "_TimeOld"(w2129) -> ()
        n1539 = In Range and Coerce(upper limit=w2133, x=w2132, lower limit=1) -> (coerced(x)=w2130:i32)  [unwired: 1 out]
        "CS.Mode1.List:Index" <- w2130
        n1540 = Decrement(x=w2130) -> (x-1=w2131:i32)
        n1541 = Initialize Array(FALSE, w2149) -> (w2150:bool[])
        n1542 = Index Array(array="CS.Mode1.List", index (row)=w2131) -> (element=w2152:T23[])  [unwired: 1 in]
        n1543 = local write "_CSMode1List[i]"(w2152) -> ()
        n1544 = Subtract(x=w2131, y=w2149) -> (x-y=w2139:i32)
        n1545 = Increment(x=w2139) -> (x+1=w2138:i32)
        n1546 = Decrement(x=w2149) -> (x-1=w2147:i32)
        n1547 = In Range and Coerce(upper limit=inf, x=w2138, lower limit=0) -> (coerced(x)=w2137:dbl)  [unwired: 1 out]
        n1548 = In Range and Coerce(upper limit=w2147, x=w2131, lower limit=0) -> (coerced(x)=w2144:i32)  [unwired: 1 out]
        n1549 = control-ref of="CS.Mode1.List"() -> (w2142:refnum<vi>)
        n1550 = Build Array(w2137, 0 ("element")) -> (w2143:dbl[])
        n1551 = Replace Array Subset(array=w2150, new element=TRUE ("new element/subarray"), index=w2144) -> (→"CS.Mode1.Row":bool[])
        n1552 = property class="Arr (strict)"(reference=w2142, "Index Values"=w2143) -> ()  [unwired: 1 in, 2 out]
      }
      event "CS.Mode1.List:Save": Value Change {
        n1553 = event-data() -> ()  [unwired: 1 in, 6 out]
        n1554 = call "File Dialog6"() -> ("selected path"=w2156:path, "cancelled"=w2155:bool)  [unwired: 12 in, 2 out]
        n1555 = case shown="False" w2155 {
          tunnel: w2156 -> [w2157 _]
          frame False {
            n1556 = local read "CS.Mode1.List"() -> (w2159:T23[][])
            n1557 = call <vilib>:"Write To Spreadsheet File (DBL).vi"("format (%.3f)"="%.1f", "2D data"=w2159, "file path (dialog if empty)"=w2157) -> ()  [unwired: 5 in, 1 out]
          }
          frame True {
          }
        }
      }
      event "CS.Mode1.List:Load": Value Change {
        n1558 = event-data() -> ()  [unwired: 1 in, 6 out]
        n1559 = call "File Dialog5"() -> ("selected path"=w2161:path, "cancelled"=w2162:bool)  [unwired: 12 in, 2 out]
        n1560 = case shown="False" w2162 {
          tunnel: w2161 -> [w2163 _]
          frame False {
            n1561 = call <vilib>:"Read From Spreadsheet File (DBL).vi"("file path (dialog if empty)"=w2163) -> ("all rows"=w2164:dbl[][])  [unwired: 6 in, 4 out]
            n1562 = local write "CS.Mode1.List"(w2164) -> ()
          }
          frame True {
          }
        }
      }
      event "CS.Mode1.Write To Log": Value Change {
        n1563 = event-data() -> ()  [unwired: 1 in, 6 out]
        n1564 = Unbundle By Name(w2167) -> ("TempStabilized"=w2166:refnum<user-event>)
        n1565 = Generate User Event(user event=w2166, event data cluster=FALSE ("event data")) -> ()  [unwired: 2 in, 2 out]
      }
      event "CS.Mode2.Add Row": Value Change {
        n1566 = event-data() -> ()  [unwired: 1 in, 6 out]
        n1567 = call "Currents-Temp list  - add new range.vi"("List in"="CS.Mode2.List", "Array"="CS.Mode2.New Row") -> ("Sorted list out"=w2171:dbl[][])  [unwired: 3 in, 1 out]
        n1568 = local write "CS.Mode2.List"(w2171) -> ()
      }
      event "CS.Mode2.List": Shortcut Menu Selection (User) {
        n1569 = event-data() -> ("CtlRef"=w2176:refnum<vi>, "Coords"=w2175:T72, "ItemPath"=w2174:string)  [unwired: 1 in]
        n1570 = case shown="\"Erase Range\"" w2174 {
          tunnel: w2176 -> [_ w2182 _ w2188 w2189]
          tunnel: w2175 -> [_ w2181 _ _ _]
          frame Default {
          }
          frame "Erase Range" {
            (unwired) TRUE
            n1571 = call "Get Clicked Array Index.vi"("Coords"=w2181, "Array in"=w2182) -> ("Clicked Index"=w2178:i32[])  [unwired: 6 in, 3 out]
            n1572 = local read "CS.Mode2.List"() -> (w2180:dbl[][])
            n1573 = Index Array(array=w2178) -> (element=w2177:i32)  [unwired: 1 in]
            n1574 = call "Currents-Temp list - delete range.vi"("Numeric"=w2177, "I_list 2"=w2180) -> ("I_list"=w2179:dbl[][])  [unwired: 2 in]
            n1575 = local write "CS.Mode2.List"(w2179) -> ()
          }
          frame "Clear List" {
            n1576 = call "Currents-Temp list - check ranges.vi"() -> ("I_list out"=w2183:dbl[][])  [unwired: 5 in]
            n1577 = local write "CS.Mode2.List"(w2183) -> ()
          }
          frame "Copy Data" {
            n1578 = property class="Arr (strict)"(reference=w2188) -> ("Value"=w2184:dbl[][])  [unwired: 1 in, 2 out]
            n1579 = Array To Spreadsheet String(delimiter (Tab)="\t", array=w2184, 3:"%.4g" ("format string")) -> (spreadsheet string=w2187:string)
            n1580 = invoke class="App" method="Clipboard.Write"("Param 0"=w2187) -> ()  [unwired: 3 in, 4 out]
          }
          frame "Paste Data" {
            n1581 = invoke class="App" method="Clipboard.Read"() -> ("Read Clipbrd"=w2190:string)  [unwired: 3 in, 2 out]
            n1582 = Spreadsheet String To Array(delimiter (Tab)="\t", format string="%.4g", spreadsheet string=w2190) -> (array=w2193:dbl[][])  [unwired: 1 in]
            n1583 = property class="Arr (strict)"(reference=w2189, "Value"=w2193) -> ()  [unwired: 1 in, 2 out]
          }
        }
      }
      event "Graph-open popup": Value Change {
        w2206 = 128  # call and forget
        n1584 = event-data() -> ()  [unwired: 1 in, 6 out]
        n1585 = vi-ref "Graph popup.vi"() -> (w2202:refnum<vi>)
        n1586 = property class="VI"(reference=w2202) -> (error out=w2204:errorcluster, "Name"=w2205:string)  [unwired: 1 in, 1 out]
        n1587 = local read "Sensor Names"() -> (w2195:T10)
        n1588 = Open VI Reference(type specifier VI Refnum (for type only)=refnum<vi> refnum, vi path=w2205, options=w2206, error in (no error)=w2204) -> (vi reference=w2203:refnum<vi>, error out=w2198:errorcluster)  [unwired: 2 in]
        n1589 = control-ref of="Data"() -> (w2200:refnum<vi>)
        n1590 = Cluster To Array(cluster=w2195) -> (array=w2194:string[])
        n1591 = call-by-ref "Start Asynchronous Call"(reference=w2203, error in=w2198, "Data"=w2200, "Channel Names"=w2194) -> (reference out=w2199:refnum<vi>, error out=w2197:errorcluster)  [unwired: 18 in]
        n1592 = Close Reference(reference=w2199, error in (no error)=w2197) -> ()  [unwired: 1 out]
      }
      event "ColorBox": Mouse Move {
        n1593 = event-data() -> ("Coords"=w2210:T72)  [unwired: 1 in]
        n1594 = call <vilib>:"Picture to Pixmap.vi"("picture"="Colors") -> ("image data"=w2216:T71)  [unwired: 9 in, 1 out]
        n1595 = property on="Colors" class="Pict"() -> ("Position"=w2209:T79)  [unwired: 2 in, 2 out]
        n1596 = call <vilib>:"Unflatten Pixmap.vi"("image data"=w2216) -> ("24-bit pixmap"=w2211:u32[][])  [unwired: 4 in, 6 out]
        n1597 = Subtract(x=w2210, y=w2209) -> (x-y=w2214:T72)
        n1598 = Unbundle(w2214) -> ("Horizontal"=w2213:i32, "Vertical"=w2212:i32)
        n1599 = Index Array(array=w2211, index (row)=w2212, index (col)=w2213) -> (element=→"Color":u32)
      }
      event "ColorBox": Mouse Down {
        n1600 = event-data() -> ()  [unwired: 1 in, 8 out]
        n1601 = property on="ColorBox" class="TabCtl (strict)"("Visible"=FALSE) -> ()  [unwired: 2 in, 2 out]
      }
      event "Set Color": Value Change {
        n1602 = event-data() -> ()  [unwired: 1 in, 6 out]
        n1603 = property on="ColorBox" class="TabCtl (strict)"("Visible"=TRUE) -> ()  [unwired: 2 in, 2 out]
      }
    }
    "General Error" <- w74
  }
  n1604 = flat-sequence {
    tunnel: w38 -> [w2221]
    frame #0 {
      n1605 = Wait on Occurrence(2:w2221) -> ()  [unwired: 2 in, 1 out]
    }
    frame #1 {
      n1606 = while {
        i -> [w2232]
        stop <- "Stop" stop-if-true
        # "AVS/zBridge read-out"
        n1607 = case shown="False" "Pause" {
          tunnel: w2232 -> [w2241 _]
          frame False {
            # "For the first measurement set Stab.Time=12 s to do autoranging"
            n1608 = local read "zBridge.Active Channels"() -> (w2246:T21)
            n1609 = property on="Runtime Settings" class="Clust (strict)"() -> ("Value"=w2260:T27)  [unwired: 2 in, 2 out]
            n1610 = Unbundle By Name(w2260) -> ("Stabilisation Delay"=w2253:dbl, "Averages"=w2247:u16, "Last Channel"=w2259:i8, "Read AVS channels from"=w2258:i8)
            n1611 = Unbundle By Name("Bridge settings") -> ("Picobus Delay"=w2235:u32, "Sync to ADC"=w2236:enum16{"FALSE", "TRUE"}, "Bridge Type"=w2238:T61)
            n1612 = call "Split Exc&Range.vi"("Excitations 2"="AVS Exc&Ranges") -> ("Excitations"=w2239:T29, "Ranges"=w2240:T80)  [unwired: 4 in]
            n1613 = Cluster To Array(cluster=w2246) -> (array=w2245:bool[])
            n1614 = property on="_AVS_VISA" class="VISAName"() -> ("Value"=w2257:refnum<visa-resource-name>)  [unwired: 2 in, 2 out]
            n1615 = call "If First Iteration.vi"("Iteration"=w2241, "Value In"=w2253, "Default"=12.0) -> ("Value Out"=w2252:dbl)
            n1616 = case shown="\"AVS47B (RS232 interface)\"" w2238 {
              tunnel: w2257 -> [w2270 w2283 _ _ _]
              tunnel: w2252 -> [w2266 w2286 w2293 _ _]
              tunnel: w2247 -> [w2267 w2285 _ _ _]
              tunnel: w2259 -> [w2268 w2281 _ _ _]
              tunnel: w2258 -> [w2269 w2282 _ _ _]
              tunnel: w2239 -> [w2271 w2277 _ _ _]
              tunnel: [w2263 w2276 errorcluster {"status"=FALSE, "code"=0, "source"=""} ("error out") w2309 errorcluster {"status"=FALSE, "code"=0, "source"=""} ("error out")] -> w2250
              tunnel: w2240 -> [w2265 w2279 w2294 w2310 w2314]
              tunnel: TRUE ("Autorange") -> [w2261 w2280 _ _ _]
              tunnel: [w2264 w2278 w2294 w2310 w2314] -> w2244
              tunnel: [w2262 w2275 w2292 w2303 dbl[] [] ("Data array")] -> w2248
              tunnel: w2245 -> [_ w2274 _ _ _]
              tunnel: "_ScanData" -> [_ _ _ w2299 _]
              tunnel: w2236 -> [_ w2273 _ _ _]
              tunnel: w2235 -> [_ w2272 _ _ _]
              frame "AVS47A (GPIB interface)" {
                # "AVS 47 (GPIB)"
                n1617 = call "AVS47IB_do_single_scan.vi"("AVS Port"=w2270, "Stabilization Delay"=w2266, "Autorange"=w2261, "Number of Averages"=w2267, "Last Channel"=w2268, "First Channel"=w2269, "Excitations"=w2271, "Ranges"=w2265) -> ("error out"=w2263:errorcluster, "R"=w2262:dbl[], "Ranges"=w2264:T81)  [unwired: 3 in, 2 out]
              }
              frame "AVS47B (RS232 interface)" {
                # "AVS 47B (RS232)"
                n1618 = Type Cast(type=refnum<visa-resource-name> refnum ("dup VISA session"), x=w2283) -> (*(type *) &x=w2287:refnum<visa-resource-name>)
                n1619 = call "Scanner.vi"("STABILIZATION  DELAY"=w2286, "AVERAGE COUNT"=w2285, "Excitation"=w2277, "Range"=w2279, "VISA resource"=w2287, "FIRST CH TO SCAN"=w2282, "PICOBUS DELAY"=w2272, "SYNCHRONIZE TO ADC"=w2273, "LAST CH TO SCAN"=w2281, "array"=w2274, "Autorange"=w2280) -> ("error out 2"=w2276:errorcluster, "RI"=w2275:dbl[], "Range out"=w2278:T82)  [unwired: 11 in, 3 out]
              }
              frame "AVS Emulation" {
                (unwired) dbl[] [0.0, 0.0, 0.0, 0.0] ("I")
                n1620 = local read "CS.Automode Current"() -> (w2290:T23[])
                n1621 = Multiply(x=w2293, y=u32 1000 ("milliseconds to wait")) -> (x*y=w2297:dbl)
                n1622 = Wait (ms)(milliseconds to wait=w2297) -> ()  [unwired: 1 out]
                n1623 = Index Array(array=w2290, index=3) -> ()  [unwired: 1 out]
                n1624 = property on="CS.Current Value" class="Arr (strict)"() -> ("Value"=w2296:dbl[])  [unwired: 2 in, 2 out]
                n1625 = Multiply(x=1000.0, y=w2296) -> (x*y=w2288:dbl[])
                n1626 = call "AVS Emulate.vi"("Currents"=w2288, "Sampling time"=w2293) -> ("R"=w2292:dbl[])  [unwired: 1 in, 1 out]
              }
              frame "Impedance Bridge" {
                n1627 = local read "Bridge status"() -> (w2304:errorcluster)
                n1628 = local read "_zBridgeDll"() -> (w2311:path)
                n1629 = call "Read Data from Single Channel.vi"("error in (no error)"=w2304, "zDll"=w2311) -> ("error out"=w2309:errorcluster, "Value"=w2308:dbl, "Scan parameters/Error string"=→"_zBridgeParText":string, "Set number"=w2301:u8, "Error code"=→"Error code":u8, "Unit"=→"_ZBridgeUnit":string, "ScanParameters out"=w2302:T83)  [unwired: 3 in]
                "_zBridgeSetNr" <- w2301
                n1630 = call "ScanParameters FGV.vi"("Action"=Action."Write", "index"=w2301, "ScanParameters in"=w2302) -> ()  [unwired: 8 in, 1 out]
                n1631 = Replace Array Subset(array=w2299, new element=w2308, index=w2301) -> (w2303:dbl[])
              }
              frame "Disabled", Default {
              }
            }
            "Bridge status" <- w2250
            n1632 = property on="_AVSRanges" class="Clust (strict)"("Val(Sgnl)"=w2244) -> ()  [unwired: 2 in, 2 out]
            n1633 = property on="_ScanData" class="Arr (strict)"("Val(Sgnl)"=w2248) -> ()  [unwired: 2 in, 2 out]
            n1634 = property on="Delay" class="DigNum (strict)"() -> ("Value"=w2243:u32)  [unwired: 2 in, 2 out]
            n1635 = Multiply(x=u32 1000, y=w2243) -> (x*y=w2256:u32)
            n1636 = Wait (ms)(milliseconds to wait=w2256) -> ()  [unwired: 1 out]
          }
          frame True {
          }
        }
      }
      n1637 = while {
        stop <- w2316 stop-if-true
        (unwired) errorcluster {"status"=FALSE, "code"=0, "source"=""} ("Value")
        # "Current source control"
        n1638 = property on="CS status" class="Clust (strict)"() -> ("Value"=w2315:errorcluster)  [unwired: 2 in, 2 out]
        n1639 = stacked-sequence {
          seq-local: [w2344 _ _ _] -> [_ w2353 _ _]
          seq-local: [w2343 _ _ _] -> [_ w2352 _ _]
          seq-local: [_ w2353 _ _] -> [_ _ w2363 _]
          seq-local: [_ w2351 _ _] -> [_ _ w2362 _]
          tunnel: w2315 -> [w2342 _ _ _]
          frame #0 {
            # "Write 0 instead of the actual \ncurrent value to log if there \nis no current flowing."
            # "Read current CS status"
            n1640 = local read "_CSClassRef"() -> (w2332:refnum<class "CS.lvclass">)
            n1641 = call-dynamic "Read.vi"("CS in"=w2332, "error in (no error)"=w2342, "Optional"=FALSE) -> ("CS out"=w2344:refnum<class "CS.lvclass">, "I0"=w2335:T84, "I1"=w2336:T84, "I2"=w2337:T84, "I3"=w2338:T84, "error out"=w2343:errorcluster)  [unwired: 11 in]
            n1642 = Unbundle By Name(w2335) -> ("Current (string)"=w2330:string, "I?"=w2329:bool)
            n1643 = Unbundle By Name(w2336) -> ("Current (string)"=w2345:string, "I?"=w2328:bool)
            n1644 = Unbundle By Name(w2337) -> ("Current (string)"=w2333:string, "I?"=w2327:bool)
            n1645 = Unbundle By Name(w2338) -> ("Current (string)"=w2346:string, "I?"=w2326:bool)
            n1646 = call "CS Data Converter.vi"("CS Data"=w2335) -> ("CS Indicator"=→"I0":T85)
            n1647 = call "CS Data Converter.vi"("CS Data"=w2336) -> ("CS Indicator"=→"I1":T85)
            n1648 = call "CS Data Converter.vi"("CS Data"=w2337) -> ("CS Indicator"=→"I2":T85)
            n1649 = call "CS Data Converter.vi"("CS Data"=w2338) -> ("CS Indicator"=→"I3":T85)
            n1650 = Fract/Exp String To Number(string=w2330) -> (number=w2334:dbl)  [unwired: 3 in, 1 out]
            n1651 = Fract/Exp String To Number(string=w2345) -> (number=w2341:dbl)  [unwired: 3 in, 1 out]
            n1652 = Fract/Exp String To Number(string=w2333) -> (number=w2340:dbl)  [unwired: 3 in, 1 out]
            n1653 = Fract/Exp String To Number(string=w2346) -> (number=w2339:dbl)  [unwired: 3 in, 1 out]
            n1654 = Build Array(w2329, w2328, w2327, w2326) -> (w2325:bool[])
            n1655 = Not(x=w2325) -> (.not. x?=w2321:bool[])
            n1656 = Build Array(w2334, w2341, w2340, w2339) -> (w2324:dbl[])
            "CS.Current Value" <- w2324
            n1657 = for {
              tunnel: w2321 -> [w2350] mode=indexing
              tunnel: w2324 -> [w2349] mode=indexing
              tunnel: dbl[] [0.0, 0.0, 0.0, 0.0] ("t") -> [w2348] mode=indexing
              tunnel: [w2347] -> w2322 mode=indexing
              n1658 = Select(t=w2348, s=w2350, f=w2349) -> (s? t:f=w2347:dbl)
            }
            "CS.Actual Current" <- w2322
          }
          frame #1 {
            n1659 = Wait (ms)(milliseconds to wait=100) -> ()  [unwired: 1 out]
            n1660 = call <vilib>:"Clear Errors.vi"("error in (no error)"=w2352) -> ("error out"=w2351:errorcluster)  [unwired: 5 in, 1 out]
          }
          frame #2 {
            # "Only send data to CS if\nnew value was entered"
            # "Set CS status"
            n1661 = call "CS OnOff & Gated and Current & Range.vi"("I in"="CS.I0") -> ("OnOff & Gated"=w2374:T86, "Current & Range"=w2359:T87, "I out"=w2367:T88)  [unwired: 2 in]
            n1662 = call "CS OnOff & Gated and Current & Range.vi"("I in"="CS.I1") -> ("OnOff & Gated"=w2373:T86, "Current & Range"=w2358:T87, "I out"=w2364:T88)  [unwired: 2 in]
            n1663 = call "CS OnOff & Gated and Current & Range.vi"("I in"="CS.I2") -> ("OnOff & Gated"=w2370:T86, "Current & Range"=w2357:T87, "I out"=w2365:T88)  [unwired: 2 in]
            n1664 = call "CS OnOff & Gated and Current & Range.vi"("I in"="CS.I3") -> ("OnOff & Gated"=w2369:T86, "Current & Range"=w2356:T87, "I out"=w2366:T88)  [unwired: 2 in]
            n1665 = local write "CS.I0"(w2367) -> ()
            n1666 = local write "CS.I1"(w2364) -> ()
            n1667 = local write "CS.I2"(w2365) -> ()
            n1668 = local write "CS.I3"(w2366) -> ()
            n1669 = local read "CS.Automode Current"() -> (w2355:T23[])
            n1670 = Equal To 0?(x="CS.Mode") -> (x = 0?=w2360:bool)
            n1671 = call "CS_set_channels.vi"("CS in"=w2363, "Current & Range0"=w2359, "Current & Range1"=w2358, "Current & Range 2"=w2357, "Current & Range3"=w2356, "error out"=w2362, "I_automode"=w2355, "Auto?"=w2360) -> ("CS.lvclass out"=w2379:refnum<class "CS.lvclass">, "Current Changed?"=w2376:bool, "error out 2"=w2380:errorcluster)  [unwired: 9 in]
            n1672 = call-dynamic "Set Mode.vi"("CS.lvclass in"=w2379, "On&G 0"=w2374, "On&G 1"=w2373, "On&G 2"=w2370, "On&G 3"=w2369, "error in (no error)"=w2380) -> ("CS.lvclass out"=w2377:refnum<class "CS.lvclass">, "error out"=w2378:errorcluster)  [unwired: 12 in]
            n1673 = case shown="True" w2376 {
              selector: w2376 -> [_ w2381]
              frame False {
              }
              frame True {
                n1674 = property on="_CurrentsChanged" class="Bool (strict)"("Val(Sgnl)"=w2381) -> ()  [unwired: 2 in, 2 out]
              }
            }
            n1675 = local write "_CSClassRef"(w2377) -> ()
            n1676 = property on="CS status" class="Clust (strict)"("Value"=w2378) -> ()  [unwired: 2 in, 2 out]
          }
          frame #3 {
            n1677 = Wait (ms)(milliseconds to wait=100) -> ()  [unwired: 1 out]
          }
        }
        n1678 = local read "Stop"() -> (w2316:bool)
      }
      n1679 = while {
        stop <- w2224 stop-if-true
        # "zBridge status read-out"
        n1680 = property on="Bridge Type" class="Enum (strict)"() -> ("Value"=w2222:T61)  [unwired: 2 in, 2 out]
        n1681 = case shown="Default" w2222 {
          frame Default {
          }
          frame "Impedance Bridge" {
            n1682 = local read "_zBridgeDll"() -> (w2230:path)
            n1683 = local read "Bridge status"() -> (w2229:errorcluster)
            n1684 = call "ScanStatus.vi"("error in (no error)"=w2229, "zDll"=w2230) -> ("error out"=w2228:errorcluster, "Status"=w2225:i32, "Channel"=w2226:i32)  [unwired: 6 in, 1 out]
            n1685 = local write "Bridge status"(w2228) -> ()
            n1686 = call "zBridge Format Status.vi"("Status"=w2225, "Channel"=w2226) -> ("Status"=→"zBridge.Scan Phase":T89, "Active channel"=→"zBridge.Active channel":T90)  [unwired: 2 in]
          }
        }
        n1687 = Wait (ms)(milliseconds to wait=u32 200) -> ()  [unwired: 1 out]
        n1688 = local read "Stop"() -> (w2224:bool)
      }
    }
  }
  n1689 = disable-structure shown="Disabled" {
    frame Disabled {
      w2396 = string[] ["Paste Data from Clipboard"] ("item names")
      (unwired) enum32{"Page 1"}."Page 1" ("Tab Control 4")
      n1690 = local read "CS.Automode Current"() -> (w2391:T23[])
      n1691 = local read "zBridge.Active Channels"() -> ()  [unwired: 1 in]
      n1692 = property on="Bridge Channel" class="DigNum (strict)"() -> ("Value"=w2384:i32)  [unwired: 2 in, 2 out]
      n1693 = local read item#-1() -> ()  [unwired: 1 out]
      n1694 = Index Array(array=w2391) -> (element #1=w2387:T23, element #2=w2388:T23, element #3=w2389:T23, element #4=w2390:T23)  [unwired: 4 in]
      n1695 = property class="XYGraph (strict)" props=["YScale", "Mapping Mode"]() -> ()  [unwired: 2 in, 3 out]
      n1696 = property on="I" class="DigNum (strict)"("Val(Sgnl)"=w2387) -> ()  [unwired: 2 in, 2 out]
      n1697 = property on="I" class="DigNum (strict)"("Val(Sgnl)"=w2388) -> ()  [unwired: 2 in, 2 out]
      n1698 = property on="I" class="DigNum (strict)"("Val(Sgnl)"=w2389) -> ()  [unwired: 2 in, 2 out]
      n1699 = property on="I" class="DigNum (strict)"("Val(Sgnl)"=w2390) -> ()  [unwired: 2 in, 2 out]
      n1700 = Insert Menu Items(4:4, 7:w2396, 8:w2396) -> ()  [unwired: 3 in, 3 out]
      n1701 = Equal?(y=w2384) -> (x = y?=w2383:bool)  [unwired: 1 in]
      n1702 = Equal?(x=w2384, y=-1) -> (x = y?=w2386:bool)
      n1703 = Or(x=w2383, y=w2386) -> ()  [unwired: 1 out]
      n1704 = property on="ON" class="Boolean (strict)"() -> ("Value"=w2403:bool)  [unwired: 2 in, 2 out]
      n1705 = control-ref of="zBridge.Active Channels"() -> ()  [unwired: 1 out]
      n1706 = Exclusive Or(1:w2403, 2:TRUE ("x")) -> (0:w2402:bool)
      n1707 = property on="Toggle ON/OFF" class="Bool (strict)"("Value"=w2402) -> ()  [unwired: 2 in, 2 out]
      n1708 = control-ref of="CS.Mode1.List"() -> (w2398:refnum<vi>)
      n1709 = property class="Arr (strict)"(reference=w2398) -> ("Index Values"=w2399:u32[])  [unwired: 1 in, 2 out]
      n1710 = Index Array(array=w2399) -> (element=w2400:u32)  [unwired: 1 in]
      n1711 = property on="Side Panel" class="TabCtl (strict)"() -> ("Pages"=w2404:refnum<vi>[])  [unwired: 2 in, 2 out]
      n1712 = property on="CS.Mode1.List:Index" class="DigNum (strict)"("Val(Sgnl)"=w2400) -> ()  [unwired: 2 in, 2 out]
      n1713 = Index Array(array=w2404, index=1) -> (element=w2405:refnum<vi>)
      n1714 = Generate User Event(event data cluster="" ("event data")) -> ()  [unwired: 3 in, 2 out]
      n1715 = property class="Page"(reference=w2405, "PageVis"=TRUE ("Page Visible")) -> ()  [unwired: 1 in, 2 out]
      n1716 = property on="FB on" class="Enum (strict)" props=["Value"]() -> ()  [unwired: 2 in, 3 out]
      n1717 = Initialize Array(0.0 ("element"), 4 ("dimension size")) -> (w2392:dbl[])
      n1718 = local write "CS.Automode Current"(w2392) -> ()
    }
    frame Enabled {
    }
  }
